vi "Lambda_Test_RT.vi"() -> ()   [LabVIEW 2014]
uses:
  <vilib>/rvi/interface/nirviOpenFPGA/nirviOpenFPGA.xnode
  <vilib>/rvi/interface/nirviReadWriteControl/nirviReadWriteControl.xnode
  <vilib>/Platform/TimedLoop/XDataNode/XDataNode.xnode
  <vilib>/Platform/TimedLoop/XDataNode/nitl_modes.ctl
  <vilib>/Platform/TimedLoop/XDataNode/XDNodeRunTimeDep.lvlib
  <vilib>/Platform/TimedLoop/XDataNode/wakeup.ctl
  <vilib>/Platform/TimedLoop/XDataNode/timing_clust.ctl
  <vilib>/addons/control/pid/NI_PID_pid.lvlib
  <vilib>/rvi/errors/niLvFpgaAdjustHostInterfaceError.vi
  <vilib>/rvi/interface/nirviCloseFPGA/nirviCloseFPGA.xnode
  <vilib>/addons/control/pid/pid.llb/PID (DBL).vi
  NiFpgaLv.dll
  <vilib>/Utility/error.llb/Error Cluster From Error Code.vi
  FPGA main v06-01.vi
  FPGA Bitfiles/MAXCAT_FPGATarget5_FPGAmainv06-01_qYdUsd75oPc.lvbitx
  FPGA 9146 v160610.vi
  <vilib>/FPGAPlugInAG/cRIO-9067/niLvFpga_Open_cRIO-9067.vi
  <vilib>/FPGAPlugInAG/cRIO-9067/niLvFpga_Close_cRIO-9067.vi
panel:
  in  "HC Fact HCLO":dbl
  in  "HC Base HCLO":dbl
  in  "O2 Base HCLO":dbl
  in  "O2 Fact HCLO":dbl
  in  "Heat Load Control":T1(radio)
  in  "Reset Heat Load 4":bool
  out "% Complete 4":dbl
  out "Complete 4":dbl(slide) scale=0.0..100.0
  out "Remaining Time 4":dbl format="%<%H:%M:%S>t"
  out "Ageing Time 4":dbl format="%<%H:%M:%S>t"
  in  "Reset Heat Load 3":bool
  out "% Complete 3":dbl
  out "Complete 3":dbl(slide) scale=0.0..100.0
  out "Remaining Time 3":dbl format="%<%H:%M:%S>t"
  out "Ageing Time 3":dbl format="%<%H:%M:%S>t"
  out "UEGO Array":dbl[](array[numeric])
  in  "UEGO 3":i64=200
  out "UEGO Sensor Results 2":T2
  in  "SensorControl 2":T3={"UEGO1Enable"=FALSE, "UEGO2Enable"=FALSE, "EGO1Enable"=FALSE, "EGO2Enable"=FALSE, "EGO3Enable"=FALSE, "EGO4Enable"=FALSE, "UEGO1Range"=FALSE, "UEGO2Range"=FALSE, "FilterCutoff (Hz)"=10.0}
  in  "UEGO Back Pressure (bar) 3":T4={"UEGO1BackPressure (bar)"=1.013, "UEGO2BackPressure (bar)"=1.013}
  in  "UEGOModuleEnable 3":bool
  out "UEGO Heater (V) 2":T5
  out "UEGO Diagnostics 3":T6={"ModulePresent"=FALSE, "UEGO1SensorFault"=63, "UEGO2SensorFault"=63, "UEGO1HeaterFault"=192, "UEGO2HeaterFault"=192, "UEGOFuseStatus"=0, "Battery (V)"=0.0, "LSUType"=0} {"LSUType" items=["LSU 4.9", "LSU 4.2"]; "UEGOFuseStatus" items=["FUSE OK", "FUSE BLOWN"]; "UEGO2SensorFault" items=["NO FAULT"=63, "SHORT TO GND OR BATT"=0]; "UEGO2HeaterFault" items=["SHORT TO GROUND"=0, "OPEN CIRCUIT"=64, "SHORT TO BATTERY"=128, "NO FAULT"=192]; "UEGO1SensorFault" items=["NO FAULT"=63, "SHORT TO GND OR BATT"=0]; "UEGO1HeaterFault" items=["SHORT TO GROUND"=0, "OPEN CIRCUIT"=64, "SHORT TO BATTERY"=128, "NO FAULT"=192]}
  out "UEGO Temperature (C) 2":T7
  in  "Start Test":bool
  out "Ready":bool
  out "UEGO Sensor Results":T2
  in  "SensorControl":T3={"UEGO1Enable"=FALSE, "UEGO2Enable"=FALSE, "EGO1Enable"=FALSE, "EGO2Enable"=FALSE, "EGO3Enable"=FALSE, "EGO4Enable"=FALSE, "UEGO1Range"=FALSE, "UEGO2Range"=FALSE, "FilterCutoff (Hz)"=10.0}
  in  "UEGO Back Pressure (bar)":T4={"UEGO1BackPressure (bar)"=1.013, "UEGO2BackPressure (bar)"=1.013}
  in  "UEGOModuleEnable":bool
  out "UEGO Heater (V)":T5
  out "UEGO Diagnostics":T6={"ModulePresent"=FALSE, "UEGO1SensorFault"=63, "UEGO2SensorFault"=63, "UEGO1HeaterFault"=192, "UEGO2HeaterFault"=192, "UEGOFuseStatus"=0, "Battery (V)"=0.0, "LSUType"=0} {"LSUType" items=["LSU 4.9", "LSU 4.2"]; "UEGOFuseStatus" items=["FUSE OK", "FUSE BLOWN"]; "UEGO2SensorFault" items=["NO FAULT"=63, "SHORT TO GND OR BATT"=0]; "UEGO2HeaterFault" items=["SHORT TO GROUND"=0, "OPEN CIRCUIT"=64, "SHORT TO BATTERY"=128, "NO FAULT"=192]; "UEGO1SensorFault" items=["NO FAULT"=63, "SHORT TO GND OR BATT"=0]; "UEGO1HeaterFault" items=["SHORT TO GROUND"=0, "OPEN CIRCUIT"=64, "SHORT TO BATTERY"=128, "NO FAULT"=192]}
  out "UEGO Temperature (C)":T7
  in  "Reset Heat Load 2":bool
  out "% Complete 2":dbl
  out "Complete 2":dbl(slide) scale=0.0..100.0
  out "Remaining Time 2":dbl format="%<%H:%M:%S>t"
  out "Ageing Time 2":dbl format="%<%H:%M:%S>t"
  in  "Pressure Transducer 2":enum32{"Druck ", "FUJI ", "Impress"}(radio)
  in  "Pressure Transducer 1":enum32{"Druck ", "FUJI ", "Impress"}(radio)
  out "UEGO Diagnostics 2":T8={"ModulePresent"=FALSE, "UEGO1SensorFault"=63, "UEGO2SensorFault"=63, "UEGO1HeaterFault"=192, "UEGO2HeaterFault"=192, "UEGOFuseStatus"=0, "Battery (V)"=0.0} {"UEGOFuseStatus" items=["FUSE OK", "FUSE BLOWN"]; "UEGO2SensorFault" items=["NO FAULT"=63, "SHORT TO GND OR BATT"=0]; "UEGO2HeaterFault" items=["SHORT TO GROUND"=0, "OPEN CIRCUIT"=64, "SHORT TO BATTERY"=128, "NO FAULT"=192]; "UEGO1SensorFault" items=["NO FAULT"=63, "SHORT TO GND OR BATT"=0]; "UEGO1HeaterFault" items=["SHORT TO GROUND"=0, "OPEN CIRCUIT"=64, "SHORT TO BATTERY"=128, "NO FAULT"=192]}
  in  "V Max Flow":sgl=10.0 format="%.3f"
  out "Press Time":i32
  out "Valve 2 Position":dbl
  out "Valve 1 Position":dbl
  in  "Valve 2 SP":dbl=1.0
  in  "Valve 1 SP":dbl=1.0
  out "Uego Avg":dbl
  in  "Press Up Limit":sgl=5.0
  in  "Press Low Limit":sgl
  out "Loop No.":i32
  in  "UEGO 1":i64=200
  in  "UEGO 2":i64=200
  in  "UEGOModuleEnable 2":bool=TRUE
  in  "UEGO Back Pressure (bar) 2":T4={"UEGO1BackPressure (bar)"=1.013, "UEGO2BackPressure (bar)"=1.013}
  in  "SensorEnable 2":T9={"UEGO1Enable"=TRUE, "UEGO2Enable"=TRUE, "EGO1Enable"=TRUE, "EGO2Enable"=TRUE, "EGO3Enable"=TRUE, "EGO4Enable"=TRUE}
  out "UEGO Meas 2":T2
  out "Pressure":dbl(graph)
  out "HC-2":bool
  out "AIR-2":bool
  out "HC-B":bool
  out "AIR-B":bool
  out "NO":bool
  out "AIR-1":bool
  out "HC-1":bool
  out "CO":bool
  in  "NO Factor":dbl
  in  "CO Factor":dbl
  in  "Set-point Fan":dbl
  in  "Fan PID":bool
  in  "Furnace 1":dbl=2.0
  in  "Furnace 2":dbl=2.0
  in  "Furnace Manual Mode":bool
  in  "Reset Heat Load":bool
  in  "Mop-up Lambda Control":bool
  in  "Lambda SP 3":dbl
  in  "Output Low 3":dbl
  in  "Output High 3":dbl
  in  "PID Mop-up Catalyst":T10={"proportional gain (Kc)"=0.8, "integral time (Ti, min)"=0.8, "derivative time (Td, min)"=0.0}
  in  "PID Catalyst 2":T10={"proportional gain (Kc)"=0.8, "integral time (Ti, min)"=0.8, "derivative time (Td, min)"=0.0}
  in  "PID Catalyst 1":T10={"proportional gain (Kc)"=0.8, "integral time (Ti, min)"=0.8, "derivative time (Td, min)"=0.0}
  in  "NO PID Light-Off":T10={"proportional gain (Kc)"=1.0, "integral time (Ti, min)"=0.0, "derivative time (Td, min)"=0.0}
  in  "NO PID Sweep Test":T10={"proportional gain (Kc)"=1.0, "integral time (Ti, min)"=0.0, "derivative time (Td, min)"=0.0}
  in  "H2O":dbl
  in  "SO2":dbl
  in  "N2":dbl
  in  "CO2":dbl
  in  "NO":dbl format="%#_13g"
  in  "CO":dbl format="%#_13g"
  out "% Complete":dbl
  out "Complete":dbl(slide) scale=0.0..100.0
  out "Remaining Time":dbl format="%<%H:%M:%S>t"
  out "Ageing Time":dbl format="%<%H:%M:%S>t"
  in  "Furnace Open Loop":bool
  in  "Furnace 2 Baseline":dbl=2.0
  in  "BED TARGET 2":dbl=2.0
  in  "PID Furnace 1":T10={"proportional gain (Kc)"=1.0, "integral time (Ti, min)"=0.0, "derivative time (Td, min)"=0.0}
  in  "Lambda SP 2":dbl
  in  "Furnace 1 Baseline":dbl=2.0
  in  "Counter Interval 2":i32
  in  "Counter Interval 1":i32
  in  "ECM Lambda Control":bool
  out "ECM 1":dbl
  out "ECM 2":dbl
  in  "Lambda SP":dbl
  in  "Output Low 2":dbl
  in  "Output High 2":dbl
  out "Tank Pressure":dbl
  out "Rapidox":dbl
  out "Inlet Temp":sgl
  out "MFC SV Array":bool[](array[boolean])
  out "Cycle Length":i32
  in  "HC Cyc 2":dbl format="%#_13g"
  in  "HC Bal":dbl format="%#_13g"
  in  "Air Cyc 1":dbl format="%#_13g"
  in  "Air Cyc 2":dbl format="%#_13g"
  in  "Air Bal":dbl format="%#_13g"
  in  "HC Cyc 1":dbl format="%#_13g"
  in  "Furnace 2":sgl=10.0
  in  "Furnace 1":sgl=10.0
  in  "Air Cyc 2 Factor":dbl
  in  "Air Cyc 1 Factor":dbl
  in  "HC Cyc 2 Factor":dbl
  in  "HC Bal Factor":dbl
  in  "Air Bal Factor":dbl
  in  "HC Cyc1 Factor":dbl
  in  "NOxLambda Control":bool
  in  "Furnace Control VI":bool
  out "UEGO 1 Cat":dbl(graph)
  out "UEGO 1 Fur":sgl(graph)
  in  "O2 Low Limit":sgl
  in  "O2 Up Limit":sgl=5.0
  out "Flow 2":dbl
  out "Flow 1":dbl
  out "Test Start":i32
  out "Control Variables":dbl[](array[numeric])
  out "Iteration \nDuration 3":i64
  in  "Output High 1":dbl
  in  "Output Low 1":dbl
  in  "NO Base NOLO":dbl
  in  "NO Factor NOLO":dbl
  in  "CO Base NOLO":dbl
  in  "CO Factor NOLO":dbl
  in  "CO Base COLO":dbl
  in  "O2 Base COLO":dbl
  in  "CO Fact COLO":dbl
  in  "O2 Fact COLO":dbl
  in  "NO Furnace Inlet":dbl=5.0
  in  "CO Furnace Inlet":dbl=5.0
  in  "SW Furnace Inlet":dbl=5.0
  in  "HC Furnace Inlet":dbl=0.2
  in  "Sw time":dbl
  in  "N2 Age":dbl
  in  "HC INJ CONTROL":i32
  in  "Age Furnace Inlet":dbl=5.0
  in  "BED TARGET":dbl=2.0
  in  "Age Rap Lim":dbl=5.0
  in  "SW rap lim":dbl=5.0
  in  "CO Rap Lim":dbl=5.0
  in  "NO Rap Lim":dbl=5.0
  in  "Fan Speed V":dbl
  in  "HC rap lim":dbl=0.2
  in  "STOP":bool
  in  "TankLo":dbl=1.5
  in  "TankHi":dbl=2.0
  out "DI no1":u32
  in  "PID Furnace 2":T10={"proportional gain (Kc)"=1.0, "integral time (Ti, min)"=0.0, "derivative time (Td, min)"=0.0}
  in  "PID Inverter":T10={"proportional gain (Kc)"=0.8, "integral time (Ti, min)"=0.8, "derivative time (Td, min)"=0.0}
  out "Iteration Duration 2":i64
  out "error out":errorcluster
  # "Heat Load 1"
  # "Heat Load 1"
  # "Loop Readings"
  # "Pressure Release Limits"
  # "Pressure Alarm"
  # "MFC Alarms"
  # "kPa"
  # "kPa"
  # "Leak Limits"
  # "Warm-up"
  # "Rapidox Limit"
  # "Furnace Limit"
  # "Fan Control"
  # "Heat Load 2"
  # "Heat Load 2"
  # "Readings"
  # "Test Mode"
  # "Lambda PID Control"
  # "Furnace Control"
  # "NO Light - off"
  # "HC Light - off"
  # "Ageing"
  # "CO Light - off"
  # "Catalyst 1"
  # "Catalyst 2"
  # "Mop-up Catalyst"
  # "UEGO Module 1"
  # "UEGO Module 2"
  # "UEGO Module 3"
  # "Furnace PID Control"
  # "Other PID Control"
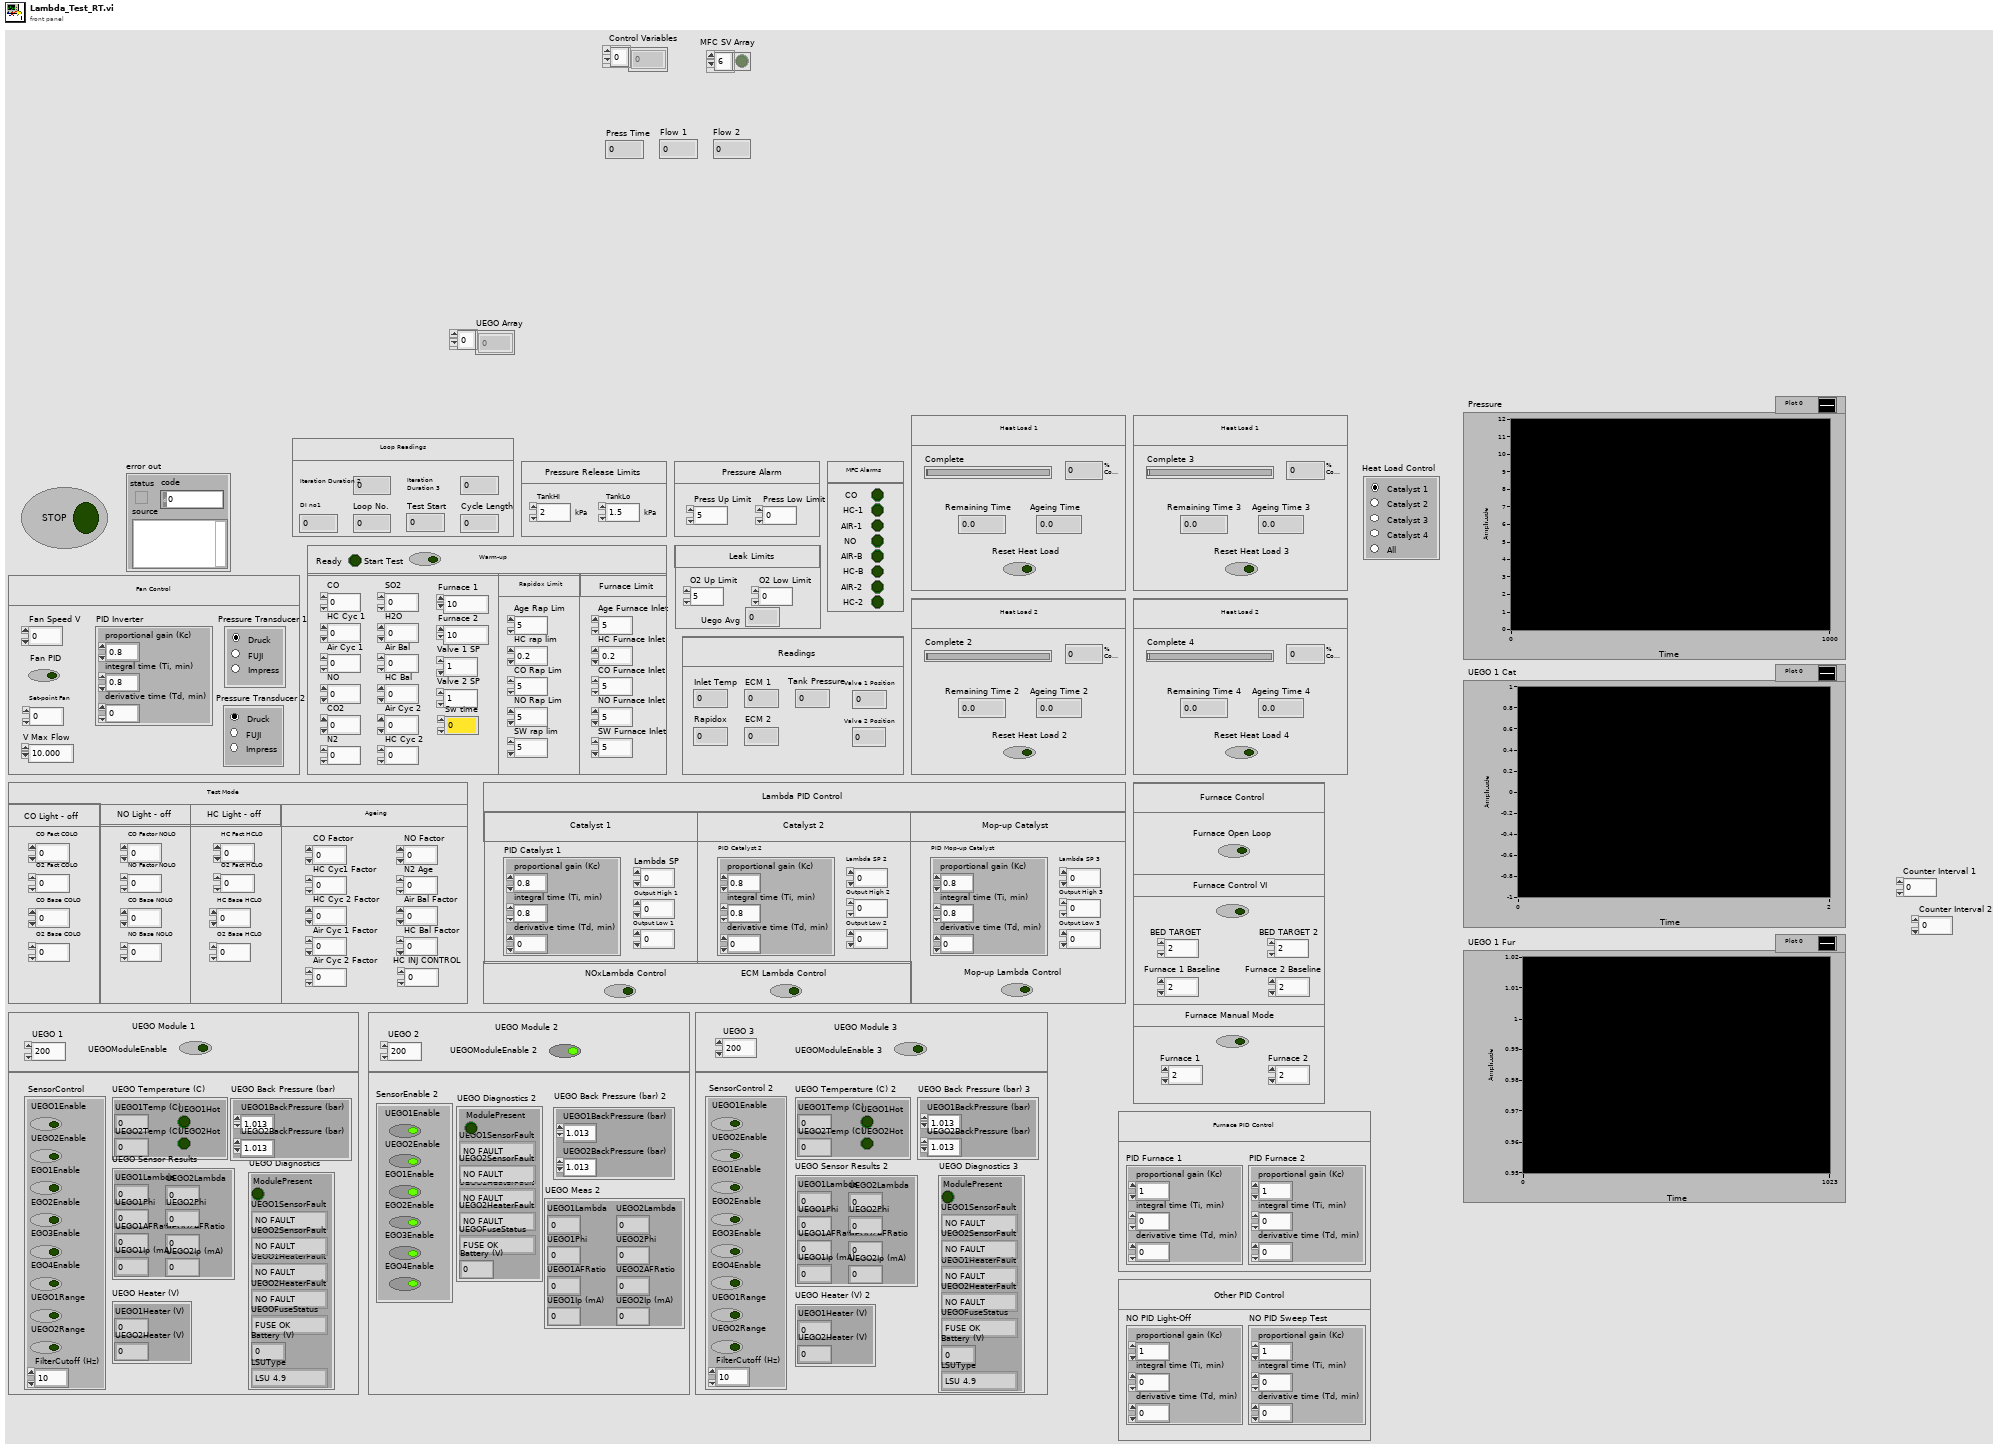
[diagram p1: front panel]
types:
  T1 = enum32{"Catalyst 1 ", "Catalyst 2 ", "Catalyst 3", "Catalyst 4", "All"}
  T2 = cluster{"UEGO1Lambda":sgl, "UEGO1Phi":sgl, "UEGO1AFRatio":sgl, "UEGO1Ip (mA)":sgl, "UEGO2Lambda":sgl, "UEGO2Phi":sgl, "UEGO2AFRatio":sgl, "UEGO2Ip (mA)":sgl}
  T3 = cluster{"UEGO1Enable":bool, "UEGO2Enable":bool, "EGO1Enable":bool, "EGO2Enable":bool, "EGO3Enable":bool, "EGO4Enable":bool, "UEGO1Range":bool, "UEGO2Range":bool, "FilterCutoff (Hz)":dbl}
  T4 = cluster{"UEGO1BackPressure (bar)":sgl, "UEGO2BackPressure (bar)":sgl}
  T5 = cluster{"UEGO1Heater (V)":sgl, "UEGO2Heater (V)":sgl}
  T6 = cluster{"ModulePresent":bool, "UEGO1SensorFault":u8, "UEGO2SensorFault":u8, "UEGO1HeaterFault":u8, "UEGO2HeaterFault":u8, "UEGOFuseStatus":u8, "Battery (V)":sgl, "LSUType":u8}
  T7 = cluster{"UEGO1Temp (C)":sgl, "UEGO2Temp (C)":sgl, "UEGO1Hot":bool, "UEGO2Hot":bool}
  T8 = cluster{"ModulePresent":bool, "UEGO1SensorFault":u8, "UEGO2SensorFault":u8, "UEGO1HeaterFault":u8, "UEGO2HeaterFault":u8, "UEGOFuseStatus":u8, "Battery (V)":sgl}
  T9 = cluster{"UEGO1Enable":bool, "UEGO2Enable":bool, "EGO1Enable":bool, "EGO2Enable":bool, "EGO3Enable":bool, "EGO4Enable":bool}
  T10 = cluster{"proportional gain (Kc)":dbl, "integral time (Ti, min)":dbl, "derivative time (Td, min)":dbl}
  T11 = typedef "XDNodeRunTimeDep.lvlib/timing_clust.ctl" = cluster{"Expected End [f-1]":u64, "Actual End [f-1]":u64, "Finished Late? [f-1]":bool, "Expected End [i-1]":u64, "Actual End [i-1]":u64, "Finished Late? [i-1]":bool, "Expected Start [i]":u64, "Actual Start [i]":u64, "Expected Start [f]":u64, "Actual Start [f]":u64, "Source Name":string, "Structure Name":string, "Period":i64, "Deadline":i64, "Offset":i64, "Start":i64, "Priority":i32, "Timeout":i32, "Mode":T12, "Wakeup Reason":T13, "Error":errorcluster, "Source Type":string, "Secondary Source Type":string, "Global End Time":u64, "Global Start Time":u64, "Frame Duration":u64, "Iteration Duration":u64, "Assigned CPU":i32, "I/O Scan Engine Mode":u32}
  T12 = typedef "XDNodeRunTimeDep.lvlib/nitl_modes.ctl" = enum32{"No Change", "Process missed periods, maintain original phase", "Discard missed periods, maintain original phase", "Process missed periods, ignore original phase", "Discard missed periods, ignore original phase"}
  T13 = typedef "XDNodeRunTimeDep.lvlib/wakeup.ctl" = enum32{"Normal", "Aborted", "Asynchronous wakeup", "Timing source error", "Timed loop error", "Timeout"}
  T14 = cluster{"Stoich A/F Ratio":sgl, "IpArray (mA)":sgl[], "LambdaArray":sgl[]}
  T15 = cluster{"UEGO1Diag":u8, "UEGO2Diag":u8, "UEGO1Sensor":u16, "UEGO2Sensor":u16, "UEGO1Heater":u16, "UEGO2Heater":u16, "UEGO1AmpOffset":u16, "UEGO2AmpOffset":u16, "UEGO1RIOffset":u16, "UEGO2RIOffset":u16, "UEGO1HeaterGain":u16, "UEGO2HeaterGain":u16, "Fuse":u16, "EGO1Sensor":u16, "EGO2Sensor":u16, "EGO3Sensor":u16, "EGO4Sensor":u16, "Battery":u16, "ModulePresent":bool, "UEGO1ID":u8, "UEGO2ID":u8, "LSUType":u8}
  T16 = cluster{"ModuleEnable":bool, "WatchdogIn":bool, "UEGO1Hot":bool, "UEGO2Hot":bool, "Cal1Request":bool, "Cal2Request":bool, "UEGOHeaterPeriod":u16, "UEGO1HeaterPulseWidth":u16, "UEGO2HeaterPulseWidth":u16, "UEGO1Range":bool, "UEGO2Range":bool, "LSUType (F=4.9,T=4.2)":bool}
  T17 = cluster{"UEGO1Diag":u8, "UEGO2Diag":u8, "UEGO1Sensor":i16, "UEGO2Sensor":i16, "UEGO1Heater":i16, "UEGO2Heater":i16, "UEGO1AmpOffset":i16, "UEGO2AmpOffset":i16, "UEGO1RIOffset":i16, "UEGO2RIOffset":i16, "UEGO1HeaterGain":i16, "UEGO2HeaterGain":i16, "Fuse":i16, "EGO1Sensor":i16, "EGO2Sensor":i16, "EGO3Sensor":i16, "EGO4Sensor":i16, "Battery":i16, "ModulePresent":bool, "UEGO1ID":u8, "UEGO2ID":u8}
  T18 = cluster{"ModuleEnable":bool, "WatchdogIn":bool, "UEGO1Hot":bool, "UEGO2Hot":bool, "Cal1Request":bool, "Cal2Request":bool, "UEGOHeaterPeriod":u16, "UEGO1HeaterPulseWidth":u16, "UEGO2HeaterPulseWidth":u16}
  T19 = cluster{"NOx (bits)":u16, "O2 (bits)":u16, "Sensor Supply Status":u8, "Sensor Temperature Status":u8, "NOx Signal Status":u8, "O2 Signal Status":u8, "Heater Mode Status":u8, "Heater Circuit Status":u8, "NOx Circuit Status":u8, "O2 Circuit Status":u8, "NOx Sensor Module Present":bool}
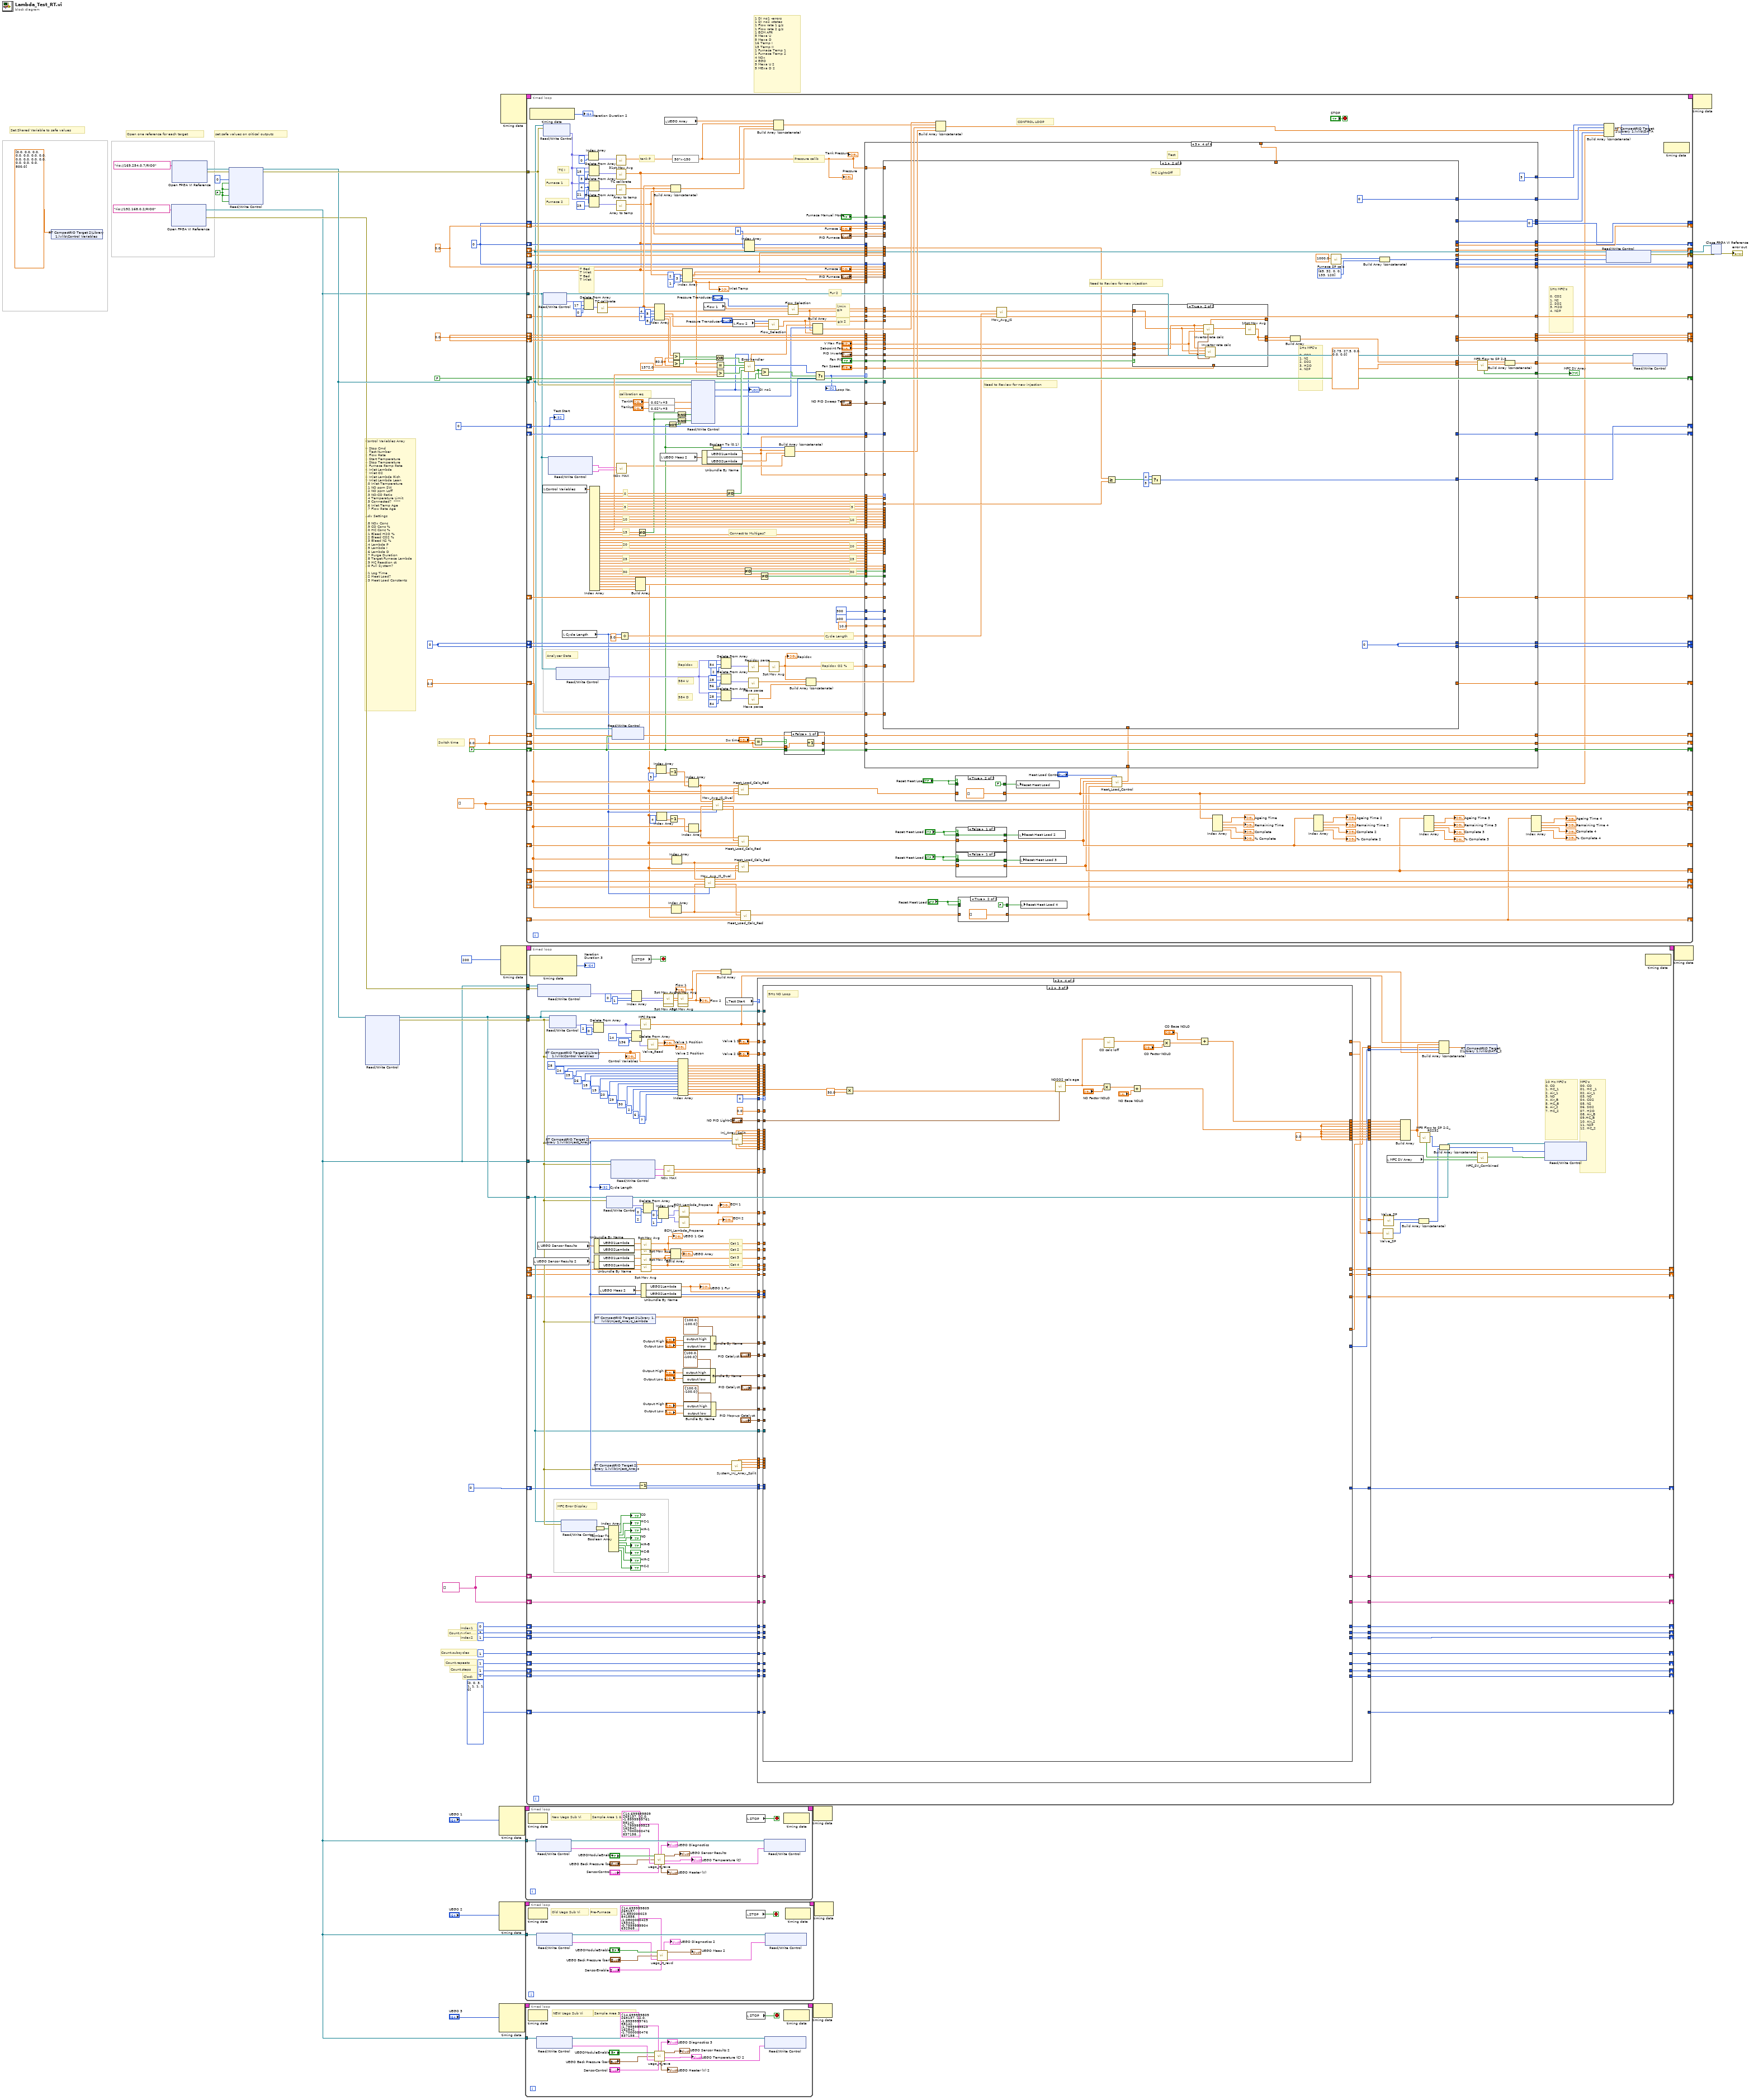
[diagram p0: block diagram]
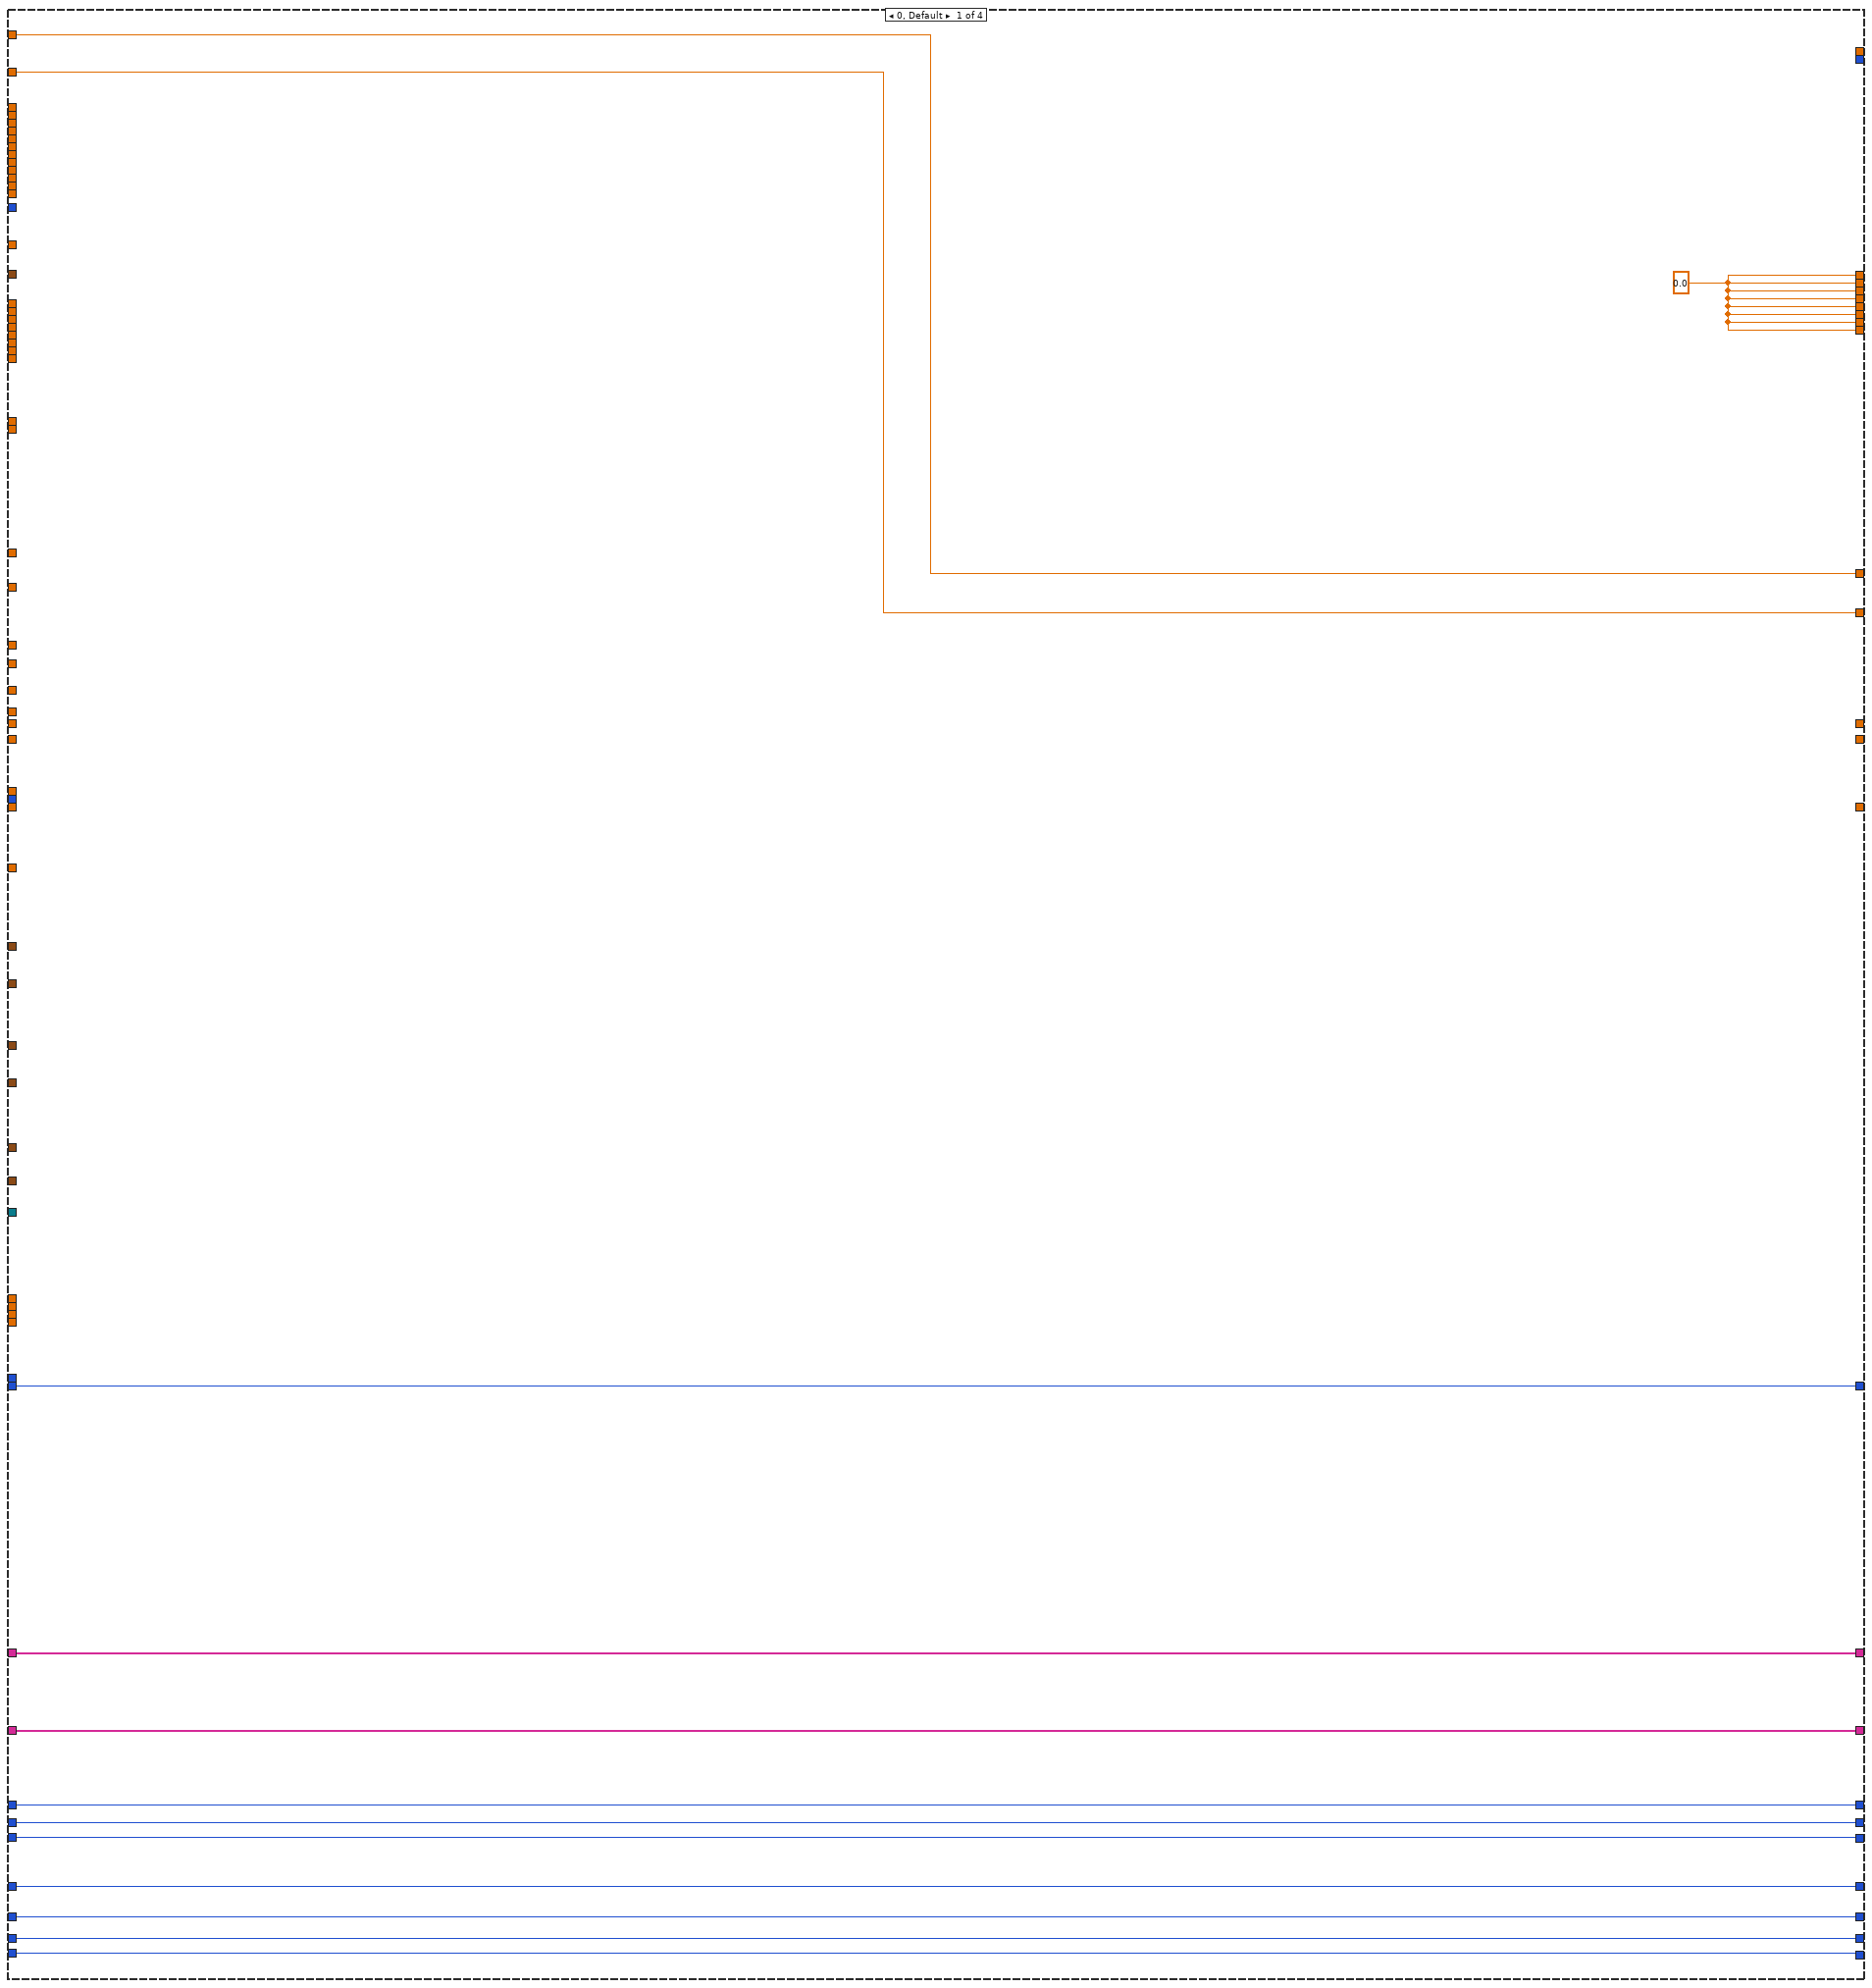
[diagram p2: hidden frame]
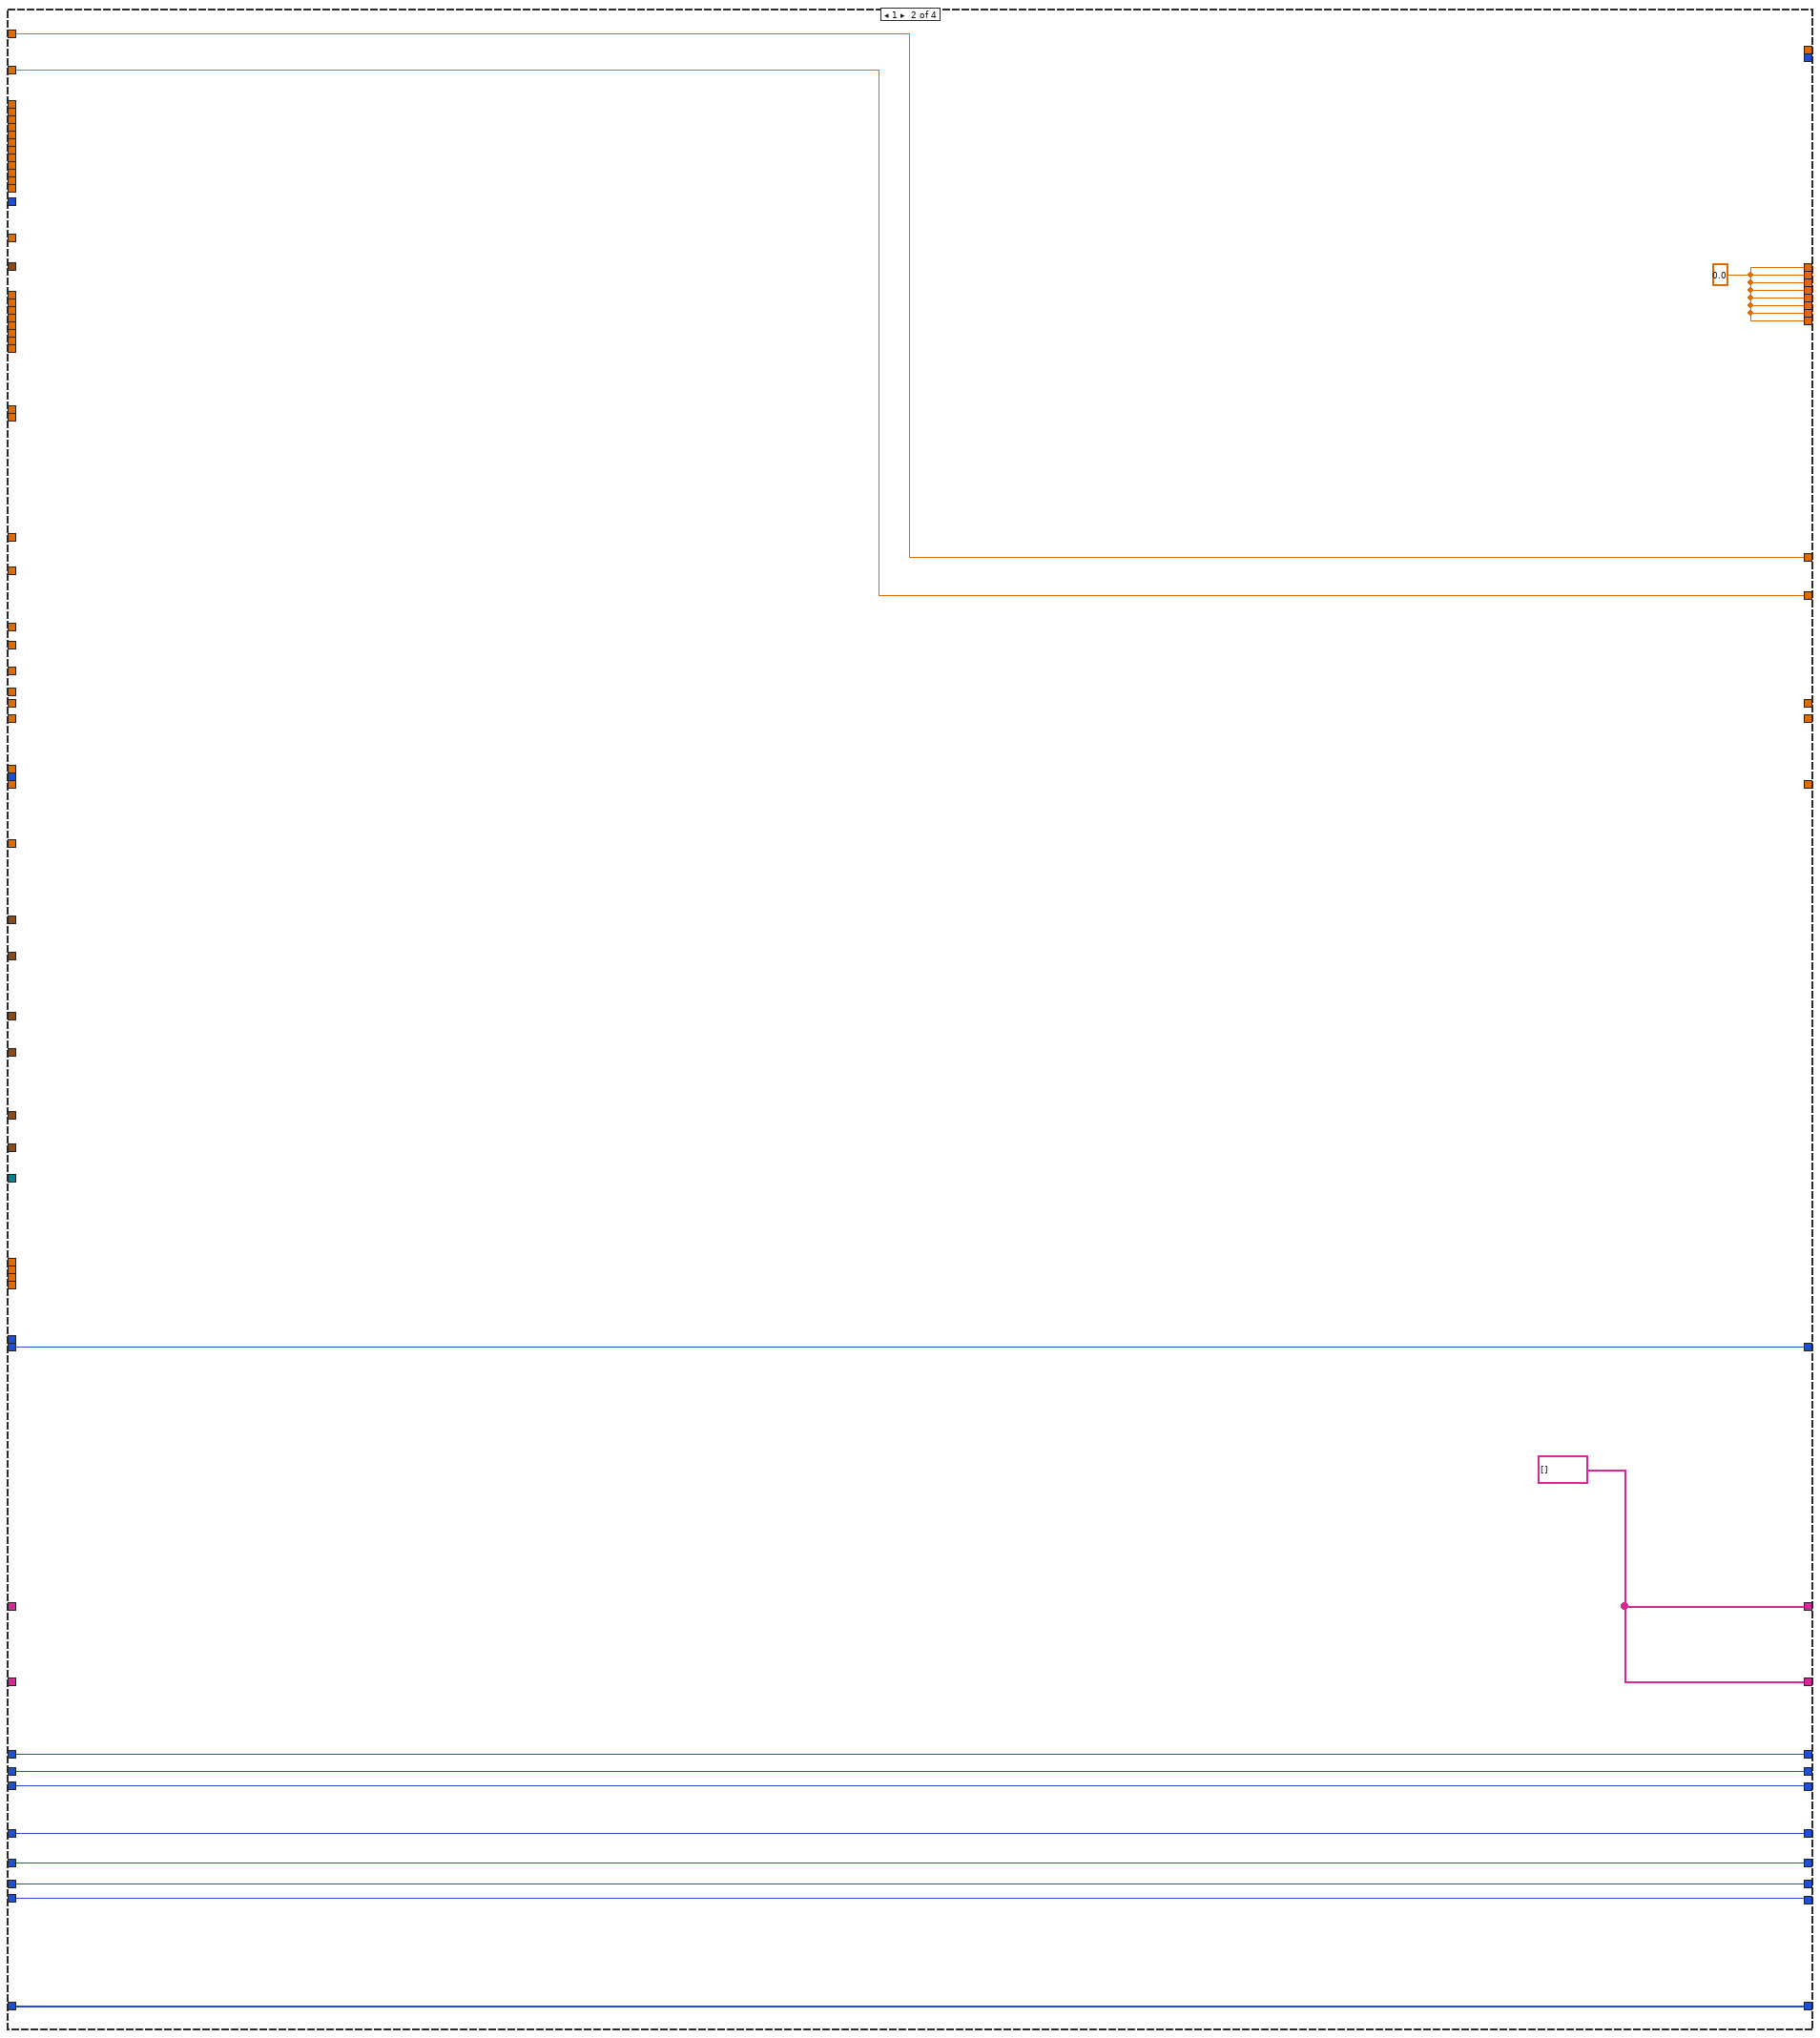
[diagram p3: hidden frame]
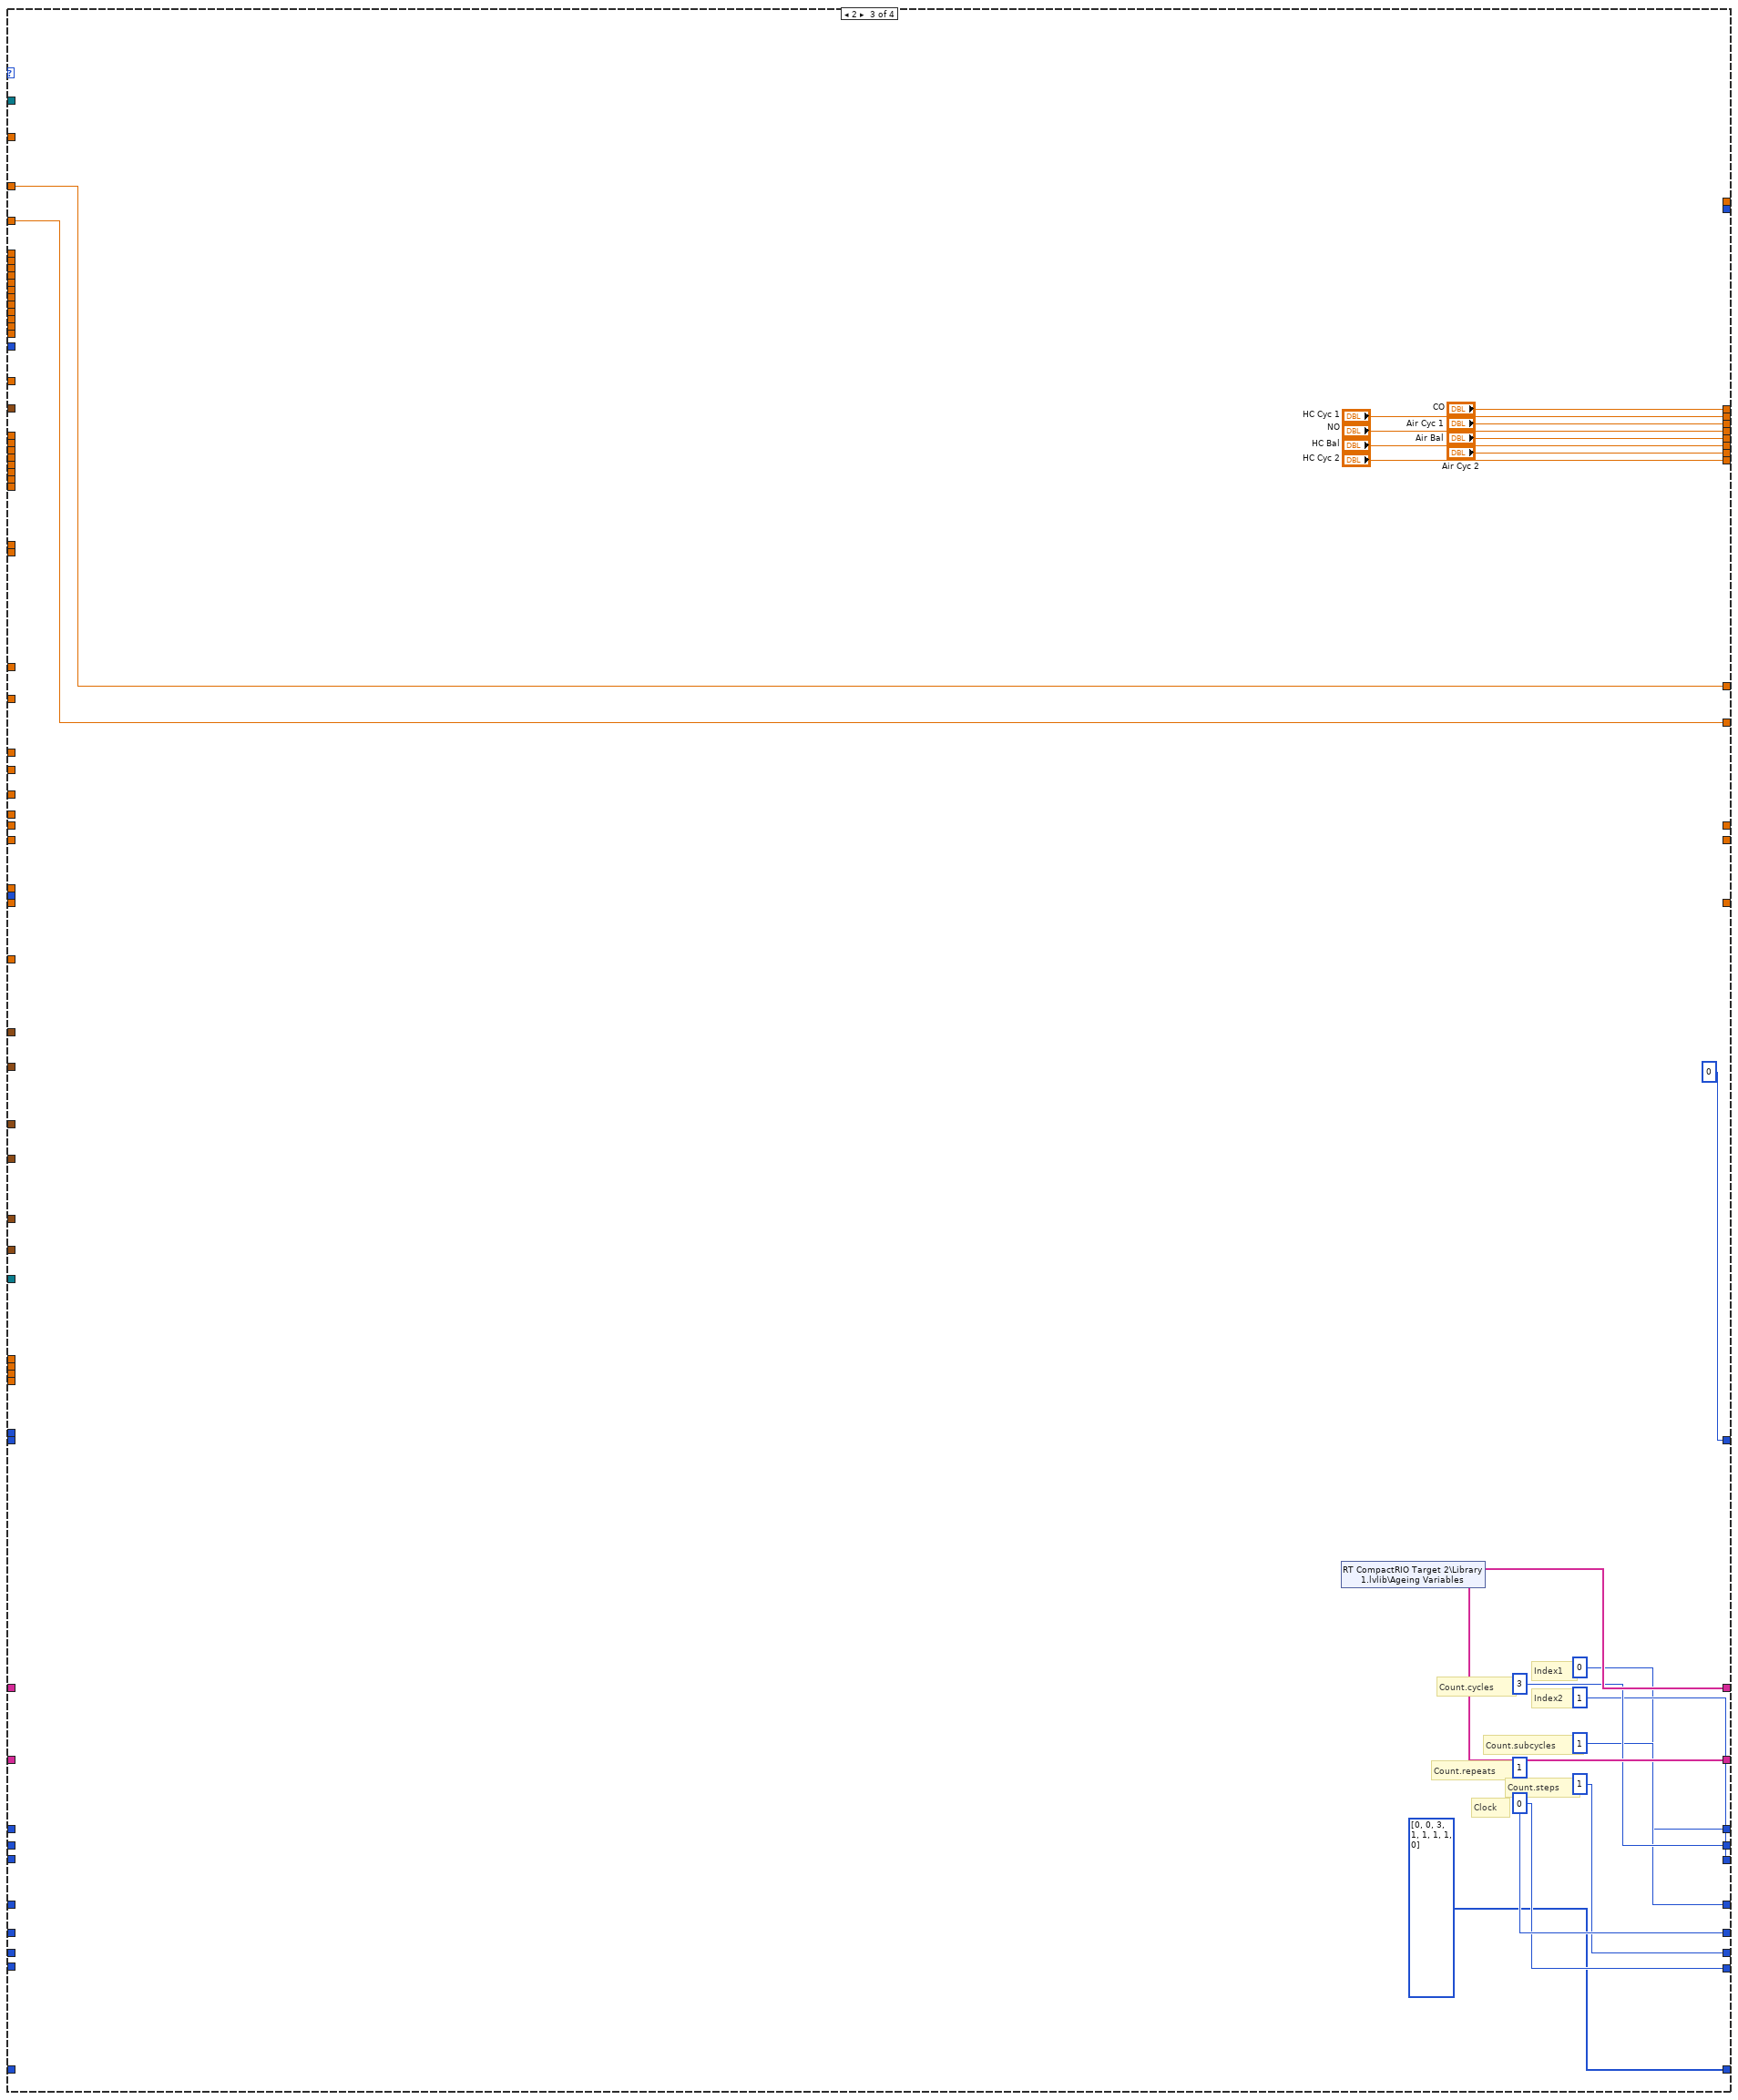
[diagram p4: hidden frame]
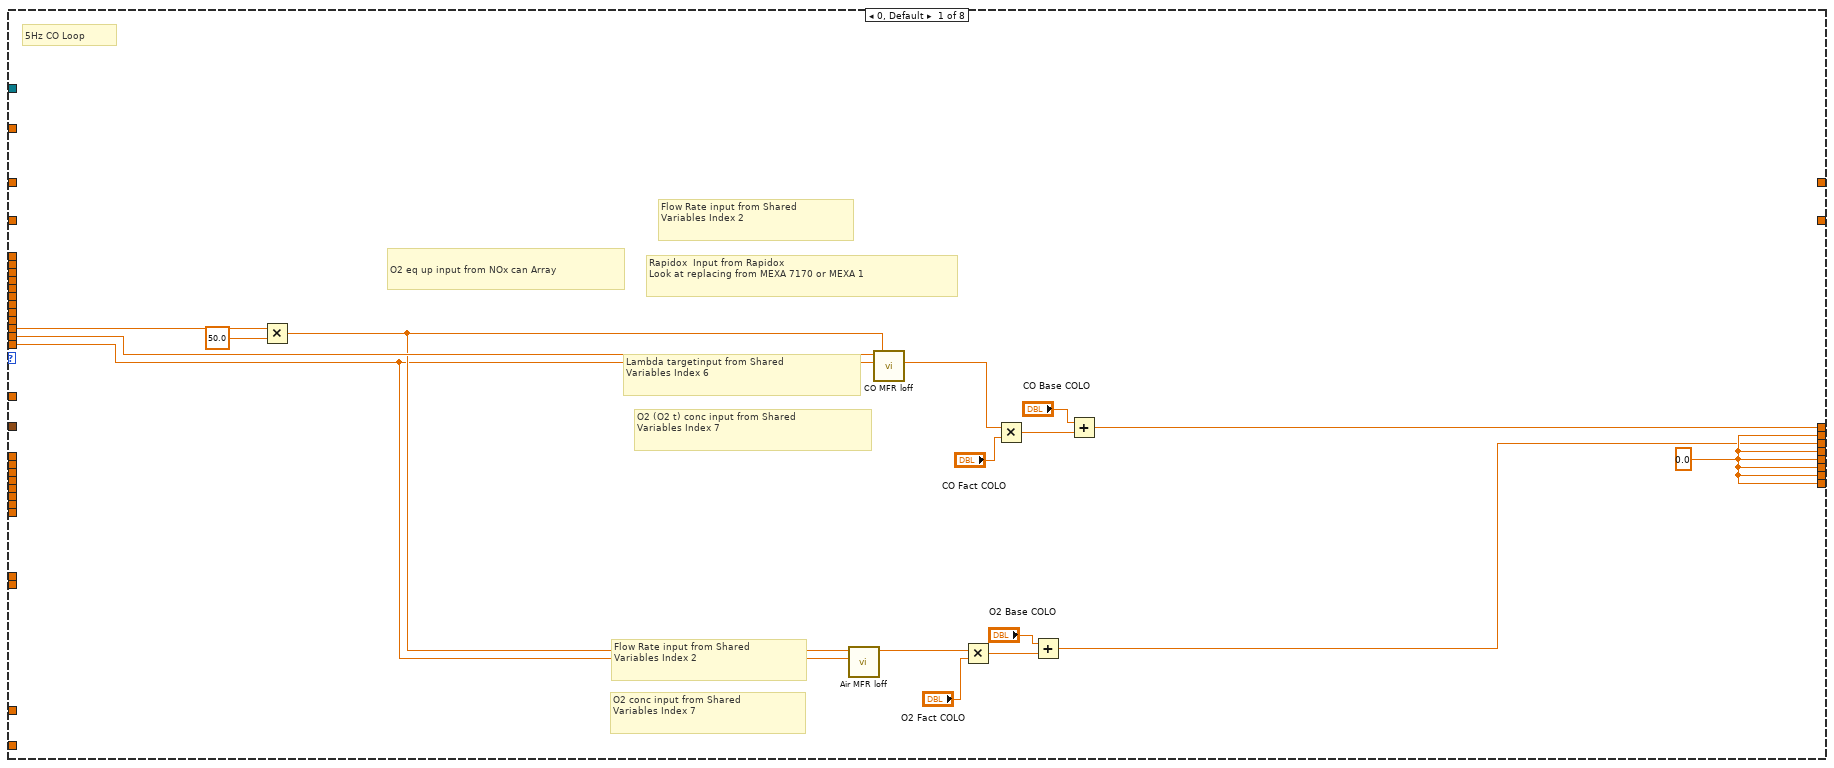
[diagram p5: hidden frame]
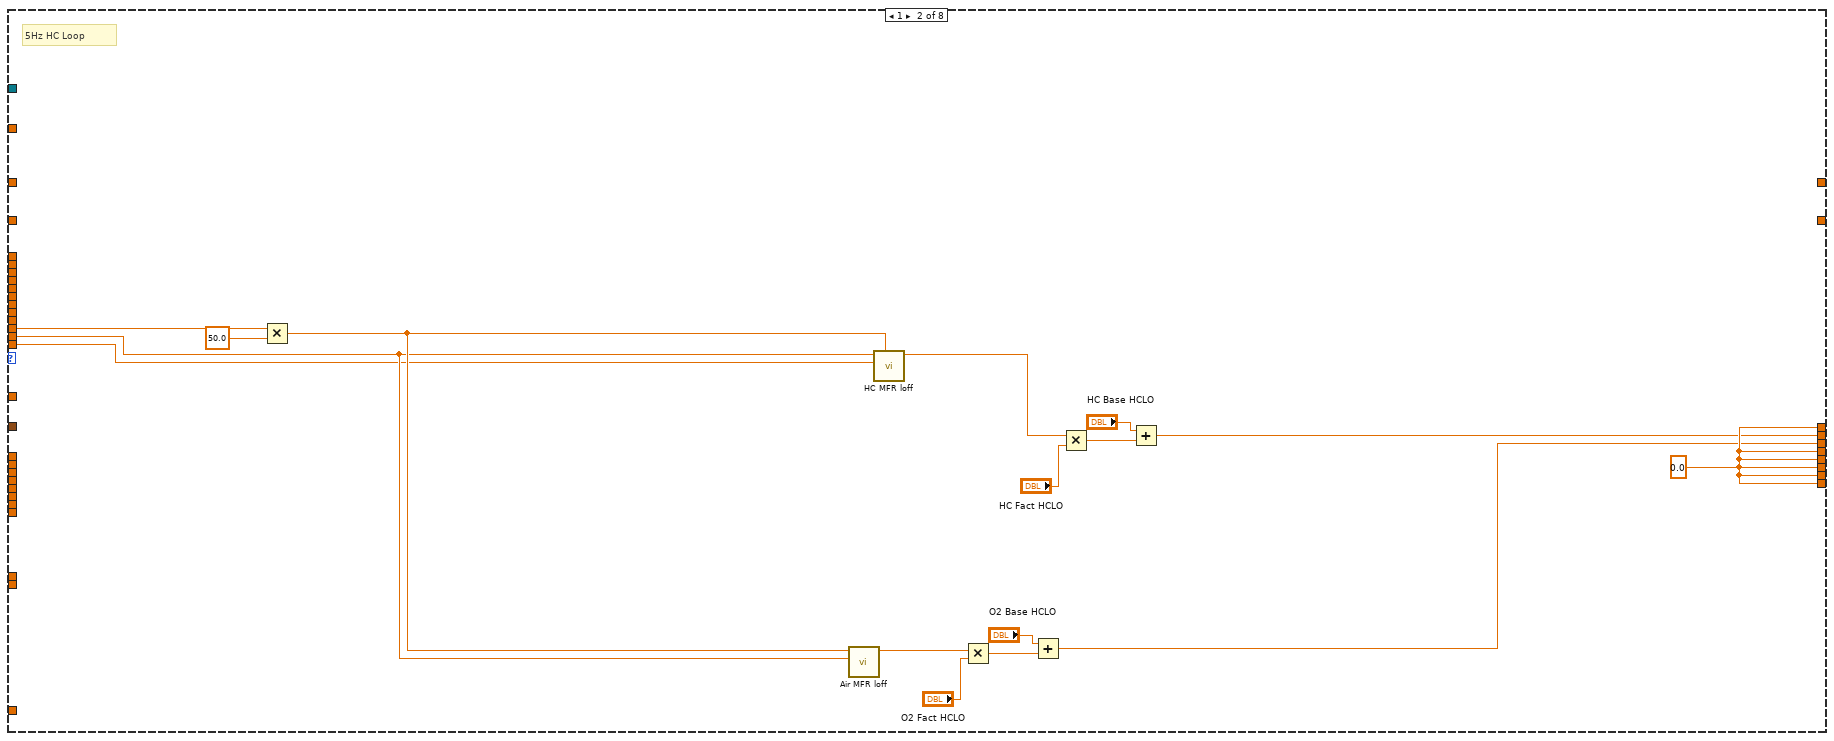
[diagram p6: hidden frame]
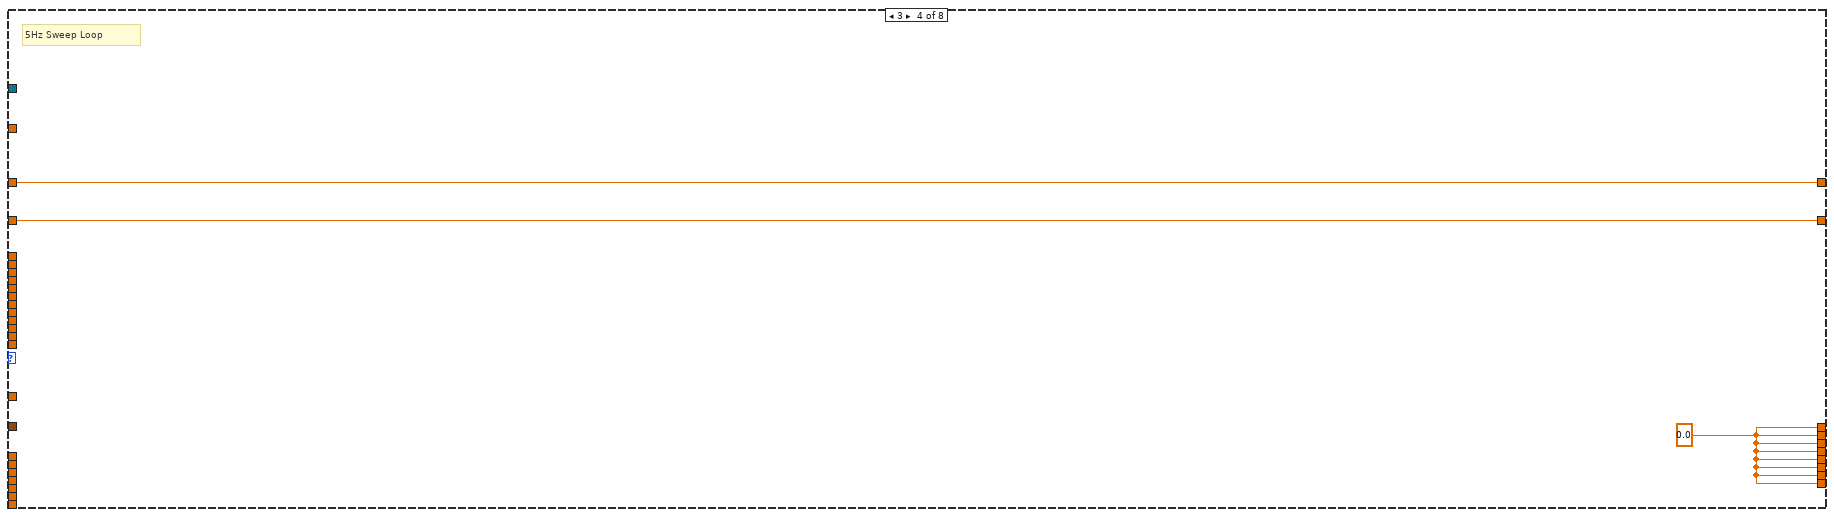
[diagram p7: hidden frame]
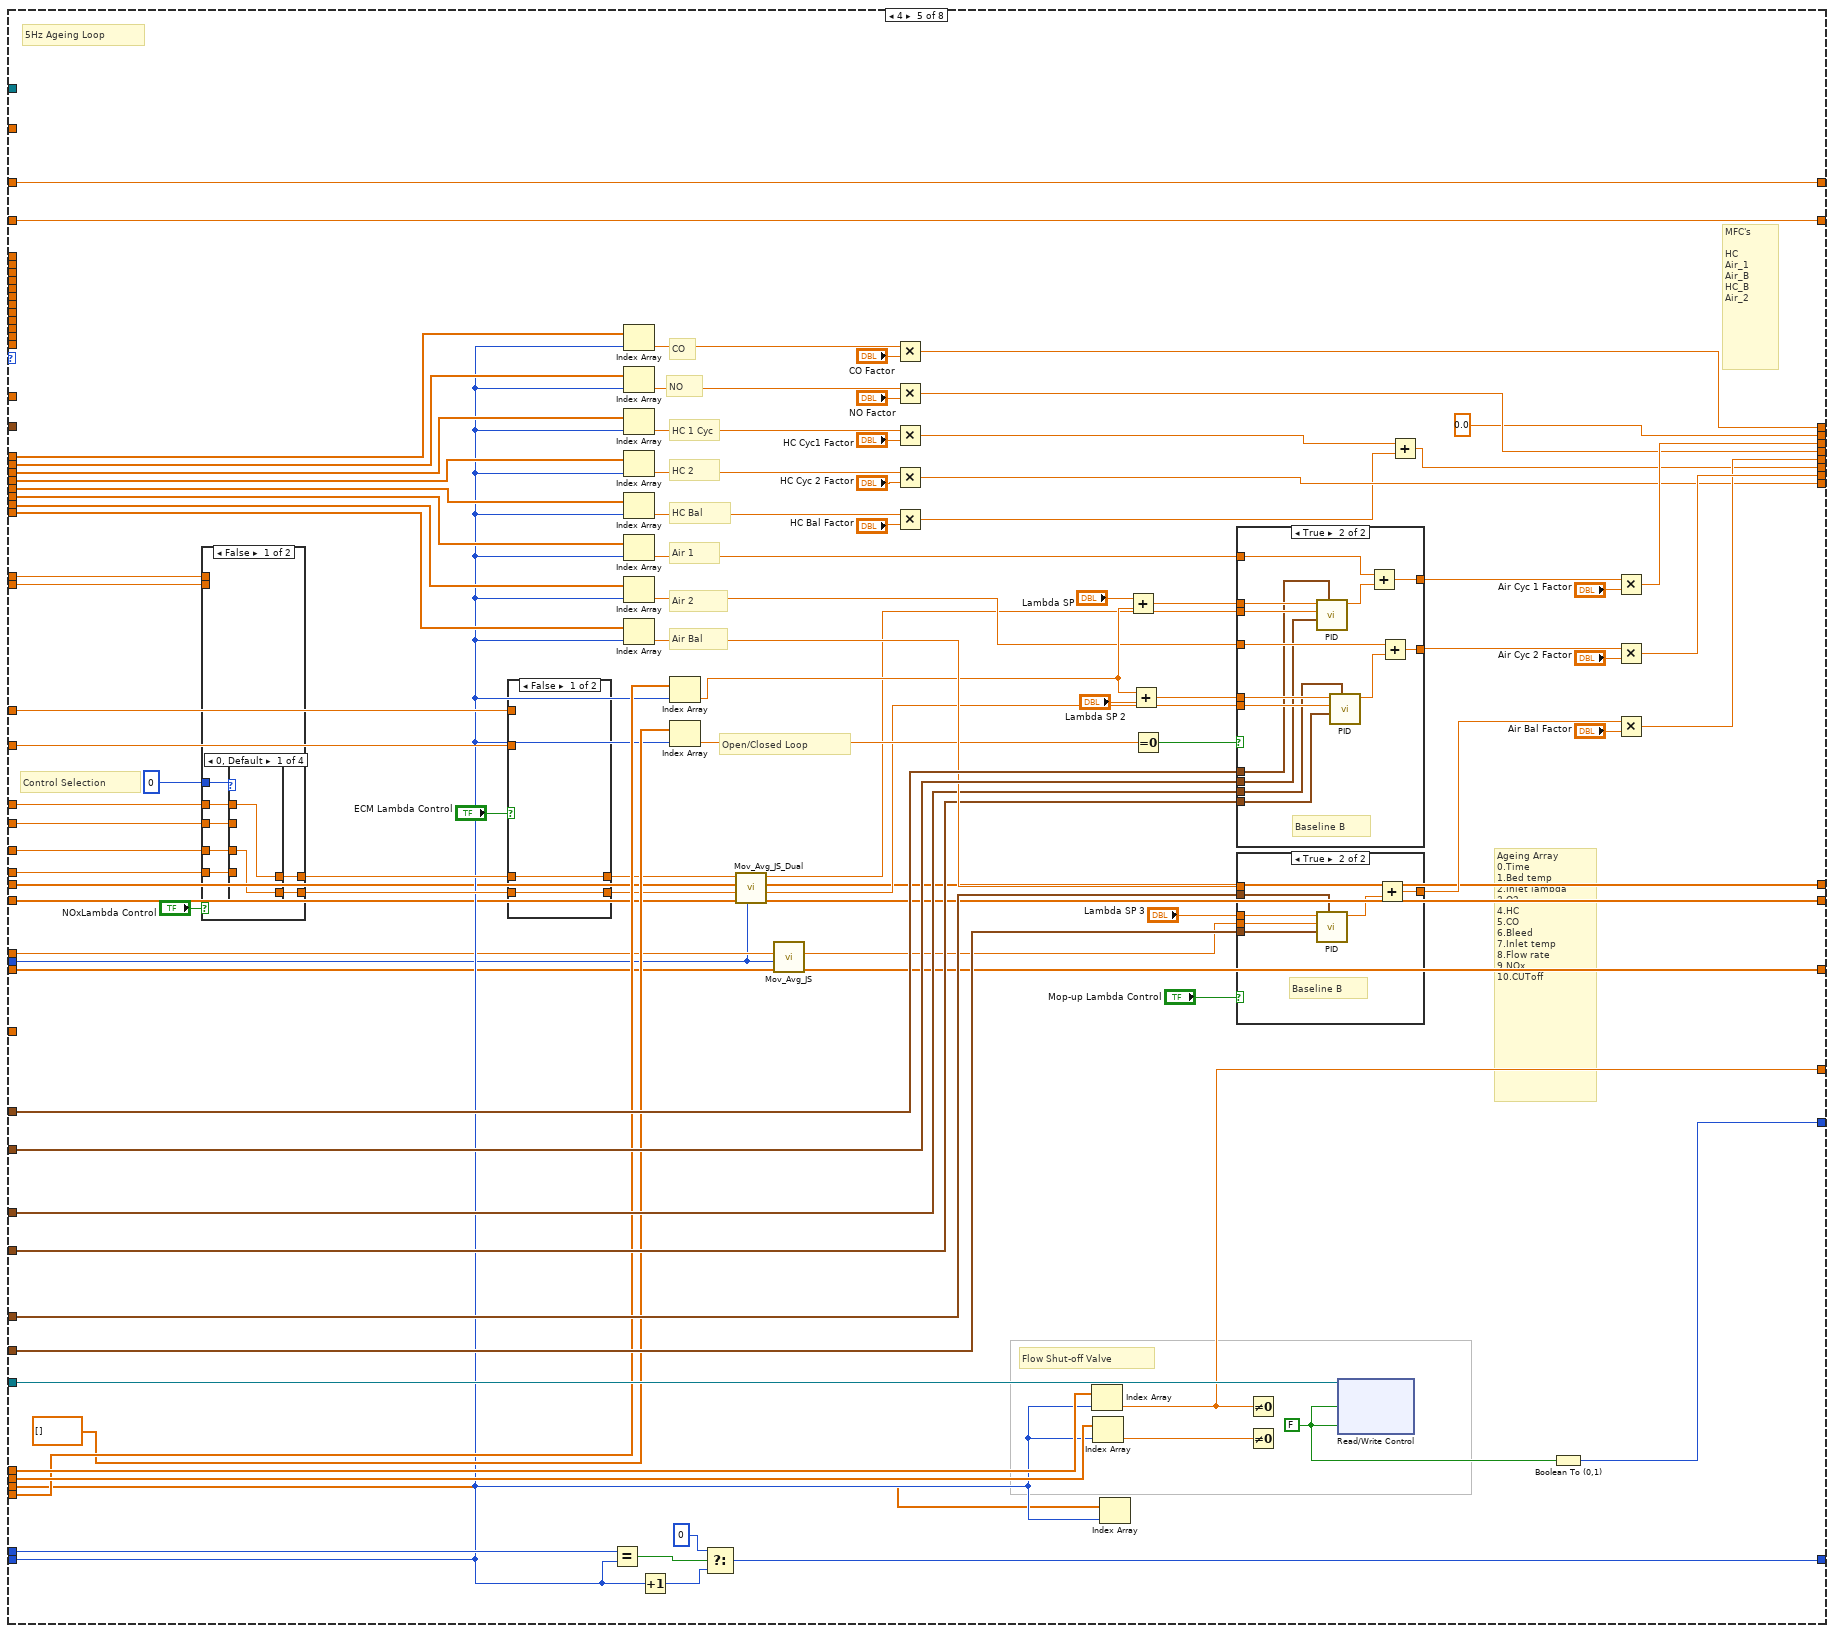
[diagram p8: hidden frame]
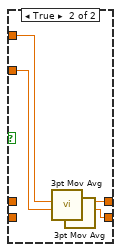
[diagram p10: hidden frame]
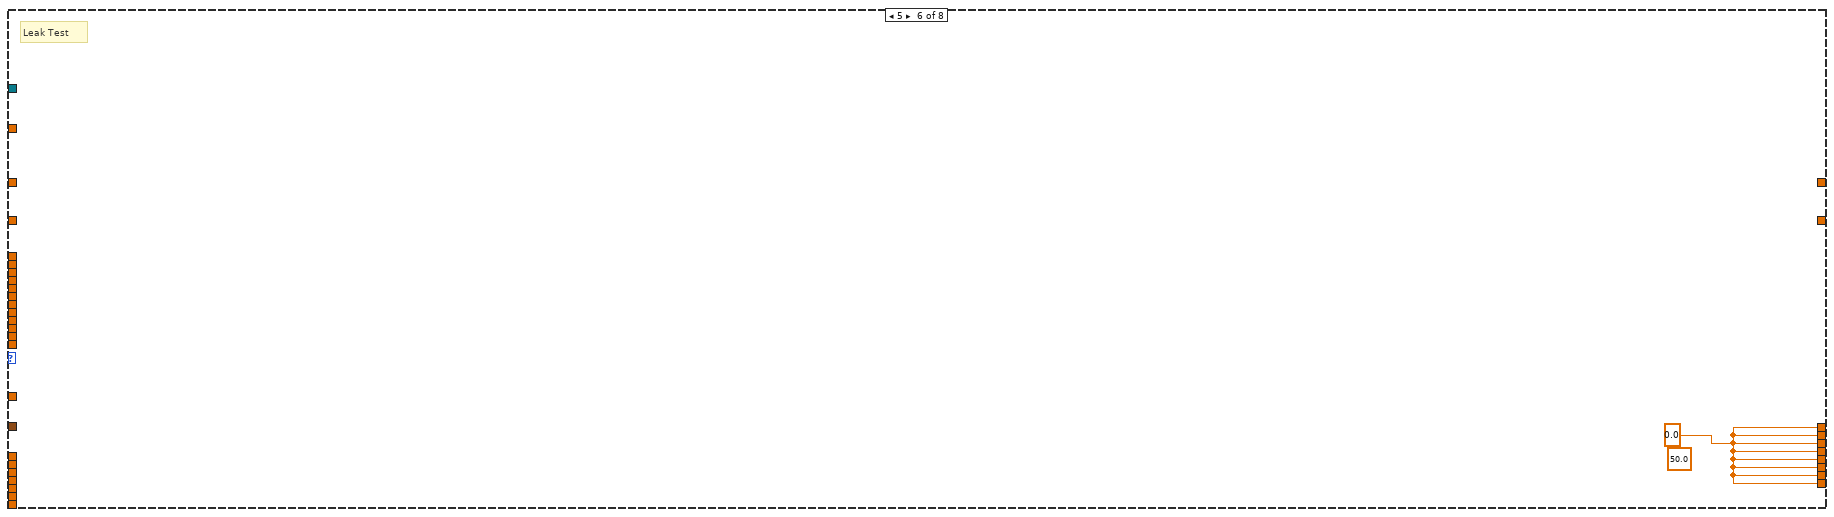
[diagram p16: hidden frame]
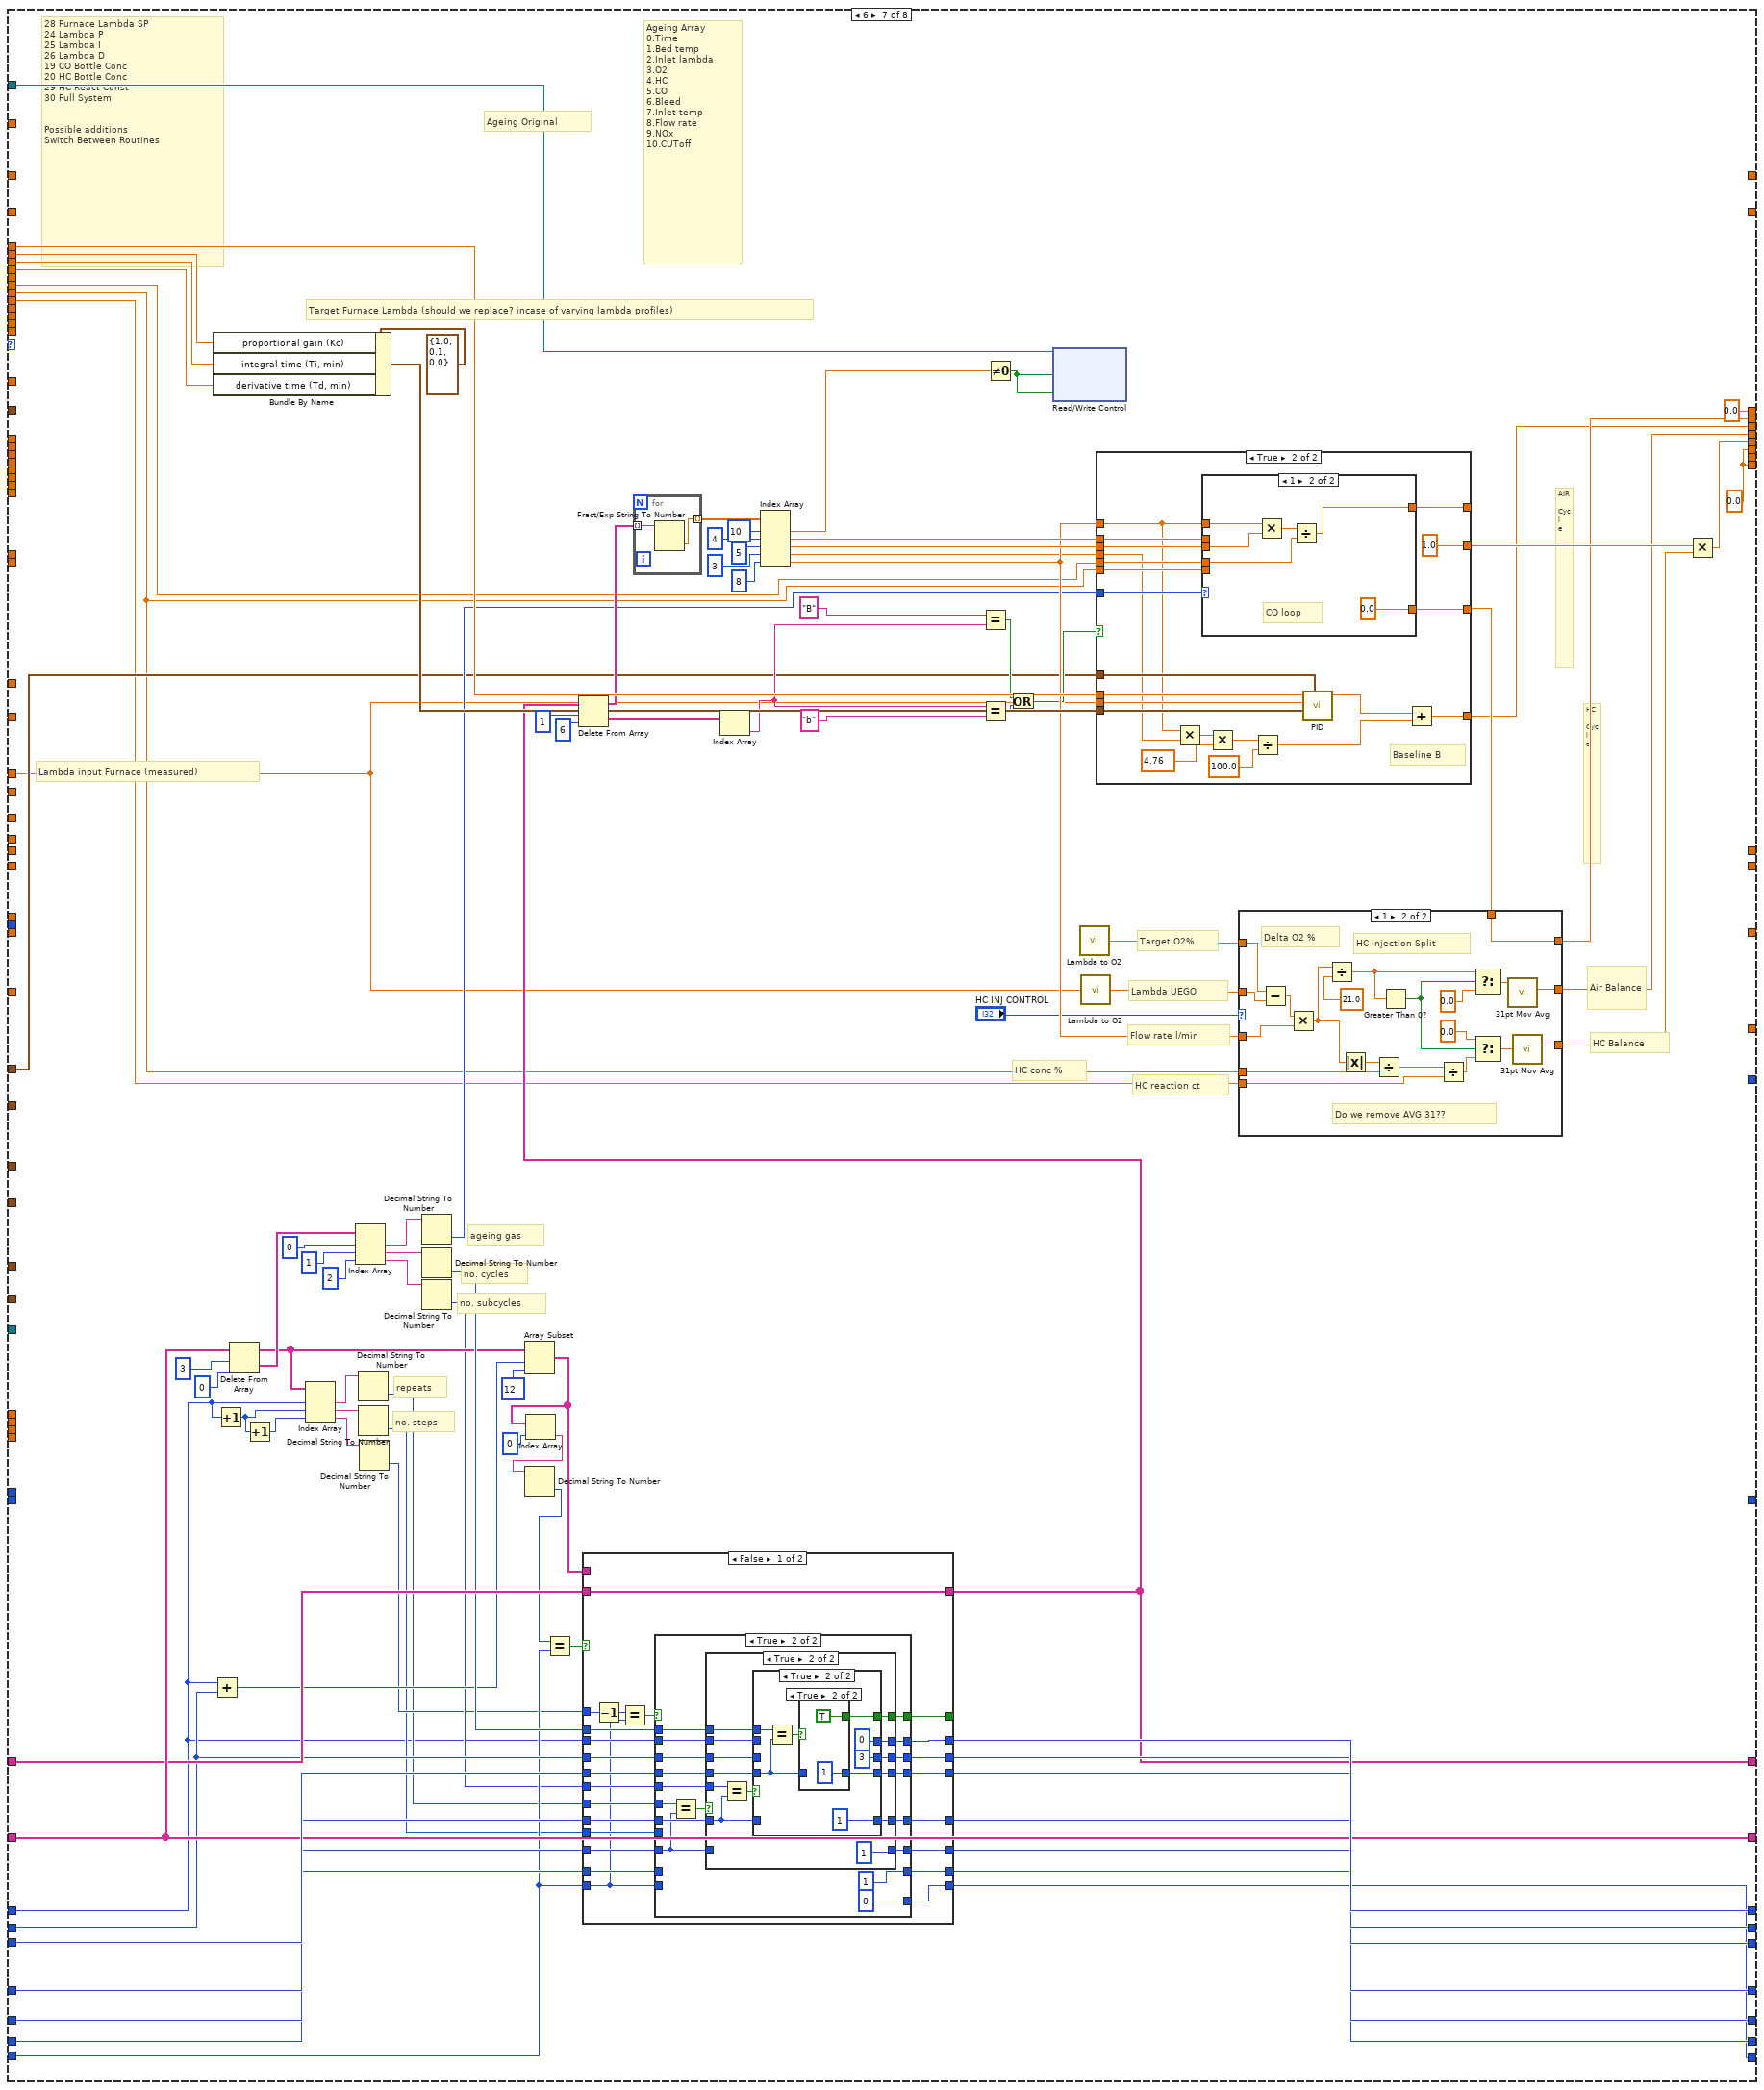
[diagram p17: hidden frame]
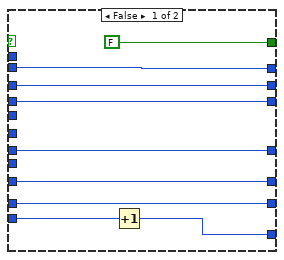
[diagram p18: hidden frame]
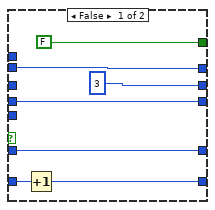
[diagram p19: hidden frame]
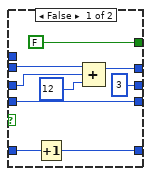
[diagram p20: hidden frame]
diagram:
  w5 = dbl[] [] ("Array Out Main")
  w24 = 0.0 ("Furnace Set-point")
  w7 = 0 ("It Out")
  w26 = string[] [] ("Ageing Variables")
  w8 = 0.0 ("Time to shut down 3")
  w9 = 0.0 ("output V")
  w20 = FALSE ("DIO On?")
  w50 = u16 0 ("length")
  # "1 DI no1 -errors\n1 DI no2 -states\n1 Flow rate 1 g/s\n1 Flow rate 2 g/s\n1 ECM AFR\n5 Mexa U\n5 Mexa D\n16 Temp I\n15 Temp II\n1 Furnace Temp 1\n1 Furnace Temp 2\n4 NOx\n4 EGO\n5 Mexa U 2\n5 MExa D 2"
  # "Control Variables Array\n\n0 Stop Cmd\n1 Test Number\n2 Flow Rate\n3 Start Temperature\n4 Stop Temperature\n5 Furnace Ramp Rate\n6 Inlet Lambda\n7 Inlet O2\n8 Inlet Lambda Rich\n9 Inlet Lambda Lean\n10 Inlet Temperature\n11 NO ppm SW\n12 NO ppm Loff\n13 NO:CO Ratio\n14 Temperature Limit\n15 Connected?  ****\n16 Inlet Temp Age\n17 Flow Rate Age\n\nAdv Settings\n\n18 NOx Conc\n19 CO Conc %\n20 HC Conc %\n21 Bleed H2O %\n22 Bleed CO2 %\n23 Bleed N2 %\n24 Lambda P\n25 Lambda I\n26 Lambda D\n27 Purge Duration\n28 Target Furnace Lambda\n29 HC Reaction ct\n30 Full System?\n\n31 Log Time\n32 Heat Load?\n33 Heat Load Constants"
  # "set safe values on critical outputs"
  # "Open one reference for each target"
  # "Set Shared Variable to safe values"
  # "Index2"
  # "Index1"
  # "Clock"
  # "Count.steps"
  # "Count.repeats"
  # "Count.subcycles"
  # "Count.cycles"
  # "Switch time"
  n1 = shared-variable "RT CompactRIO Target 2\\Library 1.lvlib\\Control Variables"(dbl[] [0.0, 0.0, 0.0, 0.0, 0.0, 0.0, 0.0, 0.0, 0.0, 0.0, 0.0, 0.0, 0.0, 0.0, 800.0] ("Control Variables")) -> ()  [unwired: 1 in, 1 out]
  n2 = xnode "Open FPGA VI Reference"("resource name"=tag "rio://192.168.0.2/RIO0") -> ("FPGA VI Reference Out"=w2:refnum<k20>, "error out"=w19:errorcluster)  [unwired: 1 in]
  n3 = xnode "Open FPGA VI Reference"("resource name"=tag "rio://169.254.0.7/RIO0") -> ("FPGA VI Reference Out"=w13:refnum<k20>, "error out"=w43:errorcluster)  [unwired: 1 in]
  n4 = xnode "Read/Write Control"("FPGA VI Reference In"=w13, "error in"=w43, "Command"=0, "Leak test on?"=w20, "DO On?"=w20, "CUToff 1"=w20, "CUToff 2"=w20) -> ("FPGA VI Reference Out"=w29:refnum<k20>, "error out"=w42:errorcluster)
  n5 = xnode "Read/Write Control"("FPGA VI Reference In"=w29) -> ("FPGA VI Reference Out"=w23:refnum<k20>, "error out"=w30:errorcluster)  [unwired: 8 in]
  n6 = node-c288("UEGO 1") -> (w12:T11)  [unwired: 3 in]
  n7 = node-c288("UEGO 2") -> (w18:T11)  [unwired: 3 in]
  n8 = node-c288("UEGO 3") -> (w4:T11)  [unwired: 3 in]
  n9 = node-c288() -> (w47:T11)  [unwired: 4 in]
  n10 = node-c288(i64 200 ("Period")) -> (w39:T11)  [unwired: 3 in]
  n11 = timed-loop {
    timing: w12 -> [_]
    timing-out: [_] -> w11
    tunnel: w2 -> [w63]
    stop <- w62 stop-if-true
    # "Sample Area 1 & 2"
    # "New Uego Sub Vi"
    n12 = node-c288() -> ()  [unwired: 1 in, 1 out]
    n13 = xnode "Read/Write Control"("FPGA VI Reference In"=w63) -> ("FPGA VI Reference Out"=w53:refnum<k20>, "UEGO-1_Data"=w54:T15)  [unwired: 1 in, 1 out]
    n14 = call <vilib>:"uego_rt_reve.vi"("UEGOModuleEnable"="UEGOModuleEnable", "UEGOCalibration"=T14 {"Stoich A/F Ratio"=14.7, "IpArray (mA)"=[-2.0, -1.9, -1.8, -1.7, -1.602, -1.5, -1.4, -1.3, -1.243, -1.1, -1.0, -0.927, -0.8, -0.7, -0.652, -0.5, -0.405, -0.183, -0.0746, -0.0398, -0.007, 0.0, 0.0146, 0.057, 0.097, 0.15, 0.193, 0.25, 0.329, 0.35, 0.4, 0.45, 0.509, 0.55, 0.6, 0.67, 0.7, 0.75, 0.8, 0.85, 0.9, 0.938, 1.0, 1.05, 1.1, 1.15, 1.2, 1.25, 1.3, 1.35, 1.4, 1.45, 1.5, 1.55, 1.6, 1.65, 1.7, 1.75, 1.8, 1.85, 1.9, 1.95, 2.0, 2.05, 2.1, 2.15, 2.2, 2.25, 2.3, 2.3565], "LambdaArray"=[0.65, 0.6607, 0.6732, 0.6866, 0.7, 0.714, 0.7278, 0.7418, 0.75, 0.7716, 0.7876, 0.7999, 0.8224, 0.841, 0.8502, 0.8802, 0.8999, 0.9501, 0.9791, 0.9895, 1.0, 1.0032, 1.01, 1.0301, 1.0498, 1.077, 1.1, 1.1319, 1.179, 1.1921, 1.2243, 1.2581, 1.3002, 1.331, 1.3703, 1.4289, 1.4554, 1.5016, 1.5504, 1.6021, 1.657, 1.701, 1.7774, 1.8437, 1.9145, 1.9904, 2.0719, 2.1597, 2.2545, 2.3571, 2.4687, 2.5904, 2.7236, 2.8701, 3.0321, 3.212, 3.4131, 3.6393, 3.8958, 4.189, 4.5275, 4.9229, 5.3907, 5.9531, 6.6421, 7.5061, 8.6219, 10.1187, 12.2328, 15.99]}, "UEGO Back Pressure (bar)"="UEGO Back Pressure (bar)", "UEGOData (From FPGA)"=w54, "SensorControl"="SensorControl") -> ("UEGO Diagnostics"=→"UEGO Diagnostics":T6, "UEGO Sensor Results"=→"UEGO Sensor Results":T2, "UEGO Heater (V)"=→"UEGO Heater (V)":T5, "UEGO Temperature (C)"=→"UEGO Temperature (C)":T7, "UEGOControl (To FPGA)"=w55:T16)  [unwired: 1 out]
    n15 = local read "STOP"() -> (w62:bool)
    n16 = xnode "Read/Write Control"("FPGA VI Reference In"=w53, "UEGO-1_Control"=w55) -> ()  [unwired: 1 in, 2 out]
    n17 = node-c288() -> ()  [unwired: 1 in, 1 out]
  }
  n18 = timed-loop {
    timing: w18 -> [_]
    timing-out: [_] -> w17
    tunnel: w2 -> [w76]
    stop <- w75 stop-if-true
    # "Pre-Furnace"
    # "Old Uego Sub Vi"
    n19 = node-c288() -> ()  [unwired: 1 in, 1 out]
    n20 = xnode "Read/Write Control"("FPGA VI Reference In"=w76) -> ("FPGA VI Reference Out"=w74:refnum<k20>, "UEGO-2_Data"=w69:T17)  [unwired: 1 in, 1 out]
    n21 = call <vilib>:"uego_rt_revd.vi"("UEGOModuleEnable"="UEGOModuleEnable 2", "UEGOCalibration"=T14 {"Stoich A/F Ratio"=14.7, "IpArray (mA)"=[-1.85, -1.08, -0.76, -0.47, 0.0, 0.34, 0.68, 0.95, 1.4, 2.55], "LambdaArray"=[0.7, 0.8, 0.85, 0.9, 1.009, 1.18, 1.43, 1.7, 2.42, 5.0]}, "UEGO Back Pressure (bar)"="UEGO Back Pressure (bar) 2", "UEGOData (From FPGA)"=w69, "SensorEnable"="SensorEnable 2") -> ("UEGO Diagnostics"=→"UEGO Diagnostics 2":T8, "UEGO Sensor Results"=→"UEGO Meas 2":T2, "UEGOControl (To FPGA)"=w68:T18)  [unwired: 3 out]
    n22 = local read "STOP"() -> (w75:bool)
    n23 = xnode "Read/Write Control"("FPGA VI Reference In"=w74, "UEGO-2_Control"=w68) -> ()  [unwired: 1 in, 2 out]
    n24 = node-c288() -> ()  [unwired: 1 in, 1 out]
  }
  n25 = timed-loop {
    timing: w4 -> [_]
    timing-out: [_] -> w3
    tunnel: w2 -> [w91]
    stop <- w90 stop-if-true
    # "Sample Area 3 & 4"
    # "NEW Uego Sub Vi"
    n26 = node-c288() -> ()  [unwired: 1 in, 1 out]
    n27 = xnode "Read/Write Control"("FPGA VI Reference In"=w91) -> ("FPGA VI Reference Out"=w81:refnum<k20>, "UEGO-3_Data"=w82:T15)  [unwired: 1 in, 1 out]
    n28 = call <vilib>:"uego_rt_reve.vi"("UEGOModuleEnable"="UEGOModuleEnable 3", "UEGOCalibration"=T14 {"Stoich A/F Ratio"=14.7, "IpArray (mA)"=[-2.0, -1.9, -1.8, -1.7, -1.602, -1.5, -1.4, -1.3, -1.243, -1.1, -1.0, -0.927, -0.8, -0.7, -0.652, -0.5, -0.405, -0.183, -0.0746, -0.0398, -0.007, 0.0, 0.0146, 0.057, 0.097, 0.15, 0.193, 0.25, 0.329, 0.35, 0.4, 0.45, 0.509, 0.55, 0.6, 0.67, 0.7, 0.75, 0.8, 0.85, 0.9, 0.938, 1.0, 1.05, 1.1, 1.15, 1.2, 1.25, 1.3, 1.35, 1.4, 1.45, 1.5, 1.55, 1.6, 1.65, 1.7, 1.75, 1.8, 1.85, 1.9, 1.95, 2.0, 2.05, 2.1, 2.15, 2.2, 2.25, 2.3, 2.3565], "LambdaArray"=[0.65, 0.6607, 0.6732, 0.6866, 0.7, 0.714, 0.7278, 0.7418, 0.75, 0.7716, 0.7876, 0.7999, 0.8224, 0.841, 0.8502, 0.8802, 0.8999, 0.9501, 0.9791, 0.9895, 1.0, 1.0032, 1.01, 1.0301, 1.0498, 1.077, 1.1, 1.1319, 1.179, 1.1921, 1.2243, 1.2581, 1.3002, 1.331, 1.3703, 1.4289, 1.4554, 1.5016, 1.5504, 1.6021, 1.657, 1.701, 1.7774, 1.8437, 1.9145, 1.9904, 2.0719, 2.1597, 2.2545, 2.3571, 2.4687, 2.5904, 2.7236, 2.8701, 3.0321, 3.212, 3.4131, 3.6393, 3.8958, 4.189, 4.5275, 4.9229, 5.3907, 5.9531, 6.6421, 7.5061, 8.6219, 10.1187, 12.2328, 15.99]}, "UEGO Back Pressure (bar)"="UEGO Back Pressure (bar) 3", "UEGOData (From FPGA)"=w82, "SensorControl"="SensorControl 2") -> ("UEGO Diagnostics"=→"UEGO Diagnostics 3":T6, "UEGO Sensor Results"=→"UEGO Sensor Results 2":T2, "UEGO Heater (V)"=→"UEGO Heater (V) 2":T5, "UEGO Temperature (C)"=→"UEGO Temperature (C) 2":T7, "UEGOControl (To FPGA)"=w83:T16)  [unwired: 1 out]
    n29 = local read "STOP"() -> (w90:bool)
    n30 = xnode "Read/Write Control"("FPGA VI Reference In"=w81, "UEGO-3_Control"=w83) -> ()  [unwired: 1 in, 2 out]
    n31 = node-c288() -> ()  [unwired: 1 in, 1 out]
  }
  n32 = timed-loop {
    shift-right: [w340] -> _
    shift-left: u16 0 ("UInt16") -> [w364]
    tunnel: w29 -> [w182]
    shift-right: [w339] -> _
    shift-left: w50 -> [w337]
    shift-right: [w338] -> _
    shift-left: w50 -> [w336]
    timing: w47 -> [_]
    timing-out: [_] -> w46
    shift-right: [w326] -> _
    shift-left: FALSE ("Alarm?") -> [w325]
    tunnel: w2 -> [w231]
    tunnel: w42 -> [w277]
    shift-right: [w299] -> _
    shift-left: w9 -> [w298]
    shift-right: [w297] -> _
    shift-left: w9 -> [w296]
    shift-right: [w175] -> _
    shift-left: w8 -> [w179]
    shift-right: [w174] -> _
    shift-left: FALSE -> [w178]
    shift-right: [w273] -> _
    shift-left: _ -> [w272]
    shift-right: [w264] -> _
    shift-left: w7 -> [w260]
    shift-right: [w263] -> _
    shift-left: w7 -> [w259]
    shift-right: [w261] -> _
    shift-left: w24 -> [w257]
    shift-right: [w262] -> _
    shift-left: w24 -> [w258]
    shift-right: [w251] -> _
    shift-left: _ -> [w250]
    shift-right: [w110] -> _
    shift-left: _ -> [w249]
    tunnel: [w242] -> w22
    tunnel: [w241] -> w21
    shift-right: [w204] -> _
    shift-left: 0.0 ("y") -> [w203]
    shift-right: [w194] -> _
    shift-left: w7 -> [w195]
    shift-right: [w105] -> _
    shift-left: _ -> [w139]
    shift-right: [w185] -> _
    shift-left: w9 -> [w186]
    shift-right: [w172] -> _
    shift-left: w8 -> [w173]
    shift-right: [w165] -> _
    shift-left: _ -> [w167]
    shift-right: [w164] -> _
    shift-left: _ -> [w166]
    shift-right: [w162] -> _
    shift-left: _ -> [w163]
    shift-right: [w146] -> _
    shift-left: w5 -> [w148]
    shift-right: [w145] -> _
    shift-left: w5 -> [w147]
    shift-right: [w125] -> _
    shift-left: _ -> [w133]
    shift-right: [w124] -> _
    shift-left: _ -> [w132]
    shift-right: [w104] -> _
    shift-left: _ -> [w129]
    shift-right: [w99] -> _
    shift-left: _ -> [w128]
    stop <- "STOP" stop-if-true
    w315 = sgl 80.0 ("y")
    w320 = 4 ("length")
    # "Cycle Length"
    # "Analyser Data"
    # "Rapidox"
    # "584 U"
    # "584 D"
    # "1Hz MFC's\n\n0. CO2\n1. N2\n2. SO2\n3. H2O\n4. N2P"
    # "Fur 2"
    # "l/min\ng/s"
    # "T Bed\nT Inlet\nT Bed\nT Inlet"
    # "30"
    # "25"
    # "20"
    # "10"
    # "5"
    # "30"
    # "25"
    # "20"
    # "15"
    # "10"
    # "5"
    # "0"
    # "Pressure calib"
    # "g/s 2"
    # "calibration eq"
    # "Furnace 2"
    # "Furnace 1"
    # "Connect to Multigas?"
    # "tank P"
    # "Rapidox O2 %"
    # "CONTROL LOOP"
    # "TC I"
    n33 = node-c288() -> (→"Iteration Duration 2":i64)  [unwired: 1 in]
    n34 = local read "Control Variables"() -> (w278:dbl[])
    n35 = xnode "Read/Write Control"("FPGA VI Reference In"=w182, "error in"=w277) -> ("Array 1 In"=w284:fxp<+/-,35,9>[])  [unwired: 2 out]
    n36 = xnode "Read/Write Control"("FPGA VI Reference In"=w231) -> ("TC array"=w303:fxp<+/-,24,-2>[])  [unwired: 1 in, 2 out]
    n37 = xnode "Read/Write Control"("FPGA VI Reference In"=w231) -> ("NOxSensorData 1"=w237:T19, "NOxSensorData 2"=w238:T19)  [unwired: 1 in, 2 out]
    n38 = xnode "Read/Write Control"("FPGA VI Reference In"=w231) -> ("Expansion Input Array"=w213:fxp<+/-,34,9>[])  [unwired: 1 in, 2 out]
    n39 = local read "Cycle Length"() -> (w134:i32)
    n40 = Delete From Array(array=w303, length=17, index=0 ("length")) -> (deleted portion=w300:fxp<+/-,24,-2>[])  [unwired: 1 out]
    n41 = Index Array(array=w284, index=0 ("length")) -> (element=w142:fxp<+/-,35,9>)
    n42 = Delete From Array(array=w284, length=18 ("index"), index=3 ("length")) -> (deleted portion=w365:fxp<+/-,35,9>[])  [unwired: 1 out]
    n43 = Delete From Array(array=w284, length=w320, index=21) -> (deleted portion=w362:fxp<+/-,35,9>[])  [unwired: 1 out]
    n44 = Delete From Array(array=w284, length=w320, index=25) -> (deleted portion=w322:fxp<+/-,35,9>[])  [unwired: 1 out]
    n45 = Index Array(array=w278) -> (element #1=w358:dbl, element #2=w354:dbl, element #3=w353:dbl, element #4=w352:dbl, element #5=w310:dbl, element #6=w351:dbl, element #7=w349:dbl, element #8=w348:dbl, element #9=w347:dbl, element #10=w346:dbl, element #11=w345:dbl, element #12=w344:dbl, element #13=w343:dbl, element #14=w342:dbl, element #15=w341:dbl, element #16=w294:dbl, element #17=w293:dbl, element #18=w292:dbl, element #19=w291:dbl, element #20=w290:dbl, element #21=w289:dbl, element #22=w288:dbl, element #23=w287:dbl, element #24=w286:dbl, element #25=w281:dbl, element #26=w280:dbl, element #27=w279:dbl, element #28=w285:dbl, element #29=w306:dbl, element #30=w305:dbl, element #31=w307:dbl, element #32=w254:dbl, element #33=w253:dbl, element #34=w247:dbl, element #35=w246:dbl, element #36=w245:dbl, element #37=w201:dbl, element #38=w188:dbl)  [unwired: 38 in]
    n46 = call "TC calibrate.vi"("TC in"=w300) -> ("TC out"=w271:sgl[])  [unwired: 10 in]
    n47 = xnode "Read/Write Control"("FPGA VI Reference In"=w182, "Emission SV"=w178) -> ()  [unwired: 1 in, 2 out]
    n48 = call "31pt Mov Avg.vi"("Value in"=w142) -> ("Value out"=w255:dbl)  [unwired: 10 in]
    n49 = call "TC calibrate.vi"("TC in"=w365) -> ("TC out"=w136:sgl[])  [unwired: 10 in]
    n50 = call "Array to temp.vi"("Array"=w362) -> ("Temperature"=w266:sgl)  [unwired: 10 in]
    n51 = call "Array to temp.vi"("Array"=w322) -> ("Temperature"=w265:sgl)  [unwired: 10 in]
    n52 = call "NOx MAX.vi"("NOx Input 2"=w238, "NOx Input 1"=w237) -> ("Output Array"=w235:dbl[])  [unwired: 3 in, 6 out]
    n53 = Divide(x=w134, y=5.0) -> (x/y=w170:dbl)
    n54 = Build Array(w247, w246, w245, w201, w188) -> (w130:dbl[])
    n55 = Not Equal To 0?(x=w294) -> (x != 0?=w268:bool)
    n56 = expression code="0.02*x+3"("TankHi") -> (w329:dbl)
    n57 = expression code="0.02*x+3"("TankLo") -> (w330:dbl)
    n58 = Index Array(array=w271, index #1=4 ("index"), index #2=5 ("index"), index #3=7 ("index"), index #4=8 ("index")) -> (element #1=w159:sgl, element #2=w154:sgl, element #3=w319:sgl, element #4=w314:sgl)
    n59 = Index Array(array=w130, index=3) -> (element=w197:dbl)
    n60 = Index Array(array=w130, index=4) -> (element=w192:dbl)
    n61 = local read "UEGO Meas 2"() -> (w210:T2)
    n62 = local read "UEGO Array"() -> (w141:dbl[])
    n63 = Not(x=w178) -> (.not. x?=w267:bool)
    n64 = Decrement(x=w197) -> (x-1=w196:dbl)
    n65 = Decrement(x=w192) -> (x-1=w193:dbl)
    n66 = Build Array (concatenate)(w271, w266, w265) -> (w217:sgl[])
    n67 = Greater?(x=w319, y=w315) -> (0:w312:bool)
    n68 = Greater?(x=w314, y=w315) -> (0:w311:bool)
    n69 = Index Array(array=w136) -> (element=w131:sgl)  [unwired: 1 in]
    n70 = Index Array(array=w136) -> (element=w135:sgl)  [unwired: 1 in]
    n71 = expression code="50*x-150"(w255) -> (w143:dbl)
    "Tank Pressure" <- w143
    "Pressure" <- w143
    n72 = And(x=w268, y=w178) -> (x .and. y?=w270:bool)
    n73 = And(x=w268, y=w267) -> (x .and. y?=w269:bool)
    n74 = Index Array(array=w136, index #1=2 ("index"), index #2=3 ("index"), index #3=1 ("index")) -> (element #1=w168:sgl, element #2=w183:sgl, element #3=w184:sgl)
    "Inlet Temp" <- w184
    n75 = Index Array(array=w136, index=w196) -> (element=w152:sgl)
    n76 = Index Array(array=w136, index=w193) -> (element=w151:sgl)
    n77 = xnode "Read/Write Control"("FPGA VI Reference In"=w182, "error in"=w277, "TankHi"=w329, "TankLo"=w330, "ISO4_SV"=w270, "ISO5_SV"=w269) -> ("FPGA VI Reference Out"=w355:refnum<k20>, "DI no 1"=w144:u16, "DI no 2"=w275:u8)  [unwired: 1 out]
    "DI no1" <- w144
    n78 = Unbundle By Name(w210) -> ("UEGO1Lambda"=w94:sgl, "UEGO2Lambda"=w140:sgl)
    n79 = local read "Flow 1"() -> (w160:dbl)
    n80 = call "Mov_Avg_JS_Dual.vi"("Cycle Length"=w134, "Array In 2"=w132, "Input 2"=w131, "Array In"=w133, "Input"=w135) -> ("Array Out Main 2"=w124:dbl[], "Mean 2"=w126:dbl, "Array Out Main"=w125:dbl[], "Mean"=w127:dbl)  [unwired: 3 in]
    n81 = Boolean To (0,1)(Boolean=w178) -> (0, 1=w209:i16)
    n82 = call "Mov_Avg_JS_Dual.vi"("Cycle Length"=w134, "Array In 2"=w147, "Input 2"=w151, "Array In"=w148, "Input"=w152) -> ("Array Out Main 2"=w145:dbl[], "Mean 2"=w149:dbl, "Array Out Main"=w146:dbl[], "Mean"=w150:dbl)  [unwired: 3 in]
    n83 = Or(x=w312, y=w311) -> (x .or. y?=w313:bool)
    n84 = Equal?(x=w184, y=sgl 1372.0) -> (x = y?=w282:bool)
    n85 = Greater?(x=w184, y=w341) -> (0:w283:bool)
    n86 = Delete From Array(array=w213, length=54 ("index"), index=2 ("length")) -> (deleted portion=w224:fxp<+/-,34,9>[])  [unwired: 1 out]
    n87 = Delete From Array(array=w213, length=28 ("index"), index=56 ("length")) -> (deleted portion=w225:fxp<+/-,34,9>[])  [unwired: 1 out]
    n88 = Delete From Array(array=w213, length=28 ("index"), index=84 ("length")) -> (deleted portion=w223:fxp<+/-,34,9>[])  [unwired: 1 out]
    n89 = Not Equal To 0?(x=w358) -> (x != 0?=w334:bool)
    n90 = local read "Flow 2"() -> (w155:dbl)
    n91 = call "Heat_Load_Calc_Red.vi"("Input Array 2"=w249, "Input Array"=w130, "Avg Temp In"=w150, "Temp In"=w152) -> ("Output Array"=w137:dbl[])  [unwired: 4 in, 3 out]
    n92 = call "Heat_Load_Calc_Red.vi"("Input Array 2"=w139, "Input Array"=w130, "Avg Temp In"=w149, "Temp In"=w151) -> ("Output Array"=w138:dbl[])  [unwired: 4 in, 3 out]
    n93 = call "Heat_Load_Calc_Red.vi"("Input Array 2"=w129, "Input Array"=w130, "Avg Temp In"=w127, "Temp In"=w135) -> ("Output Array"=w123:dbl[])  [unwired: 4 in, 3 out]
    n94 = call "Heat_Load_Calc_Red.vi"("Input Array 2"=w128, "Input Array"=w130, "Avg Temp In"=w126, "Temp In"=w131) -> ("Output Array"=w121:dbl[])  [unwired: 4 in, 3 out]
    n95 = Not Equal To 0?(x=w307) -> (x != 0?=w309:bool)
    n96 = Index Array(array=w136, index #1=0 ("index")) -> (element #1=w169:sgl)  [unwired: 1 in, 1 out]
    n97 = call "Error handler.vi"("Test Alarms"=w272, "DI no 1 in"=w144, "Error 4"=w334, "Error 3"=w283, "Error 2"=w282, "Error 1"=w313) -> ("Alarm?"=w326:bool, "Loop out"=w333:u16, "Error no out"=w276:dbl)  [unwired: 3 in]
    n98 = call "Rapidox parse.vi"("RapidoxOutput"=w224) -> ("O2 %"=w230:dbl)  [unwired: 10 in]
    n99 = call "Mexa parse.vi"("Byte array"=w225) -> ("Output"=w221:dbl[])  [unwired: 10 in]
    n100 = call "Mexa parse.vi"("Byte array"=w223) -> ("Output"=w220:dbl[])  [unwired: 10 in]
    n101 = Equal?(x="Sw time", y=w179) -> (x = y?=w180:bool)
    n102 = Not Equal To 0?(x=w253) -> (x != 0?=w252:bool)
    n103 = Greater?(x=w326, y=w325) -> (0:w324:bool)
    n104 = call "Flow_Selection.vi"("Linearized Temperature"=w154, "Flow"=w155, "Pressure Transducer 2"="Pressure Transducer 2") -> ("Flow rate g/s"=w156:dbl)  [unwired: 7 in, 1 out]
    n105 = call "3pt Mov Avg.vi"("Value in"=w230) -> ("Value out"=w219:dbl)  [unwired: 10 in]
    "Rapidox" <- w219
    n106 = Build Array (concatenate)(w141, w143, w136, w217) -> (w216:dbl[])
    n107 = case shown="False" w180 {
      tunnel: [w379 w381] -> w176
      tunnel: w178 -> [w379 w382]
      tunnel: [w378 0.0] -> w177
      tunnel: w179 -> [w377 _]
      frame False {
        n108 = Increment(x=w377) -> (x+1=w378:dbl)
      }
      frame True {
        n109 = Not(x=w382) -> (.not. x?=w381:bool)
      }
    }
    n110 = Build Array (concatenate)(w209, w94, w140, w235) -> (w211:dbl[])
    n111 = call "Flow_Selection.vi"("Linearized Temperature"=w159, "Flow"=w160, "Pressure Transducer 2"="Pressure Transducer 1") -> ("Flow rate g/s"=w157:dbl, "Flow rate l/min"=w158:dbl)  [unwired: 7 in]
    n112 = Build Array (concatenate)(w219, w221, w220) -> (w215:dbl[])
    n113 = Build Array(w276, w275, w157, w156) -> (w274:dbl[])
    n114 = Select(t=w333, s=w324, f=w364) -> (s? t:f=w206:i32)
    "Loop No." <- w206
    n115 = Build Array (concatenate)(w274, w216, w215, w211) -> (w218:dbl[])
    n116 = case shown="True" "Reset Heat Load" {
      tunnel: [w388 dbl[] [] ("Output Array")] -> w110
      tunnel: w137 -> [w388 _]
      tunnel: "Reset Heat Load" -> [w387 _]
      tunnel: [w387 FALSE ("Reset Heat Load")] -> w198
      frame False {
      }
      frame True {
      }
    }
    n117 = case shown="False" "Reset Heat Load 2" {
      tunnel: [w384 dbl[] [] ("Output Array")] -> w105
      tunnel: w138 -> [w384 _]
      tunnel: "Reset Heat Load 2" -> [w383 _]
      tunnel: [w383 FALSE ("Reset Heat Load")] -> w190
      frame False {
      }
      frame True {
      }
    }
    n118 = case shown="False" "Reset Heat Load 3" {
      tunnel: [w370 dbl[] [] ("Output Array")] -> w104
      tunnel: w123 -> [w370 _]
      tunnel: "Reset Heat Load 3" -> [w369 _]
      tunnel: [w369 FALSE ("Reset Heat Load")] -> w119
      frame False {
      }
      frame True {
      }
    }
    n119 = case shown="True" "Reset Heat Load 4" {
      tunnel: [w374 dbl[] [] ("Output Array")] -> w99
      tunnel: w121 -> [w374 _]
      tunnel: "Reset Heat Load 4" -> [w373 _]
      tunnel: [w373 FALSE ("Reset Heat Load")] -> w118
      frame False {
      }
      frame True {
      }
    }
    n120 = local write "Reset Heat Load"(w198) -> ()
    n121 = local write "Reset Heat Load 2"(w190) -> ()
    n122 = local write "Reset Heat Load 3"(w119) -> ()
    n123 = local write "Reset Heat Load 4"(w118) -> ()
    n124 = call "Heat_Load_Control.vi"("Heat Load Control"="Heat Load Control", "Catalyst 4"=w99, "Catalyst 3"=w104, "Catalyst 2"=w105, "Catalyst 1"=w110) -> ("Ki() Array"=w115:dbl[], "Control Cat"=w116:dbl)  [unwired: 5 in]
    n125 = case shown="3" w206 {
      tunnel: w355 -> [w405 w424 w502 w647 _ w1434]
      tunnel: [w407 2 w506 w665 w1417 u16 0 ("length")] -> w340
      tunnel: [w396 w411 w484 w613 w1416 w1420] -> w240
      tunnel: w157 -> [_ _ w441 w667 w1411 _]
      tunnel: w352 -> [_ _ w496 _ _ _]
      tunnel: w353 -> [_ _ _ w669 _ _]
      tunnel: w348 -> [_ _ _ w668 _ _]
      tunnel: w349 -> [_ _ _ w666 _ _]
      tunnel: w351 -> [_ w423 _ _ _ _]
      tunnel: w310 -> [_ _ _ w664 _ _]
      tunnel: w354 -> [_ _ w492 w663 _ _]
      tunnel: w143 -> [_ _ _ w662 _ _]
      tunnel: w347 -> [_ _ _ w655 _ _]
      tunnel: w346 -> [_ _ _ w656 _ _]
      tunnel: w345 -> [_ _ w497 w659 _ _]
      tunnel: w337 -> [_ _ _ w661 _ _]
      tunnel: [w408 w427 w505 w660 w1415 w1433] -> w339
      tunnel: w336 -> [_ _ _ w658 _ _]
      tunnel: [w408 w427 w505 w657 w1415 w1433] -> w338
      tunnel: "PID Inverter" -> [_ _ w468 w654 w1414 _]
      tunnel: "PID Furnace 2" -> [_ _ w459 w653 _ _]
      tunnel: w344 -> [_ _ _ w652 _ _]
      tunnel: w343 -> [_ _ _ w651 _ _]
      tunnel: w342 -> [_ _ _ w650 _ _]
      tunnel: w291 -> [_ _ _ w649 _ _]
      tunnel: [w404 1 2 3 4 5] -> w350
      tunnel: w158 -> [_ _ _ w646 _ _]
      tunnel: w290 -> [_ _ _ w645 _ _]
      tunnel: w289 -> [_ _ _ w630 _ _]
      tunnel: w286 -> [_ _ _ w644 _ _]
      tunnel: w287 -> [_ _ _ w643 _ _]
      tunnel: [w404 0 0 w642 0 0] -> w328
      tunnel: w292 -> [_ _ _ _ _ _]
      tunnel: w293 -> [_ _ w498 _ _ _]
      tunnel: "NO PID Sweep Test" -> [_ _ _ w641 _ _]
      tunnel: w285 -> [_ _ w431 _ _ _]
      tunnel: w288 -> [_ _ _ w638 _ _]
      tunnel: w309 -> [_ _ w474 w640 _ _]
      tunnel: w168 -> [_ _ _ w603 _ _]
      tunnel: w156 -> [_ _ w467 w639 _ _]
      tunnel: w306 -> [_ _ _ w637 _ _]
      tunnel: w305 -> [_ _ _ w636 _ _]
      tunnel: [_ _ _ w635 _ _] -> w299
      tunnel: w298 -> [_ _ _ w634 _ _]
      tunnel: [_ _ _ w633 _ _] -> w297
      tunnel: w296 -> [_ _ _ w632 _ _]
      tunnel: "Fan Speed V" -> [_ _ w462 w631 w1405 _]
      tunnel: w281 -> [_ _ _ _ _ _]
      tunnel: w280 -> [_ _ _ _ _ _]
      tunnel: w279 -> [_ _ _ _ _ _]
      tunnel: [w403 w418 w491 w629 w1404 _] -> w273
      tunnel: w272 -> [w403 w418 w491 w628 w1404 _]
      tunnel: w266 -> [_ _ w470 w627 _ _]
      tunnel: w265 -> [_ _ w469 w626 _ _]
      tunnel: [_ _ _ w625 _ _] -> w264
      tunnel: [_ _ _ w624 _ _] -> w263
      tunnel: [_ _ _ w623 _ _] -> w262
      tunnel: [_ _ _ w622 _ _] -> w261
      tunnel: w260 -> [_ _ _ w621 _ _]
      tunnel: w259 -> [_ _ _ w620 _ _]
      tunnel: w258 -> [_ _ _ w619 _ _]
      tunnel: w257 -> [_ _ _ w618 _ _]
      tunnel: "PID Furnace 1" -> [_ _ _ w617 _ _]
      tunnel: w254 -> [_ _ w490 _ _ _]
      tunnel: w252 -> [_ _ _ w616 _ _]
      tunnel: [0.0 ("Numeric") 0.0 ("Numeric") w490 w614 0.0 ("Numeric") 0.0 ("Numeric")] -> w251
      tunnel: w250 -> [_ _ _ w615 _ _]
      tunnel: w245 -> [_ _ _ w611 _ _]
      tunnel: "Furnace Manual Mode" -> [_ _ _ w610 _ _]
      tunnel: [u8[] [64, 160, 0, 0, 133, 108, 64, 160, 0, 0, 133, 108] ("SP&CRC") u8[] [64, 160, 0, 0, 133, 108, 64, 160, 0, 0, 133, 108] ("SP&CRC") w481 w609 w1399 u8[] [64, 160, 0, 0, 133, 108, 64, 160, 0, 0, 133, 108] ("SP&CRC")] -> w243
      tunnel: [bool[] [FALSE, FALSE, FALSE, FALSE, FALSE] ("SV Array") bool[] [FALSE, FALSE, FALSE, FALSE, FALSE] ("SV Array") w480 w606 w1397 bool[] [FALSE, FALSE, FALSE, FALSE, FALSE] ("SV Array")] -> w239
      tunnel: "Furnace 1" -> [_ _ _ w605 _ _]
      tunnel: "Fan PID" -> [_ _ w461 w604 _ _]
      tunnel: "Furnace 2" -> [_ _ _ w602 _ _]
      tunnel: w219 -> [_ _ w476 w601 _ _]
      tunnel: "Set-point Fan" -> [_ _ w454 w600 _ _]
      tunnel: 400 ("y") -> [_ _ _ w599 _ _]
      tunnel: 10.0 ("y") -> [_ _ _ w598 _ _]
      tunnel: w94 -> [_ _ _ w597 _ _]
      tunnel: 300 ("y") -> [_ _ _ w596 _ _]
      tunnel: [_ _ _ w595 _ _] -> w204
      tunnel: w203 -> [_ _ _ w594 _ _]
      tunnel: [_ _ _ w593 _ _] -> w202
      tunnel: w195 -> [_ _ w448 _ _ _]
      tunnel: w184 -> [_ _ w446 _ _ _]
      tunnel: [_ _ w447 0 ("index") _ _] -> w194
      tunnel: [_ _ w437 w591 _ _] -> _
      tunnel: "V Max Flow" -> [_ _ w436 w590 _ _]
      tunnel: w186 -> [_ _ _ w589 _ _]
      tunnel: [_ _ w435 _ _ _] -> w185
      tunnel: w183 -> [_ _ w434 _ _ _]
      tunnel: w177 -> [_ _ w433 w588 _ _]
      tunnel: w176 -> [_ _ w432 w587 _ _]
      tunnel: [w394 w409 w433 w588 0.0 ("Sw time") w1418] -> w175
      tunnel: [FALSE FALSE w432 w587 FALSE FALSE] -> w174
      tunnel: w173 -> [_ _ _ w586 w1392 _]
      tunnel: [w394 w409 w431 w586 w1391 w1418] -> w172
      tunnel: w170 -> [_ _ _ w585 _ _]
      tunnel: w167 -> [_ _ _ w584 _ _]
      tunnel: w166 -> [_ _ _ w583 _ _]
      tunnel: w169 -> [_ _ _ w582 _ _]
      tunnel: w168 -> [_ _ _ w581 _ _]
      tunnel: [_ _ _ w580 _ _] -> w165
      tunnel: [_ _ _ w579 _ _] -> w164
      tunnel: w163 -> [_ _ _ w578 _ _]
      tunnel: [_ _ _ w577 _ _] -> w162
      tunnel: w116 -> [_ _ _ w576 _ _]
      tunnel: w94 -> [_ _ w428 _ _ _]
      frame 0, Default {
        (unwired) dbl[] [0.0, 0.0, 65.0, 48.0, 48.0, 48.0, 48.0, 48.0, 13.0, 68.0, 48.0, 48.0, 48.0, 48.0, 48.0, 13.0, 69.0, 48.0, 48.0, 48.0, 48.0, 48.0, 13.0, 70.0, 48.0, 48.0, 48.0, 48.0, 48.0, 13.0, 71.0, 48.0, 48.0, 48.0, 48.0, 48.0, 13.0] ("appended array")
        w394 = 0.0 ("Sw time")
        (unwired) 0.0 ("dt (s)")
        (unwired) 0.0 ("f")
        w404 = 0
        w408 = u16 0 ("length")
        # "Standby"
        # "an array of 37 values"
        # "safety values are sent to the system"
        n126 = xnode "Read/Write Control"("FPGA VI Reference In"=w405, "Command"=0) -> ()  [unwired: 1 in, 2 out]
        n127 = shared-variable "RT CompactRIO Target 2\\Library 1.lvlib\\Enum 1"() -> (w407:u16)  [unwired: 1 in, 1 out]
        n128 = call "MFR Flow to SP 2-3.vi"("MFC SPs"=dbl[] [0.0, 0.0, 0.0, 0.0, 0.0]) -> ("MFC array"=w399:dbl[])  [unwired: 9 in, 1 out]
        n129 = Build Array (concatenate)(dbl[] [0.0, 0.0] ("element"), w399) -> (w396:dbl[])
      }
      frame 1 {
        (unwired) dbl[] [0.0, 0.0, 65.0, 48.0, 48.0, 48.0, 48.0, 48.0, 13.0, 68.0, 48.0, 48.0, 48.0, 48.0, 48.0, 13.0, 69.0, 48.0, 48.0, 48.0, 48.0, 48.0, 13.0, 70.0, 48.0, 48.0, 48.0, 48.0, 48.0, 13.0, 71.0, 48.0, 48.0, 48.0, 48.0, 48.0, 13.0] ("appended array")
        w409 = 0.0 ("Sw time")
        (unwired) 0.0 ("dt (s)")
        (unwired) 0.0 ("f")
        w427 = u16 0
        # "Initialise"
        n130 = call "Furnace rate SP calc.vi"("SP"=w423) -> ("SP&CRC"=w419:u8[])  [unwired: 10 in]
        n131 = xnode "Read/Write Control"("FPGA VI Reference In"=w424, "Ramp rate 1 SP&CRC"=w419, "Ramp rate 2 SP&CRC"=w419, "Command"=i16 1, "DO On?"=TRUE) -> ()  [unwired: 1 in, 2 out]
        n132 = call "MFR Flow to SP 2-3.vi"("MFC SPs"=dbl[] [0.0, 0.0, 0.0, 0.0, 0.0]) -> ("MFC array"=w414:dbl[])  [unwired: 9 in, 1 out]
        n133 = Build Array (concatenate)(dbl[] [0.0, 0.0] ("element"), w414) -> (w411:dbl[])
      }
      frame 2 {
        (unwired) u16 0 ("UInt16")
        w473 = FALSE ("CUToff 1")
        (unwired) 0.0 ("dt (s)")
        w505 = u16 0
        # "0. CO\n1. HC\n2. Air\n3. NO\n4. CO2\n5. N2\n6. SO2\n7. H2O\n8. AirB"
        # "Buildup"
        # "O2% threshold limit"
        n134 = Equal To 0?(x=w448) -> (x = 0?=w460:bool)
        n135 = xnode "Read/Write Control"("FPGA VI Reference In"=w502, "Command"=0, "CUToff 1"=w473, "CUToff 2"=w473, "DO On?"=TRUE) -> ()  [unwired: 1 in, 2 out]
        n136 = case shown="4" w492 {
          tunnel: w496 -> [_ _ _ _ _]
          tunnel: w497 -> [_ _ _ _ _]
          tunnel: ["CO Furnace Inlet" "HC Furnace Inlet" "NO Furnace Inlet" "SW Furnace Inlet" "Age Furnace Inlet"] -> w452
          tunnel: w498 -> [_ _ _ _ _]
          tunnel: ["CO Rap Lim" "HC rap lim" "NO Rap Lim" "SW rap lim" "Age Rap Lim"] -> w477
          frame 0, Default {
          }
          frame 1 {
          }
          frame 2 {
          }
          frame 3 {
          }
          frame 4 {
          }
        }
        n137 = case shown="True" w460 {
          tunnel: [w527 "Furnace 1"] -> w472
          tunnel: [w525 "Furnace 2"] -> w471
          tunnel: w470 -> [_ w531]
          tunnel: w469 -> [_ w530]
          tunnel: [TRUE w529] -> w445
          tunnel: w446 -> [w526 _]
          tunnel: w434 -> [w524 _]
          tunnel: w459 -> [w523 _]
          tunnel: w452 -> [w522 _]
          tunnel: w452 -> [w515 _]
          tunnel: w446 -> [w516 _]
          tunnel: [w514 FALSE] -> w442
          tunnel: [w511 _] -> w438
          frame False {
            # "Furnace PID Based on Tin"
            n138 = Subtract(x=w516, y=sgl 10.0) -> (x-y=w518:sgl)
            n139 = Add(x=sgl 10.0, y=w516) -> (x+y=w517:sgl)
            n140 = call "Furnace PID SP 1.vi"("PID gains"=w523, "PV deg C"=w526, "User SP Deg C"=w522) -> ("output T SP"=w527:dbl, "Test Probe"=w512:dbl[])  [unwired: 7 in]
            n141 = call "Furnace PID SP 1.vi"("PID gains"=w523, "PV deg C"=w524, "User SP Deg C"=w515) -> ("output T SP"=w525:dbl, "Test Probe"=w513:dbl[])  [unwired: 7 in]
            n142 = In Range and Coerce(upper limit=w517, x=w515, lower limit=w518) -> (In Range?=w514:bool)  [unwired: 1 out]
            n143 = Build Array (concatenate)(w512, w513) -> (w511:dbl[])
          }
          frame True {
            # "Initial Temperature Ramp @ 1V"
            n144 = Subtract(x="Furnace 1", y=sgl 10.0) -> (x-y=w540:sgl)
            n145 = Add(x=sgl 10.0, y="Furnace 1") -> (x+y=w542:sgl)
            n146 = Subtract(x="Furnace 2", y=sgl 10.0) -> (x-y=w537:sgl)
            n147 = Add(x=sgl 10.0, y="Furnace 2") -> (x+y=w535:sgl)
            n148 = In Range and Coerce(upper limit=w542, x=w531, lower limit=w540) -> (In Range?=w543:bool)  [unwired: 1 out]
            n149 = In Range and Coerce(upper limit=w535, x=w530, lower limit=w537) -> (In Range?=w534:bool)  [unwired: 1 out]
            n150 = And(x=w543, y=w534) -> (x .and. y?=w529:bool)
          }
        }
        n151 = call "72pt Mov Avg.vi"("Value in"=w441) -> ("Value out"=w440:dbl)  [unwired: 10 in]
        n152 = call "Furnace SP calc.vi"("SP"=w472) -> ("SP&CRC"=w495:u8[])  [unwired: 10 in]
        n153 = call "Furnace SP calc.vi"("SP"=w471) -> ("SP&CRC"=w493:u8[])  [unwired: 10 in]
        n154 = Subtract(x=w440, y=sgl 3.0) -> (x-y=w457:dbl)
        n155 = Add(x=sgl 3.0, y=w440) -> (x+y=w458:dbl)
        n156 = Less?(x=w428, y=sgl 5.0) -> (x < y?=w443:bool)
        n157 = case shown="True" w445 {
          tunnel: w468 -> [_ w557]
          tunnel: w441 -> [_ w556]
          tunnel: w467 -> [_ w555]
          tunnel: [w547 w548] -> w466
          tunnel: [w547 w548] -> w465
          tunnel: w454 -> [_ w554]
          tunnel: w436 -> [_ w553]
          tunnel: w454 -> [_ w552]
          tunnel: w436 -> [_ w551]
          tunnel: [_ w550] -> w439
          frame False {
            w547 = sgl 1.0 ("y")
            # "Initial Fan SP"
          }
          frame True {
            # "Fan Control\nOnce Furnace Reaches SP"
            n158 = call "Invertor rate calc.vi"("PID gains"=w557, "V Max Flow"=w553, "process variable g/s"=w556, "User setpoint g/s"=w554) -> ("output V"=w549:dbl, "Test Probe"=w550:dbl[])  [unwired: 5 in, 1 out]
            n159 = call "Invertor rate calc.vi"("PID gains"=w557, "V Max Flow"=w551, "process variable g/s"=w555, "User setpoint g/s"=w552) -> ()  [unwired: 5 in, 3 out]
            n160 = call "10pt Mov Avg.vi"("Value in"=w549) -> ("Value out"=w548:dbl)  [unwired: 10 in]
          }
        }
        n161 = In Range and Coerce(upper limit=w458, x=w454, lower limit=w457) -> (In Range?=w444:bool)  [unwired: 1 out]
        n162 = Greater Or Equal?(x=w477, y=w476) -> ()  [unwired: 1 out]
        n163 = And(x=w445, y=w444) -> (x .and. y?=w451:bool)
        n164 = Equal To 0?(x=w448) -> (x = 0?=w449:bool)
        n165 = And(x=w451, y=w449) -> (x .and. y?=w450:bool)
        n166 = Compound Arithmetic op=AND(w442, w444, w443) -> (w429:bool)
        "Ready" <- w429
        n167 = case shown="True" w450 {
          tunnel: w448 -> [w509 _]
          tunnel: [w509 1 ("index")] -> w447
          frame False {
          }
          frame True {
            # "Turns on Furnace PID"
          }
        }
        n168 = case shown="True" w429 {
          tunnel: [FALSE "Start Test"] -> w430
          frame False {
          }
          frame True {
          }
        }
        n169 = case shown="True" w461 {
          tunnel: w466 -> [_ w546]
          tunnel: w465 -> [_ w545]
          tunnel: [w544 w546] -> w464
          tunnel: [w544 w545] -> w463
          tunnel: w462 -> [w544 _]
          frame False {
            # "Fan Manual"
          }
          frame True {
          }
        }
        n170 = Build Array (concatenate)(w438, w439) -> (w437:dbl[])
        n171 = case shown="True" w474 {
          tunnel: [w561 w565] -> w483
          tunnel: w495 -> [w561 w565]
          tunnel: [u8[] [64, 160, 0, 0, 133, 108] ("SP&CRC") w563] -> w482
          tunnel: [w560 w564] -> w435
          tunnel: w464 -> [w560 w564]
          tunnel: [0.0 ("element") w562] -> w494
          tunnel: w493 -> [_ w563]
          tunnel: w463 -> [_ w562]
          frame False {
            # "half system"
          }
          frame True {
            # "full system"
          }
        }
        n172 = Build Array(w435, w494) -> (w479:dbl[])
        n173 = Build Array("CO2", "N2", "SO2", "H2O") -> (w485:dbl[])
        n174 = Select(t=3, s=w430, f=2) -> (s? t:f=w506:i32)
        n175 = Build Array (concatenate)(w483, w482) -> (w481:u8[])
        n176 = call "MFR Flow to SP 2-3.vi"("MFC SPs"=w485) -> ("MFC array"=w478:dbl[], "SV Array"=w480:bool[])  [unwired: 9 in]
        n177 = Build Array (concatenate)(w479, w478) -> (w484:dbl[])
      }
      frame 3 {
        # "Test"
        n178 = case shown="1" w663 {
          tunnel: w669 -> [_ _ w765 w794 _ _]
          tunnel: [w693 w726 w771 w815 w1185 w1367] -> w608
          tunnel: w668 -> [_ _ _ _ _ _]
          tunnel: w667 -> [w676 w715 w742 w808 w1159 _]
          tunnel: w666 -> [_ _ _ _ _ _]
          tunnel: [w695 w729 w770 w825 w1227 w1369] -> w665
          tunnel: w664 -> [w691 w727 w769 _ _ _]
          tunnel: w662 -> [_ _ _ _ w1174 w1345]
          tunnel: w661 -> [_ _ _ w824 _ _]
          tunnel: [w692 w725 w773 w821 w1230 0 ("t")] -> w660
          tunnel: w659 -> [_ _ _ w785 _ _]
          tunnel: w658 -> [_ _ _ w822 _ w1352]
          tunnel: [w692 w725 w773 w820 w1230 w1340] -> w657
          tunnel: w656 -> [_ _ _ w819 _ _]
          tunnel: w655 -> [_ _ _ w818 _ _]
          tunnel: w654 -> [w675 w708 w745 w816 w1223 _]
          tunnel: w653 -> [_ _ _ _ w1196 _]
          tunnel: w652 -> [_ _ _ w800 _ _]
          tunnel: w651 -> [_ _ w761 _ _ _]
          tunnel: w650 -> [_ _ w759 _ _ _]
          tunnel: w649 -> [_ _ w760 w805 _ _]
          tunnel: w647 -> [_ _ _ _ _ w1366]
          tunnel: w646 -> [_ _ _ _ _ _]
          tunnel: [0 0 0 0 0 w1349] -> w642
          tunnel: w645 -> [_ _ w758 w807 _ _]
          tunnel: w630 -> [_ _ _ w806 _ _]
          tunnel: w644 -> [_ _ _ _ _ _]
          tunnel: w643 -> [_ _ _ _ _ _]
          tunnel: w641 -> [_ _ _ w801 _ _]
          tunnel: w640 -> [_ _ _ _ w1222 _]
          tunnel: w639 -> [_ _ _ _ w1220 _]
          tunnel: w638 -> [_ _ _ _ _ _]
          tunnel: w637 -> [_ _ _ _ _ _]
          tunnel: w636 -> [_ _ _ _ _ _]
          tunnel: [_ _ _ _ w1189 _] -> w635
          tunnel: w634 -> [_ _ _ _ w1221 _]
          tunnel: [_ _ _ _ w1189 _] -> w633
          tunnel: w632 -> [_ _ _ _ w1219 _]
          tunnel: w631 -> [w680 w704 w743 w795 w1189 _]
          tunnel: [_ _ _ _ w1152 w1361] -> w629
          tunnel: w628 -> [_ _ _ _ _ w1361]
          tunnel: w627 -> [_ _ _ _ w1198 _]
          tunnel: w626 -> [_ _ _ _ w1199 _]
          tunnel: [_ _ _ _ w1195 _] -> w625
          tunnel: [_ _ _ _ w1194 _] -> w624
          tunnel: [_ _ _ _ w1192 _] -> w623
          tunnel: [_ _ _ _ w1193 _] -> w622
          tunnel: w621 -> [_ _ _ _ w1203 _]
          tunnel: w620 -> [_ _ _ _ w1201 _]
          tunnel: w619 -> [_ _ _ _ w1202 _]
          tunnel: w618 -> [_ _ _ _ w1200 _]
          tunnel: w617 -> [_ _ _ w787 w1197 _]
          tunnel: w616 -> [_ _ _ _ w1214 _]
          tunnel: w615 -> [_ _ _ _ w1213 _]
          tunnel: [_ _ _ _ w1210 _] -> w614
          tunnel: [dbl[] [2.75, 27.5, 0.0, 0.0, 0.0] ("MFC SPs") dbl[] [2.75, 27.5, 0.0, 0.0, 0.0] ("MFC SPs") dbl[] [2.75, 27.5, 0.0, 0.0, 0.0] ("MFC SPs") w792 w1206 w1357] -> w612
          tunnel: w611 -> [_ _ _ _ w1205 _]
          tunnel: w610 -> [_ _ _ w788 w1204 _]
          tunnel: [w685 w717 w751 w789 w1186 w1359] -> w609
          tunnel: w605 -> [_ _ _ w784 w1183 _]
          tunnel: w604 -> [w678 w707 w744 _ w1182 _]
          tunnel: w603 -> [_ _ _ _ _ _]
          tunnel: w602 -> [_ _ _ _ w1181 _]
          tunnel: w601 -> [_ _ _ _ _ _]
          tunnel: w600 -> [w674 w706 w740 _ w1173 _]
          tunnel: w599 -> [_ _ _ _ _ w1356]
          tunnel: w598 -> [_ _ _ _ _ w1354]
          tunnel: w597 -> [_ _ w749 w782 w1180 _]
          tunnel: w596 -> [_ _ _ _ _ w1351]
          tunnel: [_ _ _ _ _ w1337] -> w595
          tunnel: w594 -> [_ _ _ _ _ w1335]
          tunnel: [_ _ _ _ _ w1336] -> w593
          tunnel: [_ _ _ _ w1170 _] -> w591
          tunnel: w590 -> [w673 w705 w741 _ w1169 _]
          tunnel: w589 -> [_ _ _ _ _ _]
          tunnel: w585 -> [w670 w713 _ _ w1160 _]
          tunnel: w584 -> [_ _ _ _ w1168 _]
          tunnel: w583 -> [_ _ _ _ w1167 _]
          tunnel: w582 -> [w682 w716 w750 w783 w1164 _]
          tunnel: w581 -> [_ _ _ _ w1163 _]
          tunnel: [_ _ _ _ w1162 _] -> w580
          tunnel: [_ _ _ _ w1161 _] -> w579
          tunnel: w578 -> [w672 w714 w747 _ w1157 _]
          tunnel: [w671 w712 w746 _ w1156 _] -> w577
          tunnel: w576 -> [_ _ _ _ w1151 _]
          frame 0, Default {
            (unwired) 0.0 ("Air MFR")
            (unwired) 0.0 ("HC MFR")
            w692 = u16 0
            # "1Hz MFC's\n\n0. CO2\n1. N2\n2. SO2\n3. H2O\n4. N2P"
            # "CO Light-Off"
            n179 = Greater Or Equal?(x=w682, y=w691) -> (x >= y?=w694:bool)
            n180 = call "Mov_Avg_JS.vi"("Array In"=w672, "Cycle Length"=w670, "Input"=w676) -> ("Array Out Main"=w671:dbl[], "Mean"=w677:dbl)  [unwired: 7 in]
            n181 = case shown="True" w678 {
              tunnel: w677 -> [_ w697]
              tunnel: w675 -> [_ w700]
              tunnel: w674 -> [_ w698]
              tunnel: [w696 w703] -> w679
              tunnel: [w696 w703] -> w681
              tunnel: [_ w702] -> _
              tunnel: w673 -> [_ w699]
              tunnel: w680 -> [w696 _]
              frame False {
                # "Manual Set-point"
              }
              frame True {
                n182 = call "Invertor rate calc.vi"("PID gains"=w700, "V Max Flow"=w699, "process variable g/s"=w697, "User setpoint g/s"=w698) -> ("output V"=w701:dbl, "Test Probe"=w702:dbl[])  [unwired: 5 in, 1 out]
                n183 = call "Invertor rate calc.vi"("PID gains"=w700, "V Max Flow"=w699, "process variable g/s"=w697, "User setpoint g/s"=w698) -> ()  [unwired: 5 in, 3 out]
                n184 = call "10pt Mov Avg.vi"("Value in"=w701) -> ("Value out"=w703:dbl)  [unwired: 10 in]
              }
            }
            n185 = Select(t=4, s=w694, f=3) -> (s? t:f=w695:i32)
            n186 = Build Array(w679, w681) -> (w693:dbl[])
            n187 = call "Furnace SP calc.vi"("SP"=sgl 1000.0) -> ("SP&CRC"=w683:u8[])  [unwired: 10 in]
            n188 = Build Array (concatenate)(w683, u8[] [65, 32, 0, 0, 133, 120] ("SP&CRC")) -> (w685:u8[])
          }
          frame 1 {
            w725 = u16 0
            # "1Hz MFC's\n\n0. CO2\n1. N2\n2. SO2\n3. H2O\n4. N2P"
            # "Need to Review for new injection"
            # "Need to Review for new injection"
            # "HC Light-Off"
            n189 = call "Mov_Avg_JS.vi"("Array In"=w714, "Cycle Length"=w713, "Input"=w715) -> ("Array Out Main"=w712:dbl[], "Mean"=w710:dbl)  [unwired: 7 in]
            n190 = Greater Or Equal?(x=w716, y=w727) -> (x >= y?=w728:bool)
            n191 = case shown="True" w707 {
              tunnel: w710 -> [_ w731]
              tunnel: w708 -> [_ w734]
              tunnel: w706 -> [_ w732]
              tunnel: [w730 w737] -> w711
              tunnel: [w730 w737] -> w709
              tunnel: [_ w736] -> _
              tunnel: w705 -> [_ w733]
              tunnel: w704 -> [w730 _]
              frame False {
                # "Manual Set-point"
              }
              frame True {
                n192 = call "Invertor rate calc.vi"("PID gains"=w734, "V Max Flow"=w733, "process variable g/s"=w731, "User setpoint g/s"=w732) -> ("output V"=w735:dbl, "Test Probe"=w736:dbl[])  [unwired: 5 in, 1 out]
                n193 = call "Invertor rate calc.vi"("PID gains"=w734, "V Max Flow"=w733, "process variable g/s"=w731, "User setpoint g/s"=w732) -> ()  [unwired: 5 in, 3 out]
                n194 = call "10pt Mov Avg.vi"("Value in"=w735) -> ("Value out"=w737:dbl)  [unwired: 10 in]
              }
            }
            n195 = Select(t=4, s=w728, f=3) -> (s? t:f=w729:i32)
            n196 = Build Array(w711, w709) -> (w726:dbl[])
            n197 = call "Furnace SP calc.vi"("SP"=sgl 1000.0) -> ("SP&CRC"=w718:u8[])  [unwired: 10 in]
            n198 = Build Array (concatenate)(w718, u8[] [65, 32, 0, 0, 133, 120] ("SP&CRC")) -> (w717:u8[])
          }
          frame 2 {
            (unwired) 0.0 ("Air MFR")
            w773 = 0 ("t")
            # "NO Light-Off"
            n199 = Multiply(x=w765, y=60.0) -> (x*y=w766:dbl)
            n200 = Divide(x=w766, y=1.2) -> (x/y=w764:dbl)
            n201 = Greater Or Equal?(x=w750, y=w769) -> (x >= y?=w772:bool)
            n202 = call "NOSO2 calc age.vi"("Flow Rate"=w764, "NO/SO2 m ppm"=w749, "NO/SO2 Conc"=w760, "NO/SO2 t ppm"=w761) -> ("NO/SO2 MFR"=w756:dbl)  [unwired: 7 in]
            n203 = call "Mov_Avg_JS.vi"("Array In"=w747, "Input"=w742) -> ("Array Out Main"=w746:dbl[], "Mean"=w748:dbl)  [unwired: 8 in]
            n204 = call "CO calc loff.vi"("CO conc"=w758, "NO conc"=w760, "NO:CO ratio"=w759, "NOx MFR"=w756) -> ()  [unwired: 7 in, 1 out]
            n205 = case shown="True" w744 {
              tunnel: w748 -> [_ w775]
              tunnel: w745 -> [_ w778]
              tunnel: w740 -> [_ w776]
              tunnel: [w774 w781] -> w739
              tunnel: [w774 w781] -> w738
              tunnel: [_ w780] -> _
              tunnel: w741 -> [_ w777]
              tunnel: w743 -> [w774 _]
              frame False {
                # "Manual Set-point"
              }
              frame True {
                n206 = call "Invertor rate calc.vi"("PID gains"=w778, "V Max Flow"=w777, "process variable g/s"=w775, "User setpoint g/s"=w776) -> ("output V"=w779:dbl, "Test Probe"=w780:dbl[])  [unwired: 5 in, 1 out]
                n207 = call "Invertor rate calc.vi"("PID gains"=w778, "V Max Flow"=w777, "process variable g/s"=w775, "User setpoint g/s"=w776) -> ()  [unwired: 5 in, 3 out]
                n208 = call "10pt Mov Avg.vi"("Value in"=w779) -> ("Value out"=w781:dbl)  [unwired: 10 in]
              }
            }
            n209 = Select(t=4, s=w772, f=3) -> (s? t:f=w770:i32)
            n210 = Build Array(w739, w738) -> (w771:dbl[])
            n211 = call "Furnace SP calc.vi"("SP"=sgl 1000.0) -> ("SP&CRC"=w753:u8[])  [unwired: 10 in]
            n212 = Build Array (concatenate)(w753, u8[] [65, 32, 0, 0, 133, 120] ("SP&CRC")) -> (w751:u8[])
          }
          frame 3 {
            (unwired) 0.0 ("Air MFR")
            (unwired) 0.0 ("HC MFR")
            # "Sweep test"
            n213 = case shown="False" w788 {
              tunnel: w787 -> [_ w830]
              tunnel: w783 -> [_ w828]
              tunnel: [w826 w829] -> w786
              tunnel: w785 -> [_ w827]
              tunnel: w784 -> [w826 _]
              frame False {
              }
              frame True {
                n214 = call "Furnace PID SP 1.vi"("PID gains"=w830, "PV deg C"=w828, "User SP Deg C"=w827) -> ("output T SP"=w829:dbl)  [unwired: 7 in, 1 out]
              }
            }
            n215 = call "Invertor rate calc.vi"("PID gains"=w816, "process variable g/s"=w808, "User setpoint g/s"=w794) -> ()  [unwired: 6 in, 3 out]
            n216 = Multiply(x=w794, y=60.0) -> (x*y=w810:dbl)
            n217 = Divide(x=w810, y=1.2) -> (x/y=w793:dbl)
            n218 = Multiply(x=w800, y=1.5 ("Numeric")) -> (x*y=w799:dbl)
            n219 = call "Furnace SP calc.vi"("SP"=w786) -> ("SP&CRC"=w823:u8[])  [unwired: 10 in]
            n220 = call "NOSO2 calc age.vi"("PID"=w801, "Flow Rate"=w793, "NO/SO2 m ppm"=w782, "NO/SO2 Conc"=w805, "NO/SO2 t ppm"=w799) -> ("NO/SO2 MFR"=w809:dbl)  [unwired: 6 in]
            n221 = case shown="4" w824 {
              tunnel: [w835 w860 w893 w936 w958 w993 w1029 w1057 w1092 w1128 dbl[] [0.0, 0.0, 0.0, 0.0, 0.0, 0.0, 0.0, 0.0, 0.0] ("MFC SPs")] -> w814
              tunnel: w823 -> [w837 w856 w894 w934 w957 w991 w1030 w1056 w1091 w1127 w1147]
              tunnel: w795 -> [w836 w861 w895 w935 w956 w992 w1031 w1055 w1090 w1126 w1146]
              tunnel: w822 -> [w850 w875 w909 w939 w973 w1008 w1038 w1070 w1105 w1140 _]
              tunnel: [w847 w870 w904 w945 w968 w1003 w1024 w1065 w1100 w1137 w1150] -> w821
              tunnel: [w843 w869 w903 w943 w967 w1002 w1042 w1064 w1099 w1133 w1150] -> w820
              tunnel: w782 -> [_ w874 w908 w932 w972 w1007 w1036 w1069 w1104 _ _]
              tunnel: w819 -> [_ w868 _ _ _ _ _ w1063 _ _ _]
              tunnel: w818 -> [_ _ _ _ w960 _ _ _ _ _ _]
              tunnel: [FALSE ("s") FALSE ("s") FALSE ("s") FALSE ("s") FALSE ("s") FALSE ("s") FALSE ("s") FALSE ("s") FALSE ("s") FALSE ("s") TRUE ("s")] -> w817
              tunnel: [w837 w856 w894 w934 w957 w991 w1030 w1056 w1091 w1127 w1147] -> w791
              tunnel: [w836 w861 w895 w935 w956 w992 w1031 w1055 w1090 w1126 w1146] -> w797
              tunnel: w793 -> [w833 w859 w892 w927 w955 w990 w1023 w1054 w1089 w1124 _]
              tunnel: w807 -> [w831 w858 w891 w926 w954 w988 w1028 w1053 w1088 w1123 _]
              tunnel: w806 -> [w832 w857 w890 w925 w953 w989 w1027 w1052 w1087 w1122 _]
              frame 0, Default {
                w841 = 1.0 ("C_CO")
                # "0. CO\n1. HC\n2. Air\n3. NO\n4. CO2\n5. N2\n6. SO2\n7. H2O\n8. AirB"
                n222 = Increment(x=w850) -> (x+1=w844:i32)
                n223 = call "CO MFR sw 1.vi"("Bottle conc"=w831, "C_CO"=w841, "Flow rate"=w833) -> ("CO MFR"=w842:dbl)  [unwired: 8 in]
                n224 = call "HC MFR sw 1.vi"("HC Conc %"=w832, "C_HC"=w841, "Flow rate"=w833) -> ("HC MFR"=w840:dbl)  [unwired: 8 in]
                n225 = call "Air MFR sw 1.vi"("C_air"=0.9 ("C_CO"), "Flow rate"=w833) -> ("Air MFR"=w839:dbl)  [unwired: 9 in]
                n226 = Equal?(x=w844, y=20.0) -> (x = y?=w845:bool)
                n227 = Select(t=1, s=w845, f=0) -> (s? t:f=w847:i32)
                n228 = Select(t=0, s=w845, f=w844) -> (s? t:f=w843:i32)
                n229 = Replace Array Subset(array=dbl[] [0.0, 0.0, 0.0, 0.0, 0.0, 0.0, 0.0, 0.0, 0.0] ("MFC SPs"), new element #1=w842, index #1=0 ("index"), new element #2=w840, index #2=1 ("index"), new element #3=w839, index #3=2 ("index")) -> (w835:dbl[])
              }
              frame 1 {
                w864 = 1.75  # C_air
                w863 = 1.0 ("C_CO")
                # "0. CO\n1. HC\n2. Air\n3. NO\n4. CO2\n5. N2\n6. SO2\n7. H2O\n8. AirB"
                # "Timeout"
                # "Lambda measured upstream"
                n230 = Increment(x=w875) -> (x+1=w872:i32)
                n231 = call "CO MFR sw 1.vi"("Bottle conc"=w858, "C_CO"=w863, "Flow rate"=w859) -> ("CO MFR"=w867:dbl)  [unwired: 8 in]
                n232 = call "HC MFR sw 1.vi"("HC Conc %"=w857, "C_HC"=w863, "Flow rate"=w859) -> ("HC MFR"=w866:dbl)  [unwired: 8 in]
                n233 = call "Air MFR sw 1.vi"("C_air"=w864, "Flow rate"=w859) -> ("Air MFR"=w865:dbl)  [unwired: 9 in]
                n234 = Greater Or Equal?(x=w874, y=w868) -> (x >= y?=w871:bool)
                n235 = Equal?(x=w872, y=2000.0) -> (x = y?=w873:bool)
                n236 = case shown="True" w873 {
                  tunnel: [w885 10] -> w870
                  tunnel: [w882 0] -> w869
                  tunnel: w872 -> [w883 _]
                  tunnel: w871 -> [w884 _]
                  frame False {
                    n237 = Select(t=0, s=w884, f=w883) -> (s? t:f=w882:i32)
                    n238 = Select(t=2, s=w884, f=1) -> (s? t:f=w885:i32)
                  }
                  frame True {
                    # "safe case at the end"
                  }
                }
                n239 = Replace Array Subset(array=dbl[] [0.0, 0.0, 0.0, 0.0, 0.0, 0.0, 0.0, 0.0, 0.0] ("MFC SPs"), new element #1=w867, index #1=0 ("index"), new element #2=w866, index #2=1 ("index"), new element #3=w865, index #3=2 ("index")) -> (w860:dbl[])
              }
              frame 2 {
                w897 = 0.0  # C_air
                w898 = 1.5 ("C_CO")
                # "0. CO\n1. HC\n2. Air\n3. NO\n4. CO2\n5. N2\n6. SO2\n7. H2O\n8. AirB"
                # "timeout."
                n240 = Increment(x=w909) -> (x+1=w906:i32)
                n241 = Less Or Equal?(x=w908, y=1.0) -> (x <= y?=w905:bool)
                n242 = Equal?(x=w906, y=2000.0) -> (x = y?=w907:bool)
                n243 = call "CO MFR sw 1.vi"("Bottle conc"=w891, "C_CO"=w898, "Flow rate"=w892) -> ("CO MFR"=w901:dbl)  [unwired: 8 in]
                n244 = call "HC MFR sw 1.vi"("HC Conc %"=w890, "C_HC"=w898, "Flow rate"=w892) -> ("HC MFR"=w900:dbl)  [unwired: 8 in]
                n245 = call "Air MFR sw 1.vi"("C_air"=w897, "Flow rate"=w892) -> ("Air MFR"=w899:dbl)  [unwired: 9 in]
                n246 = case shown="False" w907 {
                  tunnel: [w919 10] -> w904
                  tunnel: [w916 0] -> w903
                  tunnel: w906 -> [w917 _]
                  tunnel: w905 -> [w918 _]
                  frame False {
                    n247 = Select(t=0, s=w918, f=w917) -> (s? t:f=w916:i32)
                    n248 = Select(t=3, s=w918, f=2) -> (s? t:f=w919:i32)
                  }
                  frame True {
                    # "safe case at the end"
                  }
                }
                n249 = Replace Array Subset(array=dbl[] [0.0, 0.0, 0.0, 0.0, 0.0, 0.0, 0.0, 0.0, 0.0] ("MFC SPs"), new element #1=w901, index #1=0 ("index"), new element #2=w900, index #2=1 ("index"), new element #3=w899, index #3=2 ("index")) -> (w893:dbl[])
              }
              frame 3 {
                w924 = 1.5 ("C_CO")
                # "0. CO\n1. HC\n2. Air\n3. NO\n4. CO2\n5. N2\n6. SO2\n7. H2O\n8. AirB"
                n250 = Less Or Equal?(x=w932, y=0.98) -> (x <= y?=w931:bool)
                n251 = Increment(x=w939) -> (x+1=w938:i32)
                n252 = call "CO MFR sw 2.vi"("Increment"=w938, "Bottle conc"=w926, "C_CO"=w924, "Flow rate"=w927) -> ("CO MFR"=w942:dbl)  [unwired: 7 in]
                n253 = call "HC MFR sw 2.vi"("Increment"=w938, "HC Conc %"=w925, "C_HC"=w924, "Flow rate"=w927) -> ("HC MFR"=w941:dbl)  [unwired: 7 in]
                n254 = call "Air MFR sw 2.vi"("Increment"=w938, "C_air"=0.0 ("C_CO"), "Flow rate"=w927) -> ("Air MFR"=w940:dbl)  [unwired: 8 in]
                n255 = Equal?(x=w938, y=1200.0) -> (x = y?=w930:bool)
                n256 = Or(x=w931, y=w930) -> (x .or. y?=w929:bool)
                n257 = Select(t=4, s=w929, f=3) -> (s? t:f=w945:i32)
                n258 = Replace Array Subset(array=dbl[] [0.0, 0.0, 0.0, 0.0, 0.0, 0.0, 0.0, 0.0, 0.0] ("MFC SPs"), new element #1=w942, index #1=0 ("index"), new element #2=w941, index #2=1 ("index"), new element #3=w940, index #3=2 ("index")) -> (w936:dbl[])
                n259 = Select(t=0, s=w929, f=w938) -> (s? t:f=w943:i32)
              }
              frame 4 {
                w961 = 1.0  # C_HC
                w962 = 1.0  # C_CO
                w963 = 0.3  # C_air
                # "0. CO\n1. HC\n2. Air\n3. NO\n4. CO2\n5. N2\n6. SO2\n7. H2O\n8. AirB"
                n260 = Less Or Equal?(x=w972, y=w960) -> (x <= y?=w969:bool)
                n261 = Increment(x=w973) -> (x+1=w970:i32)
                n262 = Equal?(x=w970, y=2000.0) -> (x = y?=w971:bool)
                n263 = call "HC MFR sw 1.vi"("HC Conc %"=w953, "C_HC"=w961, "Flow rate"=w955) -> ("HC MFR"=w965:dbl)  [unwired: 8 in]
                n264 = call "CO MFR sw 1.vi"("Bottle conc"=w954, "C_CO"=w962, "Flow rate"=w955) -> ("CO MFR"=w966:dbl)  [unwired: 8 in]
                n265 = call "Air MFR sw 1.vi"("C_air"=w963, "Flow rate"=w955) -> ("Air MFR"=w964:dbl)  [unwired: 9 in]
                n266 = case shown="True" w971 {
                  tunnel: [w983 10] -> w968
                  tunnel: [w980 0] -> w967
                  tunnel: w970 -> [w981 _]
                  tunnel: w969 -> [w982 _]
                  frame False {
                    n267 = Select(t=0, s=w982, f=w981) -> (s? t:f=w980:i32)
                    n268 = Select(t=5, s=w982, f=4) -> (s? t:f=w983:i32)
                  }
                  frame True {
                    # "safe case at the end"
                  }
                }
                n269 = Replace Array Subset(array=dbl[] [0.0, 0.0, 0.0, 0.0, 0.0, 0.0, 0.0, 0.0, 0.0] ("MFC SPs"), new element #1=w966, index #1=0 ("index"), new element #2=w965, index #2=1 ("index"), new element #3=w964, index #3=2 ("index")) -> (w958:dbl[])
              }
              frame 5 {
                w996 = 0.3  # C_HC
                w997 = 0.5  # C_CO
                w998 = 0.5  # C_air
                # "0. CO\n1. HC\n2. Air\n3. NO\n4. CO2\n5. N2\n6. SO2\n7. H2O\n8. AirB"
                n270 = Greater Or Equal?(x=w1007, y=0.97) -> (x >= y?=w1004:bool)
                n271 = Increment(x=w1008) -> (x+1=w1005:i32)
                n272 = Equal?(x=w1005, y=2000.0) -> (x = y?=w1006:bool)
                n273 = call "Air MFR sw 1.vi"("C_air"=w998, "Flow rate"=w990) -> ("Air MFR"=w999:dbl)  [unwired: 9 in]
                n274 = call "CO MFR sw 1.vi"("Bottle conc"=w988, "C_CO"=w997, "Flow rate"=w990) -> ("CO MFR"=w1001:dbl)  [unwired: 8 in]
                n275 = call "HC MFR sw 1.vi"("HC Conc %"=w989, "C_HC"=w996, "Flow rate"=w990) -> ("HC MFR"=w1000:dbl)  [unwired: 8 in]
                n276 = case shown="False" w1006 {
                  tunnel: [w1018 10] -> w1003
                  tunnel: [w1015 0] -> w1002
                  tunnel: w1005 -> [w1016 _]
                  tunnel: w1004 -> [w1017 _]
                  frame False {
                    n277 = Select(t=0, s=w1017, f=w1016) -> (s? t:f=w1015:i32)
                    n278 = Select(t=6, s=w1017, f=5) -> (s? t:f=w1018:i32)
                  }
                  frame True {
                    # "safe case at the end"
                  }
                }
                n279 = Replace Array Subset(array=dbl[] [0.0, 0.0, 0.0, 0.0, 0.0, 0.0, 0.0, 0.0, 0.0] ("MFC SPs"), new element #1=w1001, index #1=0 ("index"), new element #2=w1000, index #2=1 ("index"), new element #3=w999, index #3=2 ("index")) -> (w993:dbl[])
              }
              frame 6 {
                # "0. CO\n1. HC\n2. Air\n3. NO\n4. CO2\n5. N2\n6. SO2\n7. H2O\n8. AirB"
                n280 = Increment(x=w1038) -> (x+1=w1033:i32)
                n281 = Greater Or Equal?(x=w1036, y=1.0) -> (x >= y?=w1034:bool)
                n282 = call "CO MFR sw 3.vi"("Increment"=w1033, "Bottle conc"=w1028, "C_CO"=0.75, "Flow rate"=w1023) -> ("CO MFR"=w1041:dbl)  [unwired: 7 in]
                n283 = call "HC MFR sw 3.vi"("Increment"=w1033, "HC Conc %"=w1027, "C_HC"=0.5, "Flow rate"=w1023) -> ("CO MFR"=w1040:dbl)  [unwired: 7 in]
                n284 = call "Air MFR sw 3.vi"("Increment"=w1033, "C_air"=0.65, "Flow rate"=w1023) -> ("Air MFR"=w1039:dbl)  [unwired: 8 in]
                n285 = Replace Array Subset(array=dbl[] [0.0, 0.0, 0.0, 0.0, 0.0, 0.0, 0.0, 0.0, 0.0] ("MFC SPs"), new element #1=w1041, index #1=0 ("index"), new element #2=w1040, index #2=1 ("index"), new element #3=w1039, index #3=2 ("index")) -> (w1029:dbl[])
                n286 = Select(t=0, s=w1034, f=w1033) -> (s? t:f=w1042:i32)
                n287 = Select(t=7, s=w1034, f=6) -> (s? t:f=w1024:i32)
              }
              frame 7 {
                w1059 = 1.75  # C_air
                # "0. CO\n1. HC\n2. Air\n3. NO\n4. CO2\n5. N2\n6. SO2\n7. H2O\n8. AirB"
                # "Lambda measured upstream"
                n288 = Increment(x=w1070) -> (x+1=w1067:i32)
                n289 = Greater Or Equal?(x=w1069, y=w1063) -> (x >= y?=w1066:bool)
                n290 = Equal?(x=w1067, y=2000.0) -> (x = y?=w1068:bool)
                n291 = call "Air MFR sw 1.vi"("C_air"=w1059, "Flow rate"=w1054) -> ("Air MFR"=w1060:dbl)  [unwired: 9 in]
                n292 = call "CO MFR sw 1.vi"("Bottle conc"=w1053, "C_CO"=1.0, "Flow rate"=w1054) -> ("CO MFR"=w1062:dbl)  [unwired: 8 in]
                n293 = call "HC MFR sw 1.vi"("HC Conc %"=w1052, "C_HC"=1.0, "Flow rate"=w1054) -> ("HC MFR"=w1061:dbl)  [unwired: 8 in]
                n294 = case shown="False" w1068 {
                  tunnel: [w1080 10] -> w1065
                  tunnel: [w1077 0] -> w1064
                  tunnel: w1067 -> [w1078 _]
                  tunnel: w1066 -> [w1079 _]
                  frame False {
                    n295 = Select(t=0, s=w1079, f=w1078) -> (s? t:f=w1077:i32)
                    n296 = Select(t=8, s=w1079, f=7) -> (s? t:f=w1080:i32)
                  }
                  frame True {
                    # "safe case at the end"
                  }
                }
                n297 = Replace Array Subset(array=dbl[] [0.0, 0.0, 0.0, 0.0, 0.0, 0.0, 0.0, 0.0, 0.0] ("MFC SPs"), new element #1=w1062, index #1=0 ("index"), new element #2=w1061, index #2=1 ("index"), new element #3=w1060, index #3=2 ("index")) -> (w1057:dbl[])
              }
              frame 8 {
                w1095 = 0.0  # C_air
                # "0. CO\n1. HC\n2. Air\n3. NO\n4. CO2\n5. N2\n6. SO2\n7. H2O\n8. AirB"
                # "Lambda measured upstream"
                n298 = Increment(x=w1105) -> (x+1=w1102:i32)
                n299 = Less Or Equal?(x=w1104, y=1.0) -> (x <= y?=w1101:bool)
                n300 = Equal?(x=w1102, y=1500.0) -> (x = y?=w1103:bool)
                n301 = call "CO MFR sw 1.vi"("Bottle conc"=w1088, "C_CO"=1.5, "Flow rate"=w1089) -> ("CO MFR"=w1098:dbl)  [unwired: 8 in]
                n302 = call "HC MFR sw 1.vi"("HC Conc %"=w1087, "C_HC"=1.5, "Flow rate"=w1089) -> ("HC MFR"=w1097:dbl)  [unwired: 8 in]
                n303 = call "Air MFR sw 1.vi"("C_air"=w1095, "Flow rate"=w1089) -> ("Air MFR"=w1096:dbl)  [unwired: 9 in]
                n304 = case shown="False" w1103 {
                  tunnel: [w1115 10] -> w1100
                  tunnel: [w1112 0] -> w1099
                  tunnel: w1102 -> [w1113 _]
                  tunnel: w1101 -> [w1114 _]
                  frame False {
                    n305 = Select(t=0, s=w1114, f=w1113) -> (s? t:f=w1112:i32)
                    n306 = Select(t=9, s=w1114, f=8) -> (s? t:f=w1115:i32)
                  }
                  frame True {
                    # "safe case at the end"
                  }
                }
                n307 = Replace Array Subset(array=dbl[] [0.0, 0.0, 0.0, 0.0, 0.0, 0.0, 0.0, 0.0, 0.0] ("MFC SPs"), new element #1=w1098, index #1=0 ("index"), new element #2=w1097, index #2=1 ("index"), new element #3=w1096, index #3=2 ("index")) -> (w1092:dbl[])
              }
              frame 9 {
                # "0. CO\n1. HC\n2. Air\n3. NO\n4. CO2\n5. N2\n6. SO2\n7. H2O\n8. AirB"
                n308 = Increment(x=w1140) -> (x+1=w1134:i32)
                n309 = Equal?(x=w1134, y=120.0) -> (x = y?=w1135:bool)
                n310 = call "Air MFR sw 1.vi"("C_air"=0.9 ("C_CO"), "Flow rate"=w1124) -> ("Air MFR"=w1130:dbl)  [unwired: 9 in]
                n311 = call "CO MFR sw 1.vi"("Bottle conc"=w1123, "C_CO"=1.0, "Flow rate"=w1124) -> ("CO MFR"=w1132:dbl)  [unwired: 8 in]
                n312 = call "HC MFR sw 1.vi"("HC Conc %"=w1122, "C_HC"=1.0, "Flow rate"=w1124) -> ("HC MFR"=w1131:dbl)  [unwired: 8 in]
                n313 = Select(t=10, s=w1135, f=9) -> (s? t:f=w1137:i32)
                n314 = Replace Array Subset(array=dbl[] [0.0, 0.0, 0.0, 0.0, 0.0, 0.0, 0.0, 0.0, 0.0] ("MFC SPs"), new element #1=w1132, index #1=0 ("index"), new element #2=w1131, index #2=1 ("index"), new element #3=w1130, index #3=2 ("index")) -> (w1128:dbl[])
                n315 = Select(t=0, s=w1135, f=w1134) -> (s? t:f=w1133:i32)
              }
              frame 10 {
                w1150 = 0
                # "0. CO\n1. HC\n2. Air\n3. NO\n4. CO2\n5. N2\n6. SO2\n7. H2O\n8. AirB"
              }
            }
            n316 = Replace Array Subset(array=w814, new element=w809, index=3) -> (w792:dbl[])
            n317 = Build Array(w797, 0.0 ("x")) -> (w815:dbl[])
            n318 = Select(t=4, s=w817, f=3) -> (s? t:f=w825:i32)
            n319 = Build Array (concatenate)(w791, u8[] [65, 32, 0, 0, 133, 120] ("SP&CRC")) -> (w789:u8[])
          }
          frame 4 {
            (unwired) 0.0 ("Air MFR")
            (unwired) 0.0 ("HC MFR")
            w1184 = 0.0 ("element")
            w1230 = 0
            # "Press Alarm"
            # "O2 Alarm"
            # "1Hz MFC's\n\n0. CO2\n1. N2\n2. SO2\n3. H2O\n4. N2P"
            # "last value of the fan"
            # "Original\n0. CO - x\n1. HC - x\n2. Air - x\n3. NO - x\n4. CO2 \n5. N2\n6. SO2\n7. H2O\n8. AirB - x"
            # "NO"
            # "Ageing Test"
            n320 = call "60pt Mov Avg.vi"("Value in"=w1180) -> ("Value out"=w1179:dbl)  [unwired: 10 in]
            "Uego Avg" <- w1179
            n321 = call "Mov_Avg_JS_Dual.vi"("Cycle Length"=w1160, "Array In 2"=w1167, "Input 2"=w1163, "Array In"=w1168, "Input"=w1164) -> ("Array Out Main 2"=w1161:dbl[], "Mean 2"=w1165:dbl, "Array Out Main"=w1162:dbl[], "Mean"=w1166:dbl)  [unwired: 3 in]
            n322 = call "Mov_Avg_JS.vi"("Array In"=w1157, "Cycle Length"=w1160, "Input"=w1159) -> ("Array Out Main"=w1156:dbl[], "Mean"=w1158:dbl)  [unwired: 7 in]
            n323 = Greater?(x=w1174, y="Press Up Limit") -> (0:w1175:bool)
            n324 = Less?(x=w1174, y="Press Low Limit") -> (x < y?=w1176:bool)
            n325 = Greater?(x=w1179, y="O2 Up Limit") -> (0:w1218:bool)
            n326 = Less?(x=w1179, y="O2 Low Limit") -> (x < y?=w1217:bool)
            n327 = Or(x=w1175, y=w1176) -> (x .or. y?=w1155:bool)
            n328 = Or(x=w1218, y=w1217) -> (x .or. y?=w1154:bool)
            n329 = case shown="False" w1204 {
              tunnel: [w1252 w1308] -> w1192
              tunnel: [w1253 w1307] -> w1193
              tunnel: [w1251 w1309] -> w1195
              tunnel: [w1250 w1310] -> w1194
              tunnel: w1203 -> [w1248 w1309]
              tunnel: w1202 -> [w1247 _]
              tunnel: w1201 -> [w1246 w1310]
              tunnel: w1200 -> [w1245 _]
              tunnel: w1166 -> [w1240 _]
              tunnel: w1198 -> [w1239 _]
              tunnel: w1199 -> [w1235 _]
              tunnel: w1165 -> [w1234 _]
              tunnel: w1197 -> [w1232 _]
              tunnel: w1196 -> [w1233 _]
              tunnel: w1183 -> [_ w1308]
              tunnel: w1181 -> [_ w1307]
              tunnel: [w1231 _] -> w1172
              frame False {
                n330 = case shown="False" "Furnace Open Loop" {
                  tunnel: "Furnace Control VI" -> [w1275 _]
                  tunnel: [w1274 w1305] -> w1251
                  tunnel: [w1273 w1306] -> w1250
                  tunnel: [w1272 w1304] -> w1252
                  tunnel: [w1271 w1303] -> w1253
                  tunnel: w1233 -> [w1270 _]
                  tunnel: w1246 -> [w1269 w1306]
                  tunnel: w1239 -> [w1268 _]
                  tunnel: w1235 -> [w1267 _]
                  tunnel: w1247 -> [w1266 w1304]
                  tunnel: w1245 -> [w1265 w1303]
                  tunnel: "Furnace 1 Baseline" -> [w1264 _]
                  tunnel: "Counter Interval 1" -> [w1263 _]
                  tunnel: "Counter Interval 2" -> [w1262 _]
                  tunnel: w1232 -> [w1261 _]
                  tunnel: w1248 -> [w1260 w1305]
                  tunnel: "BED TARGET" -> [w1259 _]
                  tunnel: "BED TARGET 2" -> [w1258 _]
                  tunnel: w1234 -> [w1257 _]
                  tunnel: w1240 -> [w1256 _]
                  tunnel: "Furnace 2 Baseline" -> [w1255 _]
                  tunnel: [w1254 _] -> w1231
                  frame False {
                    # "Closed Loop"
                    n331 = case shown="False" w1275 {
                      tunnel: w1270 -> [w1278 _]
                      tunnel: [w1285 w1302] -> w1272
                      tunnel: [w1276 w1301] -> w1271
                      tunnel: [_ w1300] -> w1274
                      tunnel: [_ w1299] -> w1273
                      tunnel: w1260 -> [_ w1298]
                      tunnel: w1266 -> [_ w1297]
                      tunnel: w1259 -> [w1284 w1296]
                      tunnel: w1258 -> [w1280 w1295]
                      tunnel: w1269 -> [_ w1294]
                      tunnel: w1265 -> [_ w1293]
                      tunnel: w1257 -> [w1279 w1292]
                      tunnel: w1256 -> [w1283 w1291]
                      tunnel: w1267 -> [_ w1290]
                      tunnel: w1268 -> [_ w1289]
                      tunnel: w1264 -> [_ _]
                      tunnel: w1263 -> [_ w1288]
                      tunnel: w1262 -> [_ w1287]
                      tunnel: w1261 -> [w1286 _]
                      tunnel: w1255 -> [_ _]
                      tunnel: [w1281 _] -> w1254
                      frame False {
                        # "Furnace PID"
                        n332 = call "Furnace PID SP 1.vi"("PID gains"=w1278, "PV deg C"=w1279, "User SP Deg C"=w1280) -> ("output T SP"=w1276:dbl, "Test Probe"=w1277:dbl[])  [unwired: 7 in]
                        n333 = call "Furnace PID SP 1.vi"("PID gains"=w1286, "PV deg C"=w1283, "User SP Deg C"=w1284) -> ("output T SP"=w1285:dbl, "Test Probe"=w1282:dbl[])  [unwired: 7 in]
                        n334 = Build Array (concatenate)(w1282, w1277) -> (w1281:dbl[])
                      }
                      frame True {
                        # "Furnace VI"
                        n335 = call "Furnace_Control_2.vi"("T Furnace"=w1289, "Counter Interval"=w1288, "T Cat"=w1291, "T Set-Point"=w1296, "Furnace Set-point"=w1297, "Counter In"=w1298) -> ("Furnace Set-point"=w1302:dbl, "Counter Out"=w1300:i32)  [unwired: 4 in]
                        n336 = call "Furnace_Control_2.vi"("T Furnace"=w1290, "Counter Interval"=w1287, "T Cat"=w1292, "T Set-Point"=w1295, "Furnace Set-point"=w1293, "Counter In"=w1294) -> ("Furnace Set-point"=w1301:dbl, "Counter Out"=w1299:i32)  [unwired: 4 in]
                      }
                    }
                  }
                  frame True {
                    # "Open Loop\n(Uses last value)"
                  }
                }
              }
              frame True {
                # "Furnace Manual Mode"
              }
            }
            n337 = Decrement(x=w1213) -> (x-1=w1212:dbl)
            n338 = case shown="True" w1182 {
              tunnel: w1158 -> [_ w1318]
              tunnel: w1223 -> [_ w1321]
              tunnel: w1173 -> [_ w1319]
              tunnel: [w1317 w1324] -> w1191
              tunnel: w1221 -> [_ _]
              tunnel: w1220 -> [_ _]
              tunnel: [w1317 w1324] -> w1190
              tunnel: w1219 -> [_ _]
              tunnel: w1189 -> [w1317 _]
              tunnel: [_ w1323] -> w1171
              tunnel: w1169 -> [_ w1320]
              frame False {
                # "Manual Set-point"
              }
              frame True {
                n339 = call "Invertor rate calc.vi"("PID gains"=w1321, "V Max Flow"=w1320, "process variable g/s"=w1318, "User setpoint g/s"=w1319) -> ("output V"=w1322:dbl, "Test Probe"=w1323:dbl[])  [unwired: 5 in, 1 out]
                n340 = call "Invertor rate calc.vi"("PID gains"=w1321, "V Max Flow"=w1320, "process variable g/s"=w1318, "User setpoint g/s"=w1319) -> ()  [unwired: 5 in, 3 out]
                n341 = call "10pt Mov Avg.vi"("Value in"=w1322) -> ("Value out"=w1324:dbl)  [unwired: 10 in]
              }
            }
            n342 = Build Array(w1155, w1154) -> (w1153:bool[])
            n343 = Boolean Array To Number(Boolean array=w1153) -> (number=w1152:u32)
            n344 = case shown="True" w1214 {
              tunnel: w1212 -> [w1312 w1316]
              tunnel: [w1311 w1313] -> w1211
              tunnel: [w1312 w1316] -> w1210
              tunnel: w1205 -> [_ w1314]
              tunnel: w1151 -> [_ w1315]
              frame False {
                n345 = Less Or Equal To 0?(x=w1312) -> (x <= 0?=w1311:bool)
              }
              frame True {
                n346 = Greater Or Equal?(x=w1315, y=w1314) -> (x >= y?=w1313:bool)
              }
            }
            n347 = Build Array (concatenate)(w1172, w1171) -> (w1170:dbl[])
            n348 = call "Furnace SP calc.vi"("SP"=w1192) -> ("SP&CRC"=w1225:u8[])  [unwired: 10 in]
            n349 = call "Furnace SP calc.vi"("SP"=w1193) -> ("SP&CRC"=w1224:u8[])  [unwired: 10 in]
            n350 = case shown="True" w1222 {
              tunnel: [w1328 w1332] -> w1188
              tunnel: w1225 -> [w1328 w1332]
              tunnel: [u8[] [65, 32, 0, 0, 133, 120] ("SP&CRC") w1330] -> w1187
              tunnel: [w1327 w1331] -> w1209
              tunnel: w1191 -> [w1327 w1331]
              tunnel: [0.0 ("element") w1329] -> w1208
              tunnel: w1224 -> [_ w1330]
              tunnel: w1190 -> [_ w1329]
              frame False {
                # "Half System"
              }
              frame True {
                # "Full System"
              }
            }
            n351 = Build Array(w1184, "N2 Age", w1184, w1184, w1184) -> (w1206:dbl[])
            n352 = Build Array(w1209, w1208) -> (w1185:dbl[])
            n353 = Select(t=4 ("s? t:f"), s=w1211, f=3 ("s? t:f")) -> (s? t:f=w1227:i32)
            n354 = Build Array (concatenate)(w1188, w1187) -> (w1186:u8[])
          }
          frame 5 {
            (unwired) 0.0 ("Air MFR")
            (unwired) 0.0 ("HC MFR")
            w1346 = FALSE ("ISO6_SV")
            w1362 = 0.0 ("User Flow rate")
            # "leak test"
            n355 = Increment(x=w1352) -> (x+1=w1340:i32)
            n356 = xnode "Read/Write Control"("FPGA VI Reference In"=w1366, "Leak test on?"=w1346, "DO On?"=TRUE ("ISO6_SV"), "CUToff 1"=w1346, "CUToff 2"=w1346) -> ()  [unwired: 1 in, 2 out]
            n357 = local write "TankHi"(10.0 ("TankHi")) -> ()
            n358 = local write "TankLo"(9.0 ("TankHi")) -> ()
            n359 = Equal To 0?(x=w1335) -> (x = 0?=w1341:bool)
            n360 = Greater Or Equal?(x=w1345, y=9.0) -> (x >= y?=w1342:bool)
            n361 = And(x=w1342, y=w1341) -> (x .and. y?=w1343:bool)
            n362 = case shown="True" w1343 {
              tunnel: w1340 -> [_ w1371]
              tunnel: [w1370 1.0 ("y")] -> w1337
              tunnel: w1335 -> [w1370 _]
              frame False {
              }
              frame True {
                "Press Time" <- w1371
              }
            }
            n363 = Greater Or Equal?(x=w1352, y=w1351) -> (x >= y?=w1353:bool)
            n364 = case shown="True" w1353 {
              tunnel: w1345 -> [_ w1377]
              tunnel: [0 ("length") w1379] -> w1349
              tunnel: 9.0 ("y") -> [_ w1376]
              tunnel: [FALSE TRUE] -> w1347
              frame False {
              }
              frame True {
                n365 = Greater Or Equal?(x=w1377, y=w1376) -> (x >= y?=w1378:bool)
                n366 = case shown="True" w1378 {
                  tunnel: [1 ("length") 2 ("length")] -> w1379
                  frame False {
                  }
                  frame True {
                  }
                }
              }
            }
            n367 = local read "Press Time"() -> (w1339:i32)
            n368 = Build Array(w1362, w1362) -> (w1367:dbl[])
            n369 = Not Equal To 0?(x=w1337) -> (x != 0?=w1338:bool)
            n370 = Select(t=w1339, s=w1338, f=w1340) -> (s? t:f=w1336:i32)
            n371 = case shown="True" TRUE {
              tunnel: [dbl[] [0.0, 0.0, 0.0, 0.0, 0.0] ("MFC SPs") dbl[] [0.0, 50.0, 0.0, 0.0, 0.0] ("MFC SPs")] -> w1357
              frame False {
              }
              frame True {
              }
            }
            n372 = Greater Or Equal?(x=w1340, y=w1356) -> (x >= y?=w1355:bool)
            n373 = Select(t=5 ("s? t:f"), s=w1347, f=3 ("s? t:f")) -> (s? t:f=w1369:i32)
            n374 = case shown="False" w1355 {
              tunnel: w1345 -> [_ w1385]
              tunnel: [0 ("length") w1384] -> _
              tunnel: w1354 -> [_ w1383]
              frame False {
              }
              frame True {
                n375 = Greater?(x=w1385, y=w1383) -> (0:w1386:bool)
                n376 = Select(t=2 ("length"), s=w1386, f=1 ("length")) -> (s? t:f=w1384:i32)
              }
            }
            n377 = call "Furnace SP calc.vi"("SP"=sgl 5.0) -> ("SP&CRC"=w1360:u8[])  [unwired: 10 in]
            n378 = Build Array (concatenate)(w1360, w1360) -> (w1359:u8[])
          }
        }
        n379 = call "MFR Flow to SP 2-3.vi"("MFC SPs"=w612) -> ("MFC array"=w607:dbl[], "SV Array"=w606:bool[])  [unwired: 9 in]
        n380 = Build Array (concatenate)(w608, w607) -> (w613:dbl[])
      }
      frame 4 {
        w1415 = 0
        # "1Hz MFC's\n\n0. CO2\n1. N2\n2. SO2\n3. H2O\n4. N2P"
        # "0. CO\n3. NO\n4. CO2\n5. N2\n6. SO2\n7. H2O"
        # "Shutdown/cooldown"
        # "follow condition \nthen go to standby"
        n381 = Decrement(x=w1392) -> (x-1=w1391:dbl)
        n382 = call "Invertor rate calc.vi"("PID gains"=w1414, "process variable g/s"=w1411, "User setpoint g/s"=10.0 ("User Flow rate")) -> ()  [unwired: 6 in, 3 out]
        n383 = Less Or Equal?(x=w1391, y=0.0) -> (x <= y?=w1407:bool)
        n384 = Select(t=5, s=w1407, f=4) -> (s? t:f=w1417:i32)
        n385 = local write "TankHi"(0.5 ("TankHi")) -> ()
        n386 = local write "TankLo"(0.0 ("TankHi")) -> ()
        n387 = call "Furnace SP calc.vi"("SP"=sgl 10.0) -> ("SP&CRC"=w1400:u8[])  [unwired: 10 in]
        n388 = Build Array (concatenate)(w1400, w1400) -> (w1399:u8[])
        n389 = call "MFR Flow to SP 2-3.vi"("MFC SPs"=dbl[] [0.0, 27.5, 0.0, 0.0, 0.0]) -> ("MFC array"=w1398:dbl[], "SV Array"=w1397:bool[])  [unwired: 9 in]
        n390 = Build Array (concatenate)(w1405, w1405, w1398) -> (w1416:dbl[])
      }
      frame 5 {
        w1418 = 0.0 ("Sw time")
        w1427 = FALSE ("DO On?")
        w1433 = u16 0 ("length")
        # "Off"
        n391 = xnode "Read/Write Control"("FPGA VI Reference In"=w1434, "Command"=2, "DO On?"=w1427, "Leak test on?"=w1427, "CUToff 1"=w1427) -> ()  [unwired: 1 in, 2 out]
        n392 = shared-variable "RT CompactRIO Target 2\\Library 1.lvlib\\Enum 1"(u16 0 ("Enum 1")) -> ()  [unwired: 1 in, 1 out]
        n393 = call "MFR Flow to SP 2-3.vi"("MFC SPs"=dbl[] [0.0, 0.0, 0.0, 0.0, 0.0]) -> ("MFC array"=w1423:dbl[])  [unwired: 9 in, 1 out]
        n394 = Build Array (concatenate)(dbl[] [0.0, 0.0] ("element"), w1423) -> (w1420:dbl[])
      }
    }
    "MFC SV Array" <- w239
    n395 = Index Array(array=w110) -> (element #1=→"Ageing Time":dbl, element #2=→"Remaining Time":dbl, element #3=→"Complete":dbl, element #4=→"% Complete":dbl)  [unwired: 4 in]
    n396 = Index Array(array=w105) -> (element #1=→"Ageing Time 2":dbl, element #2=→"Remaining Time 2":dbl, element #3=→"Complete 2":dbl, element #4=→"% Complete 2":dbl)  [unwired: 4 in]
    n397 = Index Array(array=w104) -> (element #1=→"Ageing Time 3":dbl, element #2=→"Remaining Time 3":dbl, element #3=→"Complete 3":dbl, element #4=→"% Complete 3":dbl)  [unwired: 4 in]
    n398 = Index Array(array=w99) -> (element #1=→"Ageing Time 4":dbl, element #2=→"Remaining Time 4":dbl, element #3=→"Complete 4":dbl, element #4=→"% Complete 4":dbl)  [unwired: 4 in]
    n399 = Build Array (concatenate)(w350, w328, w218, w202, w115) -> (w359:dbl[])
    n400 = xnode "Read/Write Control"("FPGA VI Reference In"=w182, "Furnace Array Out"=w243) -> ("FPGA VI Reference Out"=w242:refnum<k20>, "error out"=w241:errorcluster)  [unwired: 1 in]
    n401 = shared-variable "RT CompactRIO Target 2\\Library 1.lvlib\\DATA"(w359) -> ()  [unwired: 1 in, 1 out]
    n402 = xnode "Read/Write Control"("FPGA VI Reference In"=w231, "Output Array"=w240) -> ()  [unwired: 1 in, 2 out]
    n403 = node-c288() -> ()  [unwired: 1 in, 1 out]
    "Test Start" <- w364
  }
  n404 = timed-loop {
    timing: w39 -> [_]
    timing-out: [_] -> w38
    shift-right: [w1594] -> _
    shift-left: w26 -> [w1595]
    shift-right: [w1592] -> _
    shift-left: 0 -> [w1593]
    shift-right: [w1590] -> _
    shift-left: 3 -> [w1591]
    shift-right: [w1588] -> _
    shift-left: 1 -> [w1589]
    shift-right: [w1586] -> _
    shift-left: 1 -> [w1587]
    shift-right: [w1584] -> _
    shift-left: 1 -> [w1585]
    shift-right: [w1581] -> _
    shift-left: 1 -> [w1583]
    shift-right: [w1580] -> _
    shift-left: 0 -> [w1582]
    shift-right: [w1578] -> _
    shift-left: w26 -> [w1579]
    shift-right: [w1576] -> _
    shift-left: 0 ("t") -> [w1577]
    tunnel: w30 -> [w1504]
    tunnel: w23 -> [w1519]
    shift-right: [w1554] -> _
    shift-left: i32[] [0, 0, 3, 1, 1, 1, 1, 0] -> [w1555]
    tunnel: w23 -> [w1462]
    tunnel: w2 -> [w1514]
    tunnel: w2 -> [w1492]
    tunnel: w19 -> [w1491]
    shift-right: [w1460] -> _
    shift-left: _ -> [w1461]
    shift-right: [w1458] -> _
    shift-left: _ -> [w1459]
    shift-right: [w1457] -> _
    shift-left: _ -> [w1456]
    stop <- w1611 stop-if-true
    # "Cat 4"
    # "Cat 3"
    # "Cat 2"
    # "Cat 1"
    # "MFC Error Display"
    # "10 Hz MFC's\n0. CO\n1. HC_1\n2. Air_1\n3. NO\n4. Air_B\n5. HC_B\n6. Air_2\n7. HC_2"
    # "MFC's\n00. CO\n01. HC _1\n02. Air_1\n03. NO\n04. CO2\n05. N2\n06. SO2\n07. H2O\n08. Air_B\n09.HC_B\n10. Air_2\n11. N2P\n12. HC_2"
    n405 = node-c288() -> (→"Iteration \nDuration 3":i64)  [unwired: 1 in, 2 out]
    n406 = local read "UEGO Sensor Results 2"() -> (w1452:T2)
    n407 = local read "UEGO Sensor Results"() -> (w1571:T2)
    n408 = xnode "Read/Write Control"("FPGA VI Reference In"=w1492, "error in"=w1491) -> ("Expansion Input Array"=w1493:fxp<+/-,34,9>[])  [unwired: 2 out]
    n409 = shared-variable "RT CompactRIO Target 2\\Library 1.lvlib\\Control Variables"(error in=w1504) -> (w1559:dbl[])  [unwired: 1 out]
    "Control Variables" <- w1559
    n410 = shared-variable "RT CompactRIO Target 2\\Library 1.lvlib\\Inject_Arrays"(error in=w1504) -> (w1520:dbl[])  [unwired: 1 out]
    n411 = xnode "Read/Write Control"("FPGA VI Reference In"=w1519, "error in"=w1504) -> ("Array 2 In"=w1486:fxp<+/-,30,9>[])  [unwired: 2 out]
    n412 = xnode "Read/Write Control"("FPGA VI Reference In"=w1462, "error in"=w1504) -> ("MFC Error No."=w1495:u8)  [unwired: 2 out]
    n413 = Delete From Array(array=w1486, length=2, index=0) -> (array with subset deleted=w1483:fxp<+/-,30,9>[])  [unwired: 1 out]
    n414 = Unbundle By Name(w1571) -> ("UEGO1Lambda"=w1488:sgl, "UEGO2Lambda"=w1451:sgl)
    n415 = Unbundle By Name(w1452) -> ("UEGO1Lambda"=w1450:sgl, "UEGO2Lambda"=w1449:sgl)
    n416 = shared-variable "RT CompactRIO Target 2\\Library 1.lvlib\\Inject_Arrays_Lambda"(error in=w1504) -> (w1522:dbl[])  [unwired: 1 out]
    n417 = shared-variable "RT CompactRIO Target 2\\Library 1.lvlib\\Inject_Arrays"(error in=w1504) -> (w1508:dbl[])  [unwired: 1 out]
    n418 = Number To Boolean Array(number=w1495) -> (Boolean array=w1494:bool[])
    n419 = local read "UEGO Meas 2"() -> (w1489:T2)
    n420 = xnode "Read/Write Control"("FPGA VI Reference In"=w1462, "error in"=w1504) -> ("Array 1 In"=w1532:fxp<+/-,35,9>[])  [unwired: 2 out]
    n421 = Index Array(array=w1494) -> (element #1=→"CO":bool, element #2=→"HC-1":bool, element #3=→"AIR-1":bool, element #4=→"NO":bool, element #5=→"AIR-B":bool, element #6=→"HC-B":bool, element #7=→"AIR-2":bool, element #8=→"HC-2":bool)  [unwired: 8 in]
    n422 = xnode "Read/Write Control"("FPGA VI Reference In"=w1514, "error in"=w1504) -> ("NOxSensorData 1"=w1598:T19, "NOxSensorData 2"=w1597:T19)  [unwired: 2 out]
    n423 = Index Array(array=w1493, index #1=0 ("index"), index #2=1 ("index")) -> (element #1=w1553:fxp<+/-,34,9>, element #2=w1556:fxp<+/-,34,9>)
    n424 = Delete From Array(array=w1483, length=14, index=136) -> (deleted portion=w1474:fxp<+/-,30,9>[])  [unwired: 1 out]
    n425 = local read "STOP"() -> (w1611:bool)
    n426 = call "MFC Parse.vi"("MFC Raw"=w1483) -> ("Array"=w1560:dbl[])
    n427 = call "5pt Mov Avg.vi"("Value in"=w1488) -> ("Value out"=w1448:dbl)  [unwired: 10 in]
    "UEGO 1 Cat" <- w1448
    n428 = call "5pt Mov Avg.vi"("Value in"=w1451) -> ("Value out"=w1447:dbl)  [unwired: 10 in]
    n429 = call "5pt Mov Avg.vi"("Value in"=w1450) -> ("Value out"=w1446:dbl)  [unwired: 10 in]
    n430 = call "5pt Mov Avg.vi"("Value in"=w1449) -> ("Value out"=w1445:dbl)  [unwired: 10 in]
    n431 = Unbundle By Name(w1489) -> ("UEGO1Lambda"=w1487:sgl)  [unwired: 1 out]
    "UEGO 1 Fur" <- w1487
    n432 = Delete From Array(array=w1532, length=2, index=0) -> (deleted portion=w1529:fxp<+/-,35,9>[])  [unwired: 1 out]
    n433 = call "Valve_Read.vi"("In Array"=w1474) -> ("x/y 2"=→"Valve 2 Position":dbl, "x/y"=→"Valve 1 Position":dbl)  [unwired: 9 in]
    n434 = Index Array(array=w1529, index #1=0 ("index"), index #2=1 ("index")) -> (element #1=w1528:fxp<+/-,35,9>, element #2=w1525:fxp<+/-,35,9>)
    n435 = call "5pt Mov Avg.vi"("Value in"=w1553) -> ("Value out"=w1552:dbl)  [unwired: 10 in]
    n436 = call "5pt Mov Avg.vi"("Value in"=w1556) -> ("Value out"=w1551:dbl)  [unwired: 10 in]
    n437 = call "NOx MAX.vi"("NOx Input 2"=w1597, "NOx Input 1"=w1598) -> ("Lambda 2"=w1541:dbl, "Lambda 1"=w1542:dbl)  [unwired: 3 in, 5 out]
    n438 = Build Array(w1448, w1447, w1446, w1445) -> (→"UEGO Array":dbl[])
    n439 = call "5pt Mov Avg.vi"("Value in"=w1552) -> ("Value out"=w1454:dbl)  [unwired: 10 in]
    "Flow 1" <- w1454
    n440 = call "5pt Mov Avg.vi"("Value in"=w1551) -> ("Value out"=w1453:dbl)  [unwired: 10 in]
    "Flow 2" <- w1453
    n441 = Index Array(array=w1559, index #1=28 ("index"), index #2=24 ("index"), index #3=25 ("index"), index #4=26 ("index"), index #5=18 ("index"), index #6=19 ("index"), index #7=20 ("index"), index #8=29 ("index"), index #9=30 ("index"), index #10=2 ("index"), index #11=6 ("index"), index #12=7 ("index")) -> (element #1=w1603:dbl, element #2=w1604:dbl, element #3=w1605:dbl, element #4=w1606:dbl, element #5=w1570:dbl, element #6=w1568:dbl, element #7=w1565:dbl, element #8=w1563:dbl, element #9=w1561:dbl, element #10=w1441:dbl, element #11=w1438:dbl, element #12=w1436:dbl)
    n442 = call "ECM_Lambda_Propane.vi"("V In"=w1528) -> ("Lambda Corr"=w1444:dbl)  [unwired: 6 in, 2 out]
    "ECM 1" <- w1444
    n443 = call "ECM_Lambda_Propane.vi"("V In"=w1525) -> ("Lambda Corr"=w1443:dbl)  [unwired: 6 in, 2 out]
    "ECM 2" <- w1443
    n444 = Bundle By Name(cluster=cluster{"output high":dbl, "output low":dbl} {"output high"=100.0, "output low"=-100.0} ("output range"), "output high"="Output High 2", "output low"="Output Low 2") -> (w1533:cluster{"output high":dbl, "output low":dbl})
    n445 = Bundle By Name(cluster=cluster{"output high":dbl, "output low":dbl} {"output high"=100.0, "output low"=-100.0} ("output range"), "output high"="Output High 1", "output low"="Output Low 1") -> (w1572:cluster{"output high":dbl, "output low":dbl})
    n446 = Bundle By Name(cluster=cluster{"output high":dbl, "output low":dbl} {"output high"=100.0, "output low"=-100.0} ("output range"), "output high"="Output High 3", "output low"="Output Low 3") -> (w1509:cluster{"output high":dbl, "output low":dbl})
    n447 = Build Array(w1454, w1453) -> (w1455:dbl[])
    n448 = local read "Test Start"() -> (w1490:i32)
    n449 = call "System_Inj_Array_Split.vi"("Inject_Arrays"=w1508) -> ("Lambda"=w1475:dbl[], "Closed Loop"=w1476:dbl[], "Cut Off -2"=w1477:dbl[], "Cut Off -1"=w1478:dbl[])  [unwired: 4 in, 3 out]
    n450 = call "Inj_Array_Split.vi"("Inject_Arrays"=w1520) -> ("Air Cyc 1"=w1544:dbl[], "HC Bal"=w1545:dbl[], "HC Cyc 2"=w1546:dbl[], "HC Cyc 1"=w1547:dbl[], "Air Cyc 2"=w1543:dbl[], "NO"=w1548:dbl[], "Air Bal"=w1550:dbl[], "CO"=w1549:dbl[], "Cycle Length"=w1521:i32)  [unwired: 2 in]
    "Cycle Length" <- w1521
    n451 = Decrement(x=w1521) -> (x-1=w1537:i32)
    n452 = case shown="3" w1490 {
      tunnel: [w1615 w1628 "Air Cyc 1" w1747] -> w1610
      tunnel: [w1615 w1628 "NO" w1746] -> w1609
      tunnel: [w1615 w1628 "Air Bal" w1745] -> w1540
      tunnel: [w1615 w1628 "HC Cyc 1" w1744] -> w1539
      tunnel: [w1615 w1628 "HC Bal" w1743] -> w1608
      tunnel: 0.0 ("y") -> [_ _ _ w1742]
      tunnel: w1606 -> [_ _ _ w1741]
      tunnel: w1605 -> [_ _ _ w1740]
      tunnel: w1604 -> [_ _ _ w1739]
      tunnel: w1603 -> [_ _ _ w1738]
      tunnel: w1448 -> [_ _ _ w1737]
      tunnel: w1542 -> [_ _ _ w1736]
      tunnel: w1541 -> [_ _ _ w1735]
      tunnel: 4 -> [_ _ _ w1734]
      tunnel: w1595 -> [w1623 _ _ w1733]
      tunnel: [w1623 w1629 w1658 w1732] -> w1594
      tunnel: w1593 -> [w1622 w1638 _ w1731]
      tunnel: [w1622 w1638 0 w1730] -> w1592
      tunnel: w1591 -> [w1621 w1637 _ w1729]
      tunnel: [w1621 w1637 3 w1728] -> w1590
      tunnel: w1589 -> [w1620 w1636 _ w1727]
      tunnel: [w1620 w1636 1 w1726] -> w1588
      tunnel: w1587 -> [w1619 w1635 _ w1725]
      tunnel: [w1619 w1635 1 w1724] -> w1586
      tunnel: w1585 -> [w1618 w1634 _ w1723]
      tunnel: [w1618 w1634 1 w1722] -> w1584
      tunnel: w1583 -> [w1617 w1633 _ w1721]
      tunnel: w1582 -> [w1616 w1632 _ w1720]
      tunnel: [w1617 w1633 1 w1719] -> w1581
      tunnel: [w1616 w1632 0 w1718] -> w1580
      tunnel: w1579 -> [w1624 _ _ w1717]
      tunnel: [w1624 w1629 w1658 w1716] -> w1578
      tunnel: w1577 -> [w1625 w1630 _ w1715]
      tunnel: [w1625 w1630 0 ("t") w1714] -> w1576
      tunnel: w1549 -> [_ _ _ w1713]
      tunnel: w1548 -> [_ _ _ w1712]
      tunnel: w1547 -> [_ _ _ w1711]
      tunnel: w1546 -> [_ _ _ w1710]
      tunnel: w1572 -> [_ _ _ w1709]
      tunnel: w1519 -> [_ _ _ w1708]
      tunnel: w1570 -> [_ _ _ w1707]
      tunnel: w1568 -> [_ _ _ w1706]
      tunnel: w1565 -> [_ _ _ w1705]
      tunnel: w1563 -> [_ _ _ w1704]
      tunnel: w1561 -> [_ _ _ w1703]
      tunnel: w1560 -> [_ _ _ w1702]
      tunnel: w1550 -> [_ _ _ w1701]
      tunnel: w1555 -> [_ w1631 _ w1700]
      tunnel: [_ w1631 i32[] [0, 0, 3, 1, 1, 1, 1, 0] _] -> w1554
      tunnel: w1537 -> [_ _ _ w1699]
      tunnel: w1447 -> [_ _ _ w1698]
      tunnel: w1545 -> [_ _ _ w1697]
      tunnel: [w1615 w1628 "Air Cyc 2" w1696] -> w1538
      tunnel: w1544 -> [_ _ _ w1695]
      tunnel: w1543 -> [_ _ _ w1694]
      tunnel: "PID Catalyst 1" -> [_ _ _ w1693]
      tunnel: [_ _ _ w1692] -> w1524
      tunnel: w1533 -> [_ _ _ w1691]
      tunnel: "PID Catalyst 2" -> [_ _ _ w1690]
      tunnel: w1444 -> [_ _ _ w1689]
      tunnel: w1443 -> [_ _ _ w1688]
      tunnel: [_ _ _ w1680] -> w1523
      tunnel: w1522 -> [_ _ _ w1687]
      tunnel: w1521 -> [_ _ _ w1686]
      tunnel: [w1615 w1628 "HC Cyc 2" w1685] -> w1518
      tunnel: [w1615 w1628 "CO" w1684] -> w1517
      tunnel: "PID Mop-up Catalyst" -> [_ _ _ w1683]
      tunnel: w1509 -> [_ _ _ w1682]
      tunnel: w1462 -> [_ _ _ w1681]
      tunnel: w1487 -> [_ _ _ w1679]
      tunnel: w1478 -> [_ _ _ w1678]
      tunnel: w1477 -> [_ _ _ w1677]
      tunnel: w1476 -> [_ _ _ w1676]
      tunnel: w1475 -> [_ _ _ w1675]
      tunnel: "Valve 1 SP" -> [w1614 w1627 w1640 w1674]
      tunnel: "Valve 2 SP" -> [w1613 w1626 w1639 w1672]
      tunnel: [w1614 w1627 w1640 w1673] -> w1464
      tunnel: [w1613 w1626 w1639 w1671] -> w1463
      tunnel: w1461 -> [_ _ _ w1670]
      tunnel: [_ _ _ w1669] -> w1460
      tunnel: w1459 -> [_ _ _ w1668]
      tunnel: [_ _ _ w1667] -> w1458
      tunnel: [_ _ _ w1666] -> w1457
      tunnel: w1456 -> [_ _ _ w1665]
      tunnel: w1446 -> [_ _ _ w1664]
      tunnel: w1445 -> [_ _ _ w1663]
      tunnel: w1441 -> [_ _ _ w1662]
      tunnel: w1438 -> [_ _ _ w1661]
      tunnel: w1436 -> [_ _ _ w1660]
      tunnel: "NO PID Light-Off" -> [_ _ _ w1659]
      frame 0, Default {
        w1615 = 0.0 ("Numeric")
      }
      frame 1 {
        w1629 = string[] [] ("Ageing Variables")
        w1628 = 0.0 ("Numeric")
      }
      frame 2 {
        # "Index2"
        # "Index1"
        # "Clock"
        # "Count.steps"
        # "Count.repeats"
        # "Count.subcycles"
        # "Count.cycles"
        n453 = shared-variable "RT CompactRIO Target 2\\Library 1.lvlib\\Ageing Variables"() -> (w1658:string[])  [unwired: 1 in, 1 out]
      }
      frame 3 {
        n454 = case shown="2" w1734 {
          tunnel: [w1753 w1772 w1794 w1797 w1878 w1941 w1955 w2346] -> w1747
          tunnel: [w1763 w1779 w1781 w1797 w1850 w1941 w1954 w2346] -> w1746
          tunnel: [w1763 w1779 w1794 w1797 w1824 w1941 w2027 w2346] -> w1745
          tunnel: [w1763 w1764 w1794 w1797 0.0 ("Numeric") w1941 w1956 w2346] -> w1744
          tunnel: w1738 -> [_ _ _ _ _ _ w2022 w2419]
          tunnel: w1741 -> [_ _ _ _ _ _ w2024 w2414]
          tunnel: w1740 -> [_ _ _ _ _ _ w2025 w2415]
          tunnel: w1739 -> [_ _ _ _ _ _ w2026 w2416]
          tunnel: w1737 -> [_ _ _ _ w1815 _ w1947 w2420]
          tunnel: [w1763 w1779 w1794 w1797 w1802 w1941 w1942 w2346] -> w1743
          tunnel: w1742 -> [_ _ _ _ _ _ _ _]
          tunnel: w1736 -> [_ _ _ _ w1870 _ _ _]
          tunnel: w1735 -> [_ _ _ _ w1875 _ _ _]
          tunnel: w1733 -> [_ _ _ _ _ _ w2007 w2372]
          tunnel: [_ _ _ _ _ _ w2007 w2372] -> w1732
          tunnel: w1731 -> [_ _ _ _ _ _ w1963 w2379]
          tunnel: [_ _ _ _ _ _ w2020 w2371] -> w1730
          tunnel: w1729 -> [_ _ _ _ _ _ w1975 w2378]
          tunnel: [_ _ _ _ _ _ w2019 w2370] -> w1728
          tunnel: w1727 -> [_ _ _ _ _ _ w2018 w2377]
          tunnel: [_ _ _ _ _ _ w2017 w2369] -> w1726
          tunnel: w1725 -> [_ _ _ _ _ _ w2016 w2376]
          tunnel: [_ _ _ _ _ _ w2015 w2368] -> w1724
          tunnel: w1723 -> [_ _ _ _ _ _ w2014 w2375]
          tunnel: [_ _ _ _ _ _ w2013 w2367] -> w1722
          tunnel: w1721 -> [_ _ _ _ _ _ w2012 w2374]
          tunnel: w1720 -> [_ _ _ _ _ _ w1969 w2373]
          tunnel: [_ _ _ _ _ _ w2011 w2366] -> w1719
          tunnel: [_ _ _ _ _ _ w2010 w2365] -> w1718
          tunnel: w1717 -> [_ _ _ _ _ _ w1996 w2380]
          tunnel: [_ _ _ _ _ _ w1978 w2349] -> w1716
          tunnel: w1715 -> [_ _ _ _ w1827 _ _ _]
          tunnel: [_ _ _ _ w1891 _ _ _] -> w1714
          tunnel: w1713 -> [_ _ _ _ w1844 _ _ _]
          tunnel: w1712 -> [_ _ _ _ w1843 _ _ _]
          tunnel: w1711 -> [_ _ _ _ w1842 _ _ _]
          tunnel: w1710 -> [_ _ _ _ w1841 _ _ _]
          tunnel: w1709 -> [_ _ _ _ w1890 _ w1953 w2347]
          tunnel: w1708 -> [_ _ _ _ _ _ w1948 _]
          tunnel: w1702 -> [_ _ _ _ _ _ _ _]
          tunnel: w1707 -> [_ _ _ _ _ _ _ _]
          tunnel: w1706 -> [_ _ _ _ _ _ w1946 _]
          tunnel: w1705 -> [_ _ _ _ _ _ w1945 _]
          tunnel: w1704 -> [_ _ _ _ _ _ w1944 _]
          tunnel: w1703 -> [_ _ _ _ _ _ _ _]
          tunnel: w1701 -> [_ _ _ _ w1837 _ _ _]
          tunnel: w1700 -> [_ _ _ _ _ _ _ _]
          tunnel: w1699 -> [_ _ _ _ w1864 _ _ _]
          tunnel: w1698 -> [_ _ _ _ w1814 _ _ _]
          tunnel: w1697 -> [_ _ _ _ w1840 _ _ _]
          tunnel: [w1763 w1779 w1794 w1797 w1825 w1941 _ w2346] -> w1696
          tunnel: w1695 -> [_ _ _ _ w1839 _ _ _]
          tunnel: w1694 -> [_ _ _ _ w1838 _ _ _]
          tunnel: w1693 -> [_ _ _ _ w1877 _ _ _]
          tunnel: [_ _ _ _ w1876 _ _ _] -> w1692
          tunnel: w1691 -> [_ _ _ _ w1848 _ _ _]
          tunnel: w1690 -> [_ _ _ _ w1847 _ _ _]
          tunnel: w1689 -> [_ _ _ _ w1869 _ _ _]
          tunnel: w1688 -> [_ _ _ _ w1874 _ _ _]
          tunnel: w1687 -> [_ _ _ _ _ _ _ _]
          tunnel: w1686 -> [_ _ _ _ w1809 _ _ _]
          tunnel: [w1763 w1779 w1794 w1797 w1823 w1941 w1942 w2346] -> w1685
          tunnel: [w1759 w1779 w1780 w1797 w1857 w1941 0.0 ("Numeric") w2346] -> w1684
          tunnel: w1683 -> [_ _ _ _ w1860 _ _ _]
          tunnel: w1682 -> [_ _ _ _ w1861 _ _ _]
          tunnel: w1681 -> [_ _ _ _ w1846 _ _ _]
          tunnel: [_ _ _ _ w1834 _ _ _] -> w1680
          tunnel: w1679 -> [_ _ _ _ w1819 _ _ _]
          tunnel: w1678 -> [_ _ _ _ w1831 _ _ _]
          tunnel: w1677 -> [_ _ _ _ w1830 _ _ _]
          tunnel: w1676 -> [_ _ _ _ w1826 _ _ _]
          tunnel: w1675 -> [_ _ _ _ w1829 _ _ _]
          tunnel: w1674 -> [_ _ _ w1796 w1822 _ _ _]
          tunnel: [_ _ _ w1796 w1822 _ _ _] -> w1673
          tunnel: [_ _ _ w1795 w1821 _ _ _] -> w1671
          tunnel: w1672 -> [_ _ _ w1795 w1821 _ _ _]
          tunnel: w1670 -> [_ _ _ _ w1817 _ _ _]
          tunnel: [_ _ _ _ w1816 _ _ _] -> w1669
          tunnel: w1668 -> [_ _ _ _ w1808 _ _ _]
          tunnel: [_ _ _ _ w1807 _ _ _] -> w1667
          tunnel: [_ _ _ _ w1806 _ _ _] -> w1666
          tunnel: w1665 -> [_ _ _ _ w1805 _ _ _]
          tunnel: w1664 -> [_ _ _ _ w1800 _ _ _]
          tunnel: w1663 -> [_ _ _ _ w1799 _ _ _]
          tunnel: w1662 -> [w1752 w1777 w1786 _ _ _ _ _]
          tunnel: w1661 -> [w1750 w1770 _ _ _ _ _ _]
          tunnel: w1660 -> [w1748 w1769 _ _ _ _ _ _]
          tunnel: w1659 -> [_ _ w1784 _ _ _ _ _]
          frame 0, Default {
            w1763 = 0.0 ("Numeric")
            # "Rapidox  Input from Rapidox \nLook at replacing from MEXA 7170 or MEXA 1"
            # "Flow Rate input from Shared\nVariables Index 2"
            # "O2 eq up input from NOx can Array"
            # "Lambda targetinput from Shared\nVariables Index 6"
            # "O2 (O2 t) conc input from Shared\nVariables Index 7"
            # "O2 conc input from Shared\nVariables Index 7"
            # "Flow Rate input from Shared\nVariables Index 2"
            # "5Hz CO Loop"
            n455 = Multiply(x=w1752, y=50.0) -> (x*y=w1749:dbl)
            n456 = call "Air MFR loff.vi"("O2t %"=w1748, "Flow rate"=w1749) -> ("Air MFR"=w1754:dbl)  [unwired: 9 in]
            n457 = call "CO MFR loff.vi"("Flow rate"=w1749, "O2t %"=w1748, "Lambda_t"=w1750) -> ("CO MFR"=w1758:dbl)  [unwired: 8 in]
            n458 = Multiply(x=w1754, y="O2 Fact COLO") -> (x*y=w1756:dbl)
            n459 = Multiply(x=w1758, y="CO Fact COLO") -> (x*y=w1761:dbl)
            n460 = Add(x="O2 Base COLO", y=w1756) -> (x+y=w1753:dbl)
            n461 = Add(x="CO Base COLO", y=w1761) -> (x+y=w1759:dbl)
          }
          frame 1 {
            w1779 = 0.0 ("Numeric")
            # "5Hz HC Loop"
            n462 = Multiply(x=w1777, y=50.0) -> (x*y=w1771:dbl)
            n463 = call "Air MFR loff.vi"("O2t %"=w1770, "Flow rate"=w1771) -> ("Air MFR"=w1773:dbl)  [unwired: 9 in]
            n464 = call "HC MFR loff.vi"("Flow rate"=w1771, "O2t %"=w1769, "Lambda_t"=w1770) -> ("HC MFR"=w1765:dbl)  [unwired: 8 in]
            n465 = Multiply(x=w1773, y="O2 Fact HCLO") -> (x*y=w1775:dbl)
            n466 = Add(x="O2 Base HCLO", y=w1775) -> (x+y=w1772:dbl)
            n467 = Multiply(x=w1765, y="HC Fact HCLO") -> (x*y=w1767:dbl)
            n468 = Add(x="HC Base HCLO", y=w1767) -> (x+y=w1764:dbl)
          }
          frame 2 {
            w1794 = 0.0 ("Numeric")
            # "5Hz NO Loop"
            n469 = Multiply(x=w1786, y=50.0) -> (x*y=w1785:dbl)
            n470 = call "NOSO2 calc age.vi"("PID"=w1784, "Flow Rate"=w1785) -> ("NO/SO2 MFR"=w1783:dbl)  [unwired: 9 in]
            n471 = Multiply(x=w1783, y="NO Factor NOLO") -> (x*y=w1789:dbl)
            n472 = call "CO calc loff.vi"("NOx MFR"=w1783) -> ("CO MFR"=w1782:dbl)  [unwired: 10 in]
            n473 = Add(x=w1789, y="NO Base NOLO") -> (x+y=w1781:dbl)
            n474 = Multiply(x=w1782, y="CO Factor NOLO") -> (x*y=w1792:dbl)
            n475 = Add(x="CO Base NOLO", y=w1792) -> (x+y=w1780:dbl)
          }
          frame 3 {
            w1797 = 0.0 ("Numeric")
            # "5Hz Sweep Loop"
          }
          frame 4 {
            w1820 = FALSE ("CUToff 1")
            # "Control Selection"
            # "Flow Shut-off Valve"
            # "5Hz Ageing Loop"
            # "NO"
            # "Open/Closed Loop"
            # "CO"
            # "Air Bal"
            # "Air 2"
            # "Air 1"
            # "HC Bal"
            # "HC 2"
            # "MFC's\n\nHC\nAir_1\nAir_B\nHC_B\nAir_2"
            # "Ageing Array\n0.Time\n1.Bed temp\n2.Inlet lambda\n3.O2\n4.HC\n5.CO\n6.Bleed\n7.Inlet temp\n8.Flow rate\n9.NOx\n10.CUToff"
            # "HC 1 Cyc"
            n476 = case shown="False" "NOxLambda Control" {
              tunnel: w1870 -> [_ w1924]
              tunnel: [w1910 w1924] -> w1872
              tunnel: w1875 -> [_ w1923]
              tunnel: [w1908 w1923] -> w1873
              tunnel: w1815 -> [w1913 _]
              tunnel: w1814 -> [w1914 _]
              tunnel: w1800 -> [w1909 _]
              tunnel: w1799 -> [w1911 _]
              tunnel: 0 ("length") -> [w1912 _]
              frame False {
                n477 = case shown="0, Default" w1912 {
                  tunnel: w1913 -> [w1916 w1918 _ _]
                  tunnel: w1914 -> [_ _ w1920 w1922]
                  tunnel: w1911 -> [_ w1917 _ w1921]
                  tunnel: [w1916 w1918 w1920 w1922] -> w1910
                  tunnel: w1909 -> [w1915 _ w1919 _]
                  tunnel: [w1915 w1917 w1919 w1921] -> w1908
                  frame 0, Default {
                  }
                  frame 1 {
                  }
                  frame 2 {
                  }
                  frame 3 {
                  }
                }
              }
              frame True {
              }
            }
            n478 = case shown="False" "ECM Lambda Control" {
              tunnel: w1869 -> [_ w1907]
              tunnel: [w1903 w1906] -> w1813
              tunnel: w1874 -> [_ w1905]
              tunnel: [w1902 w1904] -> w1812
              tunnel: w1872 -> [w1903 _]
              tunnel: w1873 -> [w1902 _]
              frame False {
              }
              frame True {
                n479 = call "3pt Mov Avg.vi"("Value in"=w1907) -> ("Value out"=w1906:dbl)  [unwired: 10 in]
                n480 = call "3pt Mov Avg.vi"("Value in"=w1905) -> ("Value out"=w1904:dbl)  [unwired: 10 in]
              }
            }
            n481 = Equal?(x=w1864, y=w1827) -> (x = y?=w1889:bool)
            n482 = Index Array(array=w1844, index=w1827) -> (element=w1845:dbl)
            n483 = Index Array(array=w1843, index=w1827) -> (element=w1849:dbl)
            n484 = Index Array(array=w1842, index=w1827) -> (element=w1856:dbl)
            n485 = Index Array(array=w1841, index=w1827) -> (element=w1855:dbl)
            n486 = Index Array(array=w1840, index=w1827) -> (element=w1851:dbl)
            n487 = Index Array(array=w1839, index=w1827) -> (element=w1852:dbl)
            n488 = Index Array(array=w1838, index=w1827) -> (element=w1833:dbl)
            n489 = Index Array(array=w1837, index=w1827) -> (element=w1853:dbl)
            n490 = Increment(x=w1827) -> (x+1=w1893:i32)
            n491 = Index Array(array=w1829, index=w1827) -> (element=w1835:dbl)
            n492 = Index Array(array=dbl[] [], index=w1827) -> (element=w1836:dbl)
            n493 = Select(t=0, s=w1889, f=w1893) -> (s? t:f=w1891:i32)
            n494 = call "Mov_Avg_JS_Dual.vi"("Cycle Length"=w1809, "Array In 2"=w1805, "Input 2"=w1812, "Array In"=w1808, "Input"=w1813) -> ("Array Out Main 2"=w1806:dbl[], "Mean 2"=w1810:dbl, "Array Out Main"=w1807:dbl[], "Mean"=w1811:dbl)  [unwired: 3 in]
            n495 = call "Mov_Avg_JS.vi"("Array In"=w1817, "Cycle Length"=w1809, "Input"=w1819) -> ("Array Out Main"=w1816:dbl[], "Mean"=w1818:dbl)  [unwired: 7 in]
            n496 = Multiply(x=w1845, y="CO Factor") -> (x*y=w1857:dbl)
            n497 = Multiply(x=w1849, y="NO Factor") -> (x*y=w1850:dbl)
            n498 = Multiply(x=w1856, y="HC Cyc1 Factor") -> (x*y=w1804:dbl)
            n499 = Multiply(x=w1855, y="HC Cyc 2 Factor") -> (x*y=w1823:dbl)
            n500 = Multiply(x=w1851, y="HC Bal Factor") -> (x*y=w1803:dbl)
            n501 = Index Array(array=w1831, index=w1827) -> (element=w1834:dbl)
            n502 = Index Array(array=w1830, index=w1827) -> (element=w1832:dbl)
            n503 = Index Array(array=w1826, index=w1827) -> ()  [unwired: 1 out]
            n504 = Add(x="Lambda SP", y=w1835) -> (x+y=w1867:dbl)
            n505 = Add(x=w1835, y="Lambda SP 2") -> (x+y=w1868:dbl)
            n506 = Equal To 0?(x=w1836) -> (x = 0?=w1888:bool)
            n507 = case shown="True" w1888 {
              tunnel: w1877 -> [_ w1929]
              tunnel: w1890 -> [_ w1930]
              tunnel: w1867 -> [_ w1940]
              tunnel: w1811 -> [_ w1939]
              tunnel: w1833 -> [w1926 w1934]
              tunnel: [w1926 w1933] -> w1880
              tunnel: w1852 -> [w1925 w1937]
              tunnel: [w1925 w1936] -> w1882
              tunnel: w1810 -> [_ w1932]
              tunnel: w1868 -> [_ w1931]
              tunnel: w1847 -> [_ w1928]
              tunnel: w1848 -> [_ w1927]
              frame False {
                # "open loop - not B"
              }
              frame True {
                # "Baseline B"
                n508 = call-poly <vilib>:"PID.vi"("output range"=w1930, "PID gains"=w1929, "process variable"=w1939, "setpoint"=w1940) -> ("output"=w1938:dbl)  [unwired: 6 in, 1 out]
                n509 = call-poly <vilib>:"PID.vi"("output range"=w1927, "PID gains"=w1928, "process variable"=w1932, "setpoint"=w1931) -> ("output"=w1935:dbl)  [unwired: 6 in, 1 out]
                n510 = Add(x=w1937, y=w1938) -> (x+y=w1936:dbl)
                n511 = Add(x=w1934, y=w1935) -> (x+y=w1933:dbl)
              }
            }
            n512 = case shown="True" "Mop-up Lambda Control" {
              tunnel: w1860 -> [_ w1899]
              tunnel: w1861 -> [_ w1901]
              tunnel: "Lambda SP 3" -> [_ w1900]
              tunnel: w1818 -> [_ w1898]
              tunnel: w1853 -> [w1894 w1896]
              tunnel: [w1894 w1895] -> w1859
              frame False {
              }
              frame True {
                # "Baseline B"
                n513 = call-poly <vilib>:"PID.vi"("output range"=w1901, "PID gains"=w1899, "process variable"=w1898, "setpoint"=w1900) -> ("output"=w1897:dbl)  [unwired: 6 in, 1 out]
                n514 = Add(x=w1896, y=w1897) -> (x+y=w1895:dbl)
              }
            }
            n515 = Not Equal To 0?(x=w1834) -> ()  [unwired: 1 out]
            n516 = Not Equal To 0?(x=w1832) -> ()  [unwired: 1 out]
            n517 = xnode "Read/Write Control"("FPGA VI Reference In"=w1846, "CUToff 1"=w1820, "CUToff 2"=w1820) -> ()  [unwired: 1 in, 2 out]
            n518 = Add(x=w1804, y=w1803) -> (x+y=w1802:dbl)
            n519 = Boolean To (0,1)(Boolean=w1820) -> (0, 1=w1876:i16)
            n520 = Multiply(x=w1882, y="Air Cyc 1 Factor") -> (x*y=w1878:dbl)
            n521 = Multiply(x=w1880, y="Air Cyc 2 Factor") -> (x*y=w1825:dbl)
            n522 = Multiply(x=w1859, y="Air Bal Factor") -> (x*y=w1824:dbl)
          }
          frame 5 {
            (unwired) 50.0 ("Numeric")
            w1941 = 0.0 ("Numeric")
            # "Leak Test"
          }
          frame 6 {
            w1942 = 0.0 ("Numeric")
            # "Ageing Original"
            # "Ageing Array\n0.Time\n1.Bed temp\n2.Inlet lambda\n3.O2\n4.HC\n5.CO\n6.Bleed\n7.Inlet temp\n8.Flow rate\n9.NOx\n10.CUToff"
            # "repeats"
            # "no. steps"
            # "ageing gas"
            # "no. subcycles"
            # "no. cycles"
            # "28 Furnace Lambda SP\n24 Lambda P\n25 Lambda I\n26 Lambda D\n19 CO Bottle Conc\n20 HC Bottle Conc\n29 HC React Const\n30 Full System\n\n\nPossible additions\nSwitch Between Routines"
            # "Lambda input Furnace (measured)"
            # "Target Furnace Lambda (should we replace? incase of varying lambda profiles)"
            # "AIR\n Cyc\nl\ne"
            # "HC\n Cyc\nl\ne"
            # "Air Balance"
            # "HC Balance"
            # "Lambda UEGO"
            # "Target O2%"
            # "HC conc %"
            # "HC reaction ct"
            # "Flow rate l/min"
            n523 = Add(x=w1963, y=w1975) -> (x+y=w1974:i32)
            n524 = Bundle By Name(cluster=T10 {"proportional gain (Kc)"=1.0, "integral time (Ti, min)"=0.1, "derivative time (Td, min)"=0.0} ("Air PID Gains CO 2"), "proportional gain (Kc)"=w2026, "integral time (Ti, min)"=w2025, "derivative time (Td, min)"=w2024) -> (w2023:T10)
            n525 = Increment(x=w1963) -> (x+1=w1962:i32)
            n526 = Delete From Array(array=w2007, length=3, index=0) -> (deleted portion=w2003:string[], array with subset deleted=w1979:string[])
            n527 = Increment(x=w1962) -> (x+1=w1961:i32)
            n528 = Index Array(array=w1979, index #1=w1963, index #2=w1962, index #3=w1961) -> (element #1=w1993:string, element #2=w1994:string, element #3=w1995:string)
            n529 = Index Array(array=w2003, index #1=0 ("index"), index #2=1 ("index"), index #3=2 ("index")) -> (element #1=w2001:string, element #2=w2002:string, element #3=w2000:string)
            n530 = Decimal String To Number(string=w1993) -> (number=w1964:i32)  [unwired: 2 in, 1 out]
            n531 = Decimal String To Number(string=w1994) -> (number=w1965:i32)  [unwired: 2 in, 1 out]
            n532 = Decimal String To Number(string=w1995) -> (number=w1966:i32)  [unwired: 2 in, 1 out]
            n533 = Decimal String To Number(string=w2001) -> (number=w1977:i32)  [unwired: 2 in, 1 out]
            n534 = Decimal String To Number(string=w2002) -> (number=w1992:i32)  [unwired: 2 in, 1 out]
            n535 = Decimal String To Number(string=w2000) -> (number=w1967:i32)  [unwired: 2 in, 1 out]
            n536 = Array Subset(array=w1979, index=w1974, length=12) -> (w1972:string[])
            n537 = Index Array(array=w1972, index=0) -> (element=w1973:string)
            n538 = Decimal String To Number(string=w1973) -> (number=w1968:i32)  [unwired: 2 in, 1 out]
            n539 = Equal?(x=w1968, y=w1969) -> (x = y?=w1970:bool)
            n540 = case shown="False" w1970 {
              tunnel: w1975 -> [w2047 w2148]
              tunnel: [w2054 w2147] -> w2019
              tunnel: w1969 -> [w2038 w2128]
              tunnel: [w2049 w2133] -> w2010
              tunnel: w2016 -> [w2043 w2142]
              tunnel: w2012 -> [w2041 w2129]
              tunnel: [w2040 w2132] -> w2011
              tunnel: w1965 -> [w2039 w2145]
              tunnel: w1963 -> [w2042 w2134]
              tunnel: w2014 -> [w2050 w2130]
              tunnel: [w2051 w2136] -> w2013
              tunnel: w1964 -> [w2044 w2143]
              tunnel: [w2052 w2137] -> w2015
              tunnel: w1967 -> [w2045 w2141]
              tunnel: w2018 -> [w2046 w2140]
              tunnel: w1992 -> [w2048 w2139]
              tunnel: [w2053 w2138] -> w2017
              tunnel: [w2055 w2135] -> w2020
              tunnel: [w2057 w2146] -> _
              tunnel: w1966 -> [w2035 w2131]
              tunnel: [w2037 w2126] -> w1978
              tunnel: w1996 -> [w2037 _]
              tunnel: w1972 -> [_ w2126]
              frame False {
                n541 = Decrement(x=w2035) -> (x-1=w2036:i32)
                n542 = Equal?(x=w2036, y=w2038) -> (x = y?=w2056:bool)
                n543 = case shown="True" w2056 {
                  tunnel: w2050 -> [w2059 w2070]
                  tunnel: w2044 -> [_ w2083]
                  tunnel: w2043 -> [w2058 w2081]
                  tunnel: w2045 -> [_ w2080]
                  tunnel: w2046 -> [w2063 w2079]
                  tunnel: w2048 -> [_ w2078]
                  tunnel: [FALSE w2077] -> w2057
                  tunnel: [w2063 w2073] -> w2053
                  tunnel: [w2058 w2071] -> w2052
                  tunnel: [w2059 w2069] -> w2051
                  tunnel: [w2065 w2076] -> w2055
                  tunnel: w2047 -> [w2064 w2075]
                  tunnel: [w2064 w2074] -> w2054
                  tunnel: w2042 -> [w2065 w2072]
                  tunnel: [w2061 0] -> w2049
                  tunnel: w2038 -> [w2062 _]
                  tunnel: w2041 -> [w2060 _]
                  tunnel: [w2060 1] -> w2040
                  tunnel: w2039 -> [_ _]
                  frame False {
                    n544 = Increment(x=w2062) -> (x+1=w2061:i32)
                  }
                  frame True {
                    n545 = Equal?(x=w2083, y=w2070) -> (x = y?=w2082:bool)
                    n546 = case shown="True" w2082 {
                      tunnel: w2081 -> [w2085 w2093]
                      tunnel: w2080 -> [_ w2103]
                      tunnel: w2079 -> [w2086 w2101]
                      tunnel: w2078 -> [_ w2100]
                      tunnel: [FALSE w2099] -> w2077
                      tunnel: [w2089 w2098] -> w2076
                      tunnel: w2075 -> [_ w2097]
                      tunnel: [3 w2096] -> w2074
                      tunnel: [w2086 w2095] -> w2073
                      tunnel: w2072 -> [w2089 w2094]
                      tunnel: [w2085 w2092] -> w2071
                      tunnel: w2070 -> [w2088 _]
                      tunnel: [w2087 1] -> w2069
                      frame False {
                        n547 = Increment(x=w2088) -> (x+1=w2087:i32)
                      }
                      frame True {
                        n548 = Equal?(x=w2103, y=w2093) -> (x = y?=w2102:bool)
                        n549 = case shown="True" w2102 {
                          tunnel: w2101 -> [w2108 w2116]
                          tunnel: w2100 -> [_ w2120]
                          tunnel: [FALSE w2118] -> w2099
                          tunnel: [w2107 0] -> w2098
                          tunnel: w2097 -> [w2105 _]
                          tunnel: [3 ("y") 3] -> w2096
                          tunnel: [w2108 w2117] -> w2095
                          tunnel: w2094 -> [w2104 _]
                          tunnel: w2093 -> [w2111 _]
                          tunnel: [w2110 1] -> w2092
                          frame False {
                            n550 = Increment(x=w2111) -> (x+1=w2110:i32)
                            n551 = Compound Arithmetic op=ADD(w2104, w2105, 12 ("y")) -> (w2107:i32)
                          }
                          frame True {
                            n552 = Equal?(x=w2120, y=w2116) -> (x = y?=w2119:bool)
                            n553 = case shown="True" w2119 {
                              tunnel: [FALSE TRUE] -> w2118
                              tunnel: [w2121 1] -> w2117
                              tunnel: w2116 -> [w2122 _]
                              frame False {
                                n554 = Increment(x=w2122) -> (x+1=w2121:i32)
                              }
                              frame True {
                              }
                            }
                          }
                        }
                      }
                    }
                  }
                }
              }
              frame True {
                n555 = Increment(x=w2128) -> (x+1=w2127:i32)
                n556 = Equal?(x=w2145, y=w2129) -> (x = y?=w2144:bool)
                n557 = case shown="False" w2144 {
                  tunnel: w2148 -> [w2150 w2166]
                  tunnel: [w2149 w2165] -> w2147
                  tunnel: [FALSE w2171] -> w2146
                  tunnel: w2131 -> [_ w2179]
                  tunnel: w2130 -> [w2152 w2177]
                  tunnel: w2143 -> [_ w2176]
                  tunnel: w2142 -> [w2155 w2175]
                  tunnel: w2141 -> [_ w2174]
                  tunnel: w2140 -> [w2156 w2173]
                  tunnel: w2139 -> [_ w2172]
                  tunnel: w2127 -> [w2158 w2160]
                  tunnel: [w2156 w2170] -> w2138
                  tunnel: [w2155 w2169] -> w2137
                  tunnel: [w2152 w2168] -> w2136
                  tunnel: [w2157 w2167] -> w2135
                  tunnel: w2134 -> [w2157 w2164]
                  tunnel: [w2158 w2163] -> w2133
                  tunnel: w2129 -> [w2154 w2161]
                  tunnel: [w2153 w2162] -> w2132
                  frame False {
                    n558 = Increment(x=w2154) -> (x+1=w2153:i32)
                    n559 = Add(x=w2150, y=12) -> (x+y=w2149:i32)
                  }
                  frame True {
                    n560 = Equal?(x=w2179, y=w2160) -> (x = y?=w2178:bool)
                    n561 = case shown="False" w2178 {
                      tunnel: w2177 -> [w2185 w2191]
                      tunnel: w2176 -> [_ w2204]
                      tunnel: w2175 -> [w2186 w2202]
                      tunnel: w2174 -> [_ w2201]
                      tunnel: w2173 -> [w2187 w2200]
                      tunnel: w2172 -> [_ w2199]
                      tunnel: [FALSE w2198] -> w2171
                      tunnel: [w2187 w2194] -> w2170
                      tunnel: [w2186 w2192] -> w2169
                      tunnel: [w2185 w2190] -> w2168
                      tunnel: [w2182 w2197] -> w2167
                      tunnel: w2166 -> [w2181 w2196]
                      tunnel: [w2181 w2195] -> w2165
                      tunnel: w2164 -> [w2182 w2193]
                      tunnel: [w2183 0] -> w2163
                      tunnel: w2160 -> [w2183 _]
                      tunnel: [w2180 w2188] -> w2162
                      tunnel: w2161 -> [w2180 w2188]
                      frame False {
                      }
                      frame True {
                        n562 = Equal?(x=w2204, y=w2191) -> (x = y?=w2203:bool)
                        n563 = case shown="False" w2203 {
                          tunnel: w2202 -> [w2206 w2214]
                          tunnel: w2201 -> [_ w2224]
                          tunnel: w2200 -> [w2207 w2222]
                          tunnel: w2199 -> [_ w2221]
                          tunnel: [FALSE w2220] -> w2198
                          tunnel: [w2210 w2219] -> w2197
                          tunnel: w2196 -> [_ w2218]
                          tunnel: [3 ("y") w2217] -> w2195
                          tunnel: [w2207 w2216] -> w2194
                          tunnel: w2193 -> [w2210 w2215]
                          tunnel: [w2206 w2213] -> w2192
                          tunnel: w2191 -> [w2209 _]
                          tunnel: [w2208 1] -> w2190
                          frame False {
                            n564 = Increment(x=w2209) -> (x+1=w2208:i32)
                          }
                          frame True {
                            n565 = Equal?(x=w2224, y=w2214) -> (x = y?=w2223:bool)
                            n566 = case shown="False" w2223 {
                              tunnel: w2222 -> [w2225 w2236]
                              tunnel: w2221 -> [_ w2240]
                              tunnel: [FALSE w2238] -> w2220
                              tunnel: [w2232 0] -> w2219
                              tunnel: w2218 -> [w2231 _]
                              tunnel: [3 ("y") 3] -> w2217
                              tunnel: [w2225 w2237] -> w2216
                              tunnel: w2215 -> [_ _]
                              tunnel: w2214 -> [w2228 _]
                              tunnel: [w2227 1] -> w2213
                              frame False {
                                n567 = Increment(x=w2228) -> (x+1=w2227:i32)
                                n568 = Add(x=w2231, y=12) -> (x+y=w2232:i32)
                              }
                              frame True {
                                n569 = Equal?(x=w2240, y=w2236) -> (x = y?=w2239:bool)
                                n570 = case shown="True" w2239 {
                                tunnel: [FALSE TRUE] -> w2238
                                tunnel: [w2241 1] -> w2237
                                tunnel: w2236 -> [w2242 _]
                                frame False {
                                n571 = Increment(x=w2242) -> (x+1=w2241:i32)
                                }
                                frame True {
                                }
                                }
                              }
                            }
                          }
                        }
                      }
                    }
                  }
                }
              }
            }
            n572 = Delete From Array(array=w1978, length=1, index=6) -> (deleted portion=w1997:string[], array with subset deleted=w1987:string[])
            n573 = for {
              tunnel: [w2034] -> w1991 mode=indexing
              tunnel: w1987 -> [w2033] mode=indexing
              n574 = Fract/Exp String To Number(string=w2033) -> (number=w2034:dbl)  [unwired: 3 in, 1 out]
            }
            n575 = Index Array(array=w1997) -> (element=w1981:string)  [unwired: 1 in]
            n576 = Index Array(array=w1991, index #1=10 ("index"), index #2=4 ("index"), index #3=5 ("index"), index #4=3 ("index"), index #5=8 ("index")) -> (element #1=w1950:dbl, element #2=w1990:dbl, element #3=w1989:dbl, element #4=w1986:dbl, element #5=w1988:dbl)
            n577 = Equal?(x="B", y=w1981) -> (x = y?=w1984:bool)
            n578 = Equal?(x=w1981, y="b") -> (x = y?=w1985:bool)
            n579 = Not Equal To 0?(x=w1950) -> (x != 0?=w1951:bool)
            n580 = Or(x=w1984, y=w1985) -> (x .or. y?=w1982:bool)
            n581 = xnode "Read/Write Control"("FPGA VI Reference In"=w1948, "CUToff 1"=w1951, "CUToff 2"=w1951) -> ()  [unwired: 1 in, 2 out]
            n582 = call "Lambda to O2.vi"() -> ("O2 %"=w2029:sgl)  [unwired: 1 in]
            n583 = call "Lambda to O2.vi"("Lambda"=w1947) -> ("O2 %"=w2028:sgl)
            n584 = case shown="True" w1982 {
              tunnel: [w2292 w2331] -> _
              tunnel: [w2287 w2325] -> w1955
              tunnel: [w2293 w2330] -> w2030
              tunnel: w1977 -> [w2300 w2333]
              tunnel: w1989 -> [w2299 w2332]
              tunnel: w1990 -> [w2298 w2329]
              tunnel: w1988 -> [w2288 w2313]
              tunnel: [0.0 ("dt (s)") 1.0 ("dt (s)")] -> w2032
              tunnel: w2023 -> [_ w2320]
              tunnel: w1953 -> [_ w2322]
              tunnel: w2022 -> [_ w2321]
              tunnel: w1947 -> [_ w2319]
              tunnel: w1946 -> [w2290 w2317]
              tunnel: w1945 -> [w2289 w2316]
              tunnel: w1986 -> [w2286 w2314]
              frame False {
                # "open loop - not B"
                n585 = case shown="1" w2300 {
                  tunnel: [w2304 0.0 ("dt (s)")] -> w2293
                  tunnel: [0.0 ("dt (s)") w2309] -> w2292
                  tunnel: w2299 -> [_ w2311]
                  tunnel: w2288 -> [w2303 w2310]
                  tunnel: w2298 -> [w2302 _]
                  tunnel: w2290 -> [_ w2307]
                  tunnel: w2289 -> [w2301 _]
                  frame 0, Default {
                    # "HC"
                    n586 = Multiply(x=w2303, y=w2302) -> (x*y=w2306:dbl)
                    n587 = Divide(x=w2306, y=w2301) -> (x/y=w2304:dbl)
                  }
                  frame 1 {
                    # "CO"
                    n588 = Multiply(x=w2310, y=w2311) -> (x*y=w2312:dbl)
                    n589 = Divide(x=w2312, y=w2307) -> (x/y=w2309:dbl)
                  }
                }
                n590 = Multiply(x=w2288, y=w2286) -> (x*y=w2294:dbl)
                n591 = Multiply(x=w2294, y=4.76) -> (x*y=w2296:dbl)
                n592 = Divide(x=w2296, y=100.0) -> (x/y=w2287:dbl)
              }
              frame True {
                # "Baseline B"
                n593 = Multiply(x=w2313, y=w2314) -> (x*y=w2326:dbl)
                n594 = case shown="1" w2333 {
                  tunnel: [w2335 0.0 ("dt (s)")] -> w2330
                  tunnel: [0.0 ("dt (s)") w2342] -> w2331
                  tunnel: w2332 -> [_ w2344]
                  tunnel: w2313 -> [w2337 w2343]
                  tunnel: w2329 -> [w2336 _]
                  tunnel: w2317 -> [_ w2340]
                  tunnel: w2316 -> [w2334 _]
                  frame 0, Default {
                    # "HC loop"
                    n595 = Multiply(x=w2337, y=w2336) -> (x*y=w2338:dbl)
                    n596 = Divide(x=w2338, y=w2334) -> (x/y=w2335:dbl)
                  }
                  frame 1 {
                    # "CO loop"
                    n597 = Multiply(x=w2343, y=w2344) -> (x*y=w2345:dbl)
                    n598 = Divide(x=w2345, y=w2340) -> (x/y=w2342:dbl)
                  }
                }
                n599 = Multiply(x=w2326, y=4.76) -> (x*y=w2328:dbl)
                n600 = Divide(x=w2328, y=100.0) -> (x/y=w2315:dbl)
                n601 = call-poly <vilib>:"PID.vi"("output range"=w2322, "PID gains"=w2320, "process variable"=w2319, "setpoint"=w2321) -> ("output"=w2323:dbl)  [unwired: 6 in, 1 out]
                n602 = Add(x=w2323, y=w2315) -> (x+y=w2325:dbl)
              }
            }
            n603 = case shown="1" "HC INJ CONTROL" {
              tunnel: [w2247 w2268] -> w2031
              tunnel: [w2255 w2267] -> w1954
              tunnel: w2028 -> [w2258 w2275]
              tunnel: w1988 -> [w2257 w2276]
              tunnel: w1944 -> [w2259 w2266]
              tunnel: w2029 -> [w2246 w2274]
              tunnel: w1945 -> [w2256 w2277]
              tunnel: w2030 -> [w2248 w2269]
              tunnel: [sgl 0.0 ("f") w2269] -> w1956
              frame 0, Default {
                # "HC CYCLE CALC - came from here"
                # "Delta O2 %"
                # "HC Injected Upstream Furnace"
                n604 = Subtract(x=w2246, y=w2258) -> (x-y=w2263:sgl)
                n605 = Multiply(x=w2263, y=w2257) -> (x*y=w2264:dbl)
                n606 = Divide(x=w2264, y=sgl 21.0) -> (x/y=w2250:dbl)
                n607 = Absolute Value(x=w2264) -> (abs(x)=w2265:dbl)
                n608 = Divide(x=w2265, y=w2256) -> (x/y=w2262:dbl)
                n609 = Greater Than 0?(x=w2250) -> (x > 0?=w2260:bool)
                n610 = Divide(x=w2262, y=w2259) -> (x/y=w2253:dbl)
                n611 = Select(t=w2250, s=w2260, f=sgl 0.0) -> (s? t:f=w2255:dbl)
                n612 = Select(t=sgl 0.0 ("f"), s=w2260, f=w2253) -> (s? t:f=w2249:dbl)
                n613 = Add(x=w2248, y=w2249) -> (x+y=w2247:dbl)
              }
              frame 1 {
                # "Do we remove AVG 31??"
                # "Delta O2 %"
                # "HC Injection Split"
                n614 = Subtract(x=w2274, y=w2275) -> (x-y=w2282:sgl)
                n615 = Multiply(x=w2282, y=w2276) -> (x*y=w2284:dbl)
                n616 = Divide(x=w2284, y=sgl 21.0) -> (x/y=w2283:dbl)
                n617 = Absolute Value(x=w2284) -> (abs(x)=w2285:dbl)
                n618 = Divide(x=w2285, y=w2277) -> (x/y=w2281:dbl)
                n619 = Greater Than 0?(x=w2283) -> (x > 0?=w2279:bool)
                n620 = Divide(x=w2281, y=w2266) -> (x/y=w2272:dbl)
                n621 = Select(t=w2283, s=w2279, f=sgl 0.0) -> (s? t:f=w2270:dbl)
                n622 = Select(t=sgl 0.0 ("f"), s=w2279, f=w2272) -> (s? t:f=w2271:dbl)
                n623 = call "31pt Mov Avg.vi"("Value in"=w2270) -> ("Value out"=w2267:dbl)  [unwired: 10 in]
                n624 = call "31pt Mov Avg.vi"("Value in"=w2271) -> ("Value out"=w2268:dbl)  [unwired: 10 in]
              }
            }
            n625 = Multiply(x=w2032, y=w2031) -> (x*y=w2027:dbl)
          }
          frame 7 {
            w2346 = 0.0 ("Numeric")
            # "Ageing using model - parametrised"
            # "Ageing Gas From Ageing Array"
            # "HC conc %"
            # "repeats"
            # "no. steps"
            # "ageing gas"
            # "no. subcycles"
            # "no. cycles"
            n626 = Add(x=w2379, y=w2378) -> (x+y=w2396:i32)
            n627 = Increment(x=w2379) -> (x+1=w2406:i32)
            n628 = Delete From Array(array=w2372, length=3, index=0) -> (deleted portion=w2386:string[], array with subset deleted=w2394:string[])
            n629 = Increment(x=w2406) -> (x+1=w2407:i32)
            n630 = Bundle By Name(cluster=T10 {"proportional gain (Kc)"=1.0, "integral time (Ti, min)"=0.1, "derivative time (Td, min)"=0.0} ("Air PID Gains CO 2"), "proportional gain (Kc)"=w2416, "integral time (Ti, min)"=w2415, "derivative time (Td, min)"=w2414) -> (w2417:T10)
            n631 = Index Array(array=w2394, index #1=w2379, index #2=w2406, index #3=w2407) -> (element #1=w2392:string, element #2=w2391:string, element #3=w2390:string)
            n632 = Index Array(array=w2386, index #1=0 ("index"), index #2=1 ("index"), index #3=2 ("index")) -> (element #1=w2388:string, element #2=w2387:string, element #3=w2389:string)
            n633 = Decimal String To Number(string=w2392) -> (number=w2405:i32)  [unwired: 2 in, 1 out]
            n634 = Decimal String To Number(string=w2391) -> (number=w2404:i32)  [unwired: 2 in, 1 out]
            n635 = Decimal String To Number(string=w2390) -> (number=w2403:i32)  [unwired: 2 in, 1 out]
            n636 = Decimal String To Number(string=w2388) -> (number=w2364:i32)  [unwired: 2 in, 1 out]
            n637 = Decimal String To Number(string=w2387) -> (number=w2393:i32)  [unwired: 2 in, 1 out]
            n638 = Decimal String To Number(string=w2389) -> (number=w2402:i32)  [unwired: 2 in, 1 out]
            n639 = Array Subset(array=w2394, index=w2396, length=12) -> (w2398:string[])
            n640 = Index Array(array=w2398, index=0) -> (element=w2397:string)
            n641 = Decimal String To Number(string=w2397) -> (number=w2401:i32)  [unwired: 2 in, 1 out]
            n642 = Equal?(x=w2401, y=w2373) -> (x = y?=w2400:bool)
            n643 = case shown="False" w2400 {
              tunnel: w2378 -> [w2435 w2536]
              tunnel: [w2442 w2535] -> w2370
              tunnel: w2373 -> [w2426 w2516]
              tunnel: [w2437 w2521] -> w2365
              tunnel: w2376 -> [w2431 w2530]
              tunnel: w2374 -> [w2429 w2517]
              tunnel: [w2428 w2520] -> w2366
              tunnel: w2404 -> [w2427 w2533]
              tunnel: w2379 -> [w2430 w2522]
              tunnel: w2375 -> [w2438 w2518]
              tunnel: [w2439 w2524] -> w2367
              tunnel: w2405 -> [w2432 w2531]
              tunnel: [w2440 w2525] -> w2368
              tunnel: w2402 -> [w2433 w2529]
              tunnel: w2377 -> [w2434 w2528]
              tunnel: w2393 -> [w2436 w2527]
              tunnel: [w2441 w2526] -> w2369
              tunnel: [w2443 w2523] -> w2371
              tunnel: [w2445 w2534] -> _
              tunnel: w2403 -> [w2423 w2519]
              tunnel: [w2425 w2514] -> w2349
              tunnel: w2380 -> [w2425 _]
              tunnel: w2398 -> [_ w2514]
              frame False {
                n644 = Decrement(x=w2423) -> (x-1=w2424:i32)
                n645 = Equal?(x=w2424, y=w2426) -> (x = y?=w2444:bool)
                n646 = case shown="True" w2444 {
                  tunnel: w2438 -> [w2447 w2458]
                  tunnel: w2432 -> [_ w2471]
                  tunnel: w2431 -> [w2446 w2469]
                  tunnel: w2433 -> [_ w2468]
                  tunnel: w2434 -> [w2451 w2467]
                  tunnel: w2436 -> [_ w2466]
                  tunnel: [FALSE w2465] -> w2445
                  tunnel: [w2451 w2461] -> w2441
                  tunnel: [w2446 w2459] -> w2440
                  tunnel: [w2447 w2457] -> w2439
                  tunnel: [w2453 w2464] -> w2443
                  tunnel: w2435 -> [w2452 w2463]
                  tunnel: [w2452 w2462] -> w2442
                  tunnel: w2430 -> [w2453 w2460]
                  tunnel: [w2449 0] -> w2437
                  tunnel: w2426 -> [w2450 _]
                  tunnel: w2429 -> [w2448 _]
                  tunnel: [w2448 1] -> w2428
                  tunnel: w2427 -> [_ _]
                  frame False {
                    n647 = Increment(x=w2450) -> (x+1=w2449:i32)
                  }
                  frame True {
                    n648 = Equal?(x=w2471, y=w2458) -> (x = y?=w2470:bool)
                    n649 = case shown="True" w2470 {
                      tunnel: w2469 -> [w2473 w2481]
                      tunnel: w2468 -> [_ w2491]
                      tunnel: w2467 -> [w2474 w2489]
                      tunnel: w2466 -> [_ w2488]
                      tunnel: [FALSE w2487] -> w2465
                      tunnel: [w2477 w2486] -> w2464
                      tunnel: w2463 -> [_ w2485]
                      tunnel: [3 w2484] -> w2462
                      tunnel: [w2474 w2483] -> w2461
                      tunnel: w2460 -> [w2477 w2482]
                      tunnel: [w2473 w2480] -> w2459
                      tunnel: w2458 -> [w2476 _]
                      tunnel: [w2475 1] -> w2457
                      frame False {
                        n650 = Increment(x=w2476) -> (x+1=w2475:i32)
                      }
                      frame True {
                        n651 = Equal?(x=w2491, y=w2481) -> (x = y?=w2490:bool)
                        n652 = case shown="True" w2490 {
                          tunnel: w2489 -> [w2496 w2504]
                          tunnel: w2488 -> [_ w2508]
                          tunnel: [FALSE w2506] -> w2487
                          tunnel: [w2495 0] -> w2486
                          tunnel: w2485 -> [w2493 _]
                          tunnel: [3 ("y") 3] -> w2484
                          tunnel: [w2496 w2505] -> w2483
                          tunnel: w2482 -> [w2492 _]
                          tunnel: w2481 -> [w2499 _]
                          tunnel: [w2498 1] -> w2480
                          frame False {
                            n653 = Increment(x=w2499) -> (x+1=w2498:i32)
                            n654 = Compound Arithmetic op=ADD(w2492, w2493, 12 ("y")) -> (w2495:i32)
                          }
                          frame True {
                            n655 = Equal?(x=w2508, y=w2504) -> (x = y?=w2507:bool)
                            n656 = case shown="True" w2507 {
                              tunnel: [FALSE TRUE] -> w2506
                              tunnel: [w2509 1] -> w2505
                              tunnel: w2504 -> [w2510 _]
                              frame False {
                                n657 = Increment(x=w2510) -> (x+1=w2509:i32)
                              }
                              frame True {
                              }
                            }
                          }
                        }
                      }
                    }
                  }
                }
              }
              frame True {
                n658 = Increment(x=w2516) -> (x+1=w2515:i32)
                n659 = Equal?(x=w2533, y=w2517) -> (x = y?=w2532:bool)
                n660 = case shown="False" w2532 {
                  tunnel: w2536 -> [w2538 w2554]
                  tunnel: [w2537 w2553] -> w2535
                  tunnel: [FALSE w2559] -> w2534
                  tunnel: w2519 -> [_ w2567]
                  tunnel: w2518 -> [w2540 w2565]
                  tunnel: w2531 -> [_ w2564]
                  tunnel: w2530 -> [w2543 w2563]
                  tunnel: w2529 -> [_ w2562]
                  tunnel: w2528 -> [w2544 w2561]
                  tunnel: w2527 -> [_ w2560]
                  tunnel: w2515 -> [w2546 w2548]
                  tunnel: [w2544 w2558] -> w2526
                  tunnel: [w2543 w2557] -> w2525
                  tunnel: [w2540 w2556] -> w2524
                  tunnel: [w2545 w2555] -> w2523
                  tunnel: w2522 -> [w2545 w2552]
                  tunnel: [w2546 w2551] -> w2521
                  tunnel: w2517 -> [w2542 w2549]
                  tunnel: [w2541 w2550] -> w2520
                  frame False {
                    n661 = Increment(x=w2542) -> (x+1=w2541:i32)
                    n662 = Add(x=w2538, y=12) -> (x+y=w2537:i32)
                  }
                  frame True {
                    n663 = Equal?(x=w2567, y=w2548) -> (x = y?=w2566:bool)
                    n664 = case shown="False" w2566 {
                      tunnel: w2565 -> [w2573 w2579]
                      tunnel: w2564 -> [_ w2592]
                      tunnel: w2563 -> [w2574 w2590]
                      tunnel: w2562 -> [_ w2589]
                      tunnel: w2561 -> [w2575 w2588]
                      tunnel: w2560 -> [_ w2587]
                      tunnel: [FALSE w2586] -> w2559
                      tunnel: [w2575 w2582] -> w2558
                      tunnel: [w2574 w2580] -> w2557
                      tunnel: [w2573 w2578] -> w2556
                      tunnel: [w2570 w2585] -> w2555
                      tunnel: w2554 -> [w2569 w2584]
                      tunnel: [w2569 w2583] -> w2553
                      tunnel: w2552 -> [w2570 w2581]
                      tunnel: [w2571 0] -> w2551
                      tunnel: w2548 -> [w2571 _]
                      tunnel: [w2568 w2576] -> w2550
                      tunnel: w2549 -> [w2568 w2576]
                      frame False {
                      }
                      frame True {
                        n665 = Equal?(x=w2592, y=w2579) -> (x = y?=w2591:bool)
                        n666 = case shown="False" w2591 {
                          tunnel: w2590 -> [w2594 w2602]
                          tunnel: w2589 -> [_ w2612]
                          tunnel: w2588 -> [w2595 w2610]
                          tunnel: w2587 -> [_ w2609]
                          tunnel: [FALSE w2608] -> w2586
                          tunnel: [w2598 w2607] -> w2585
                          tunnel: w2584 -> [_ w2606]
                          tunnel: [3 ("y") w2605] -> w2583
                          tunnel: [w2595 w2604] -> w2582
                          tunnel: w2581 -> [w2598 w2603]
                          tunnel: [w2594 w2601] -> w2580
                          tunnel: w2579 -> [w2597 _]
                          tunnel: [w2596 1] -> w2578
                          frame False {
                            n667 = Increment(x=w2597) -> (x+1=w2596:i32)
                          }
                          frame True {
                            n668 = Equal?(x=w2612, y=w2602) -> (x = y?=w2611:bool)
                            n669 = case shown="False" w2611 {
                              tunnel: w2610 -> [w2613 w2624]
                              tunnel: w2609 -> [_ w2628]
                              tunnel: [FALSE w2626] -> w2608
                              tunnel: [w2620 0] -> w2607
                              tunnel: w2606 -> [w2619 _]
                              tunnel: [3 ("y") 3] -> w2605
                              tunnel: [w2613 w2625] -> w2604
                              tunnel: w2603 -> [_ _]
                              tunnel: w2602 -> [w2616 _]
                              tunnel: [w2615 1] -> w2601
                              frame False {
                                n670 = Increment(x=w2616) -> (x+1=w2615:i32)
                                n671 = Add(x=w2619, y=12) -> (x+y=w2620:i32)
                              }
                              frame True {
                                n672 = Equal?(x=w2628, y=w2624) -> (x = y?=w2627:bool)
                                n673 = case shown="False" w2627 {
                                tunnel: [FALSE TRUE] -> w2626
                                tunnel: [w2629 1] -> w2625
                                tunnel: w2624 -> [w2630 _]
                                frame False {
                                n674 = Increment(x=w2630) -> (x+1=w2629:i32)
                                }
                                frame True {
                                }
                                }
                              }
                            }
                          }
                        }
                      }
                    }
                  }
                }
              }
            }
            n675 = Delete From Array(array=w2349, length=1, index=6) -> (deleted portion=w2352:string[], array with subset deleted=w2354:string[])
            n676 = for {
              tunnel: [w2422] -> w2353 mode=indexing
              tunnel: w2354 -> [w2421] mode=indexing
              n677 = Fract/Exp String To Number(string=w2421) -> (number=w2422:dbl)  [unwired: 3 in, 1 out]
            }
            n678 = Index Array(array=w2352) -> (element=w2358:string)  [unwired: 1 in]
            n679 = Index Array(array=w2353, index #1=4 ("index"), index #2=5 ("index"), index #3=3 ("index"), index #4=8 ("index")) -> ()  [unwired: 4 out]
            n680 = Equal?(x="B", y=w2358) -> (x = y?=w2356:bool)
            n681 = Equal?(x=w2358, y="b") -> (x = y?=w2355:bool)
            n682 = Or(x=w2356, y=w2355) -> (x .or. y?=w2348:bool)
            n683 = case shown="True" w2348 {
              tunnel: [w2640 w2672] -> _
              tunnel: [w2641 w2671] -> _
              tunnel: 0.0 ("y") -> [w2644 w2673]
              tunnel: 0.0 ("y") -> [w2643 w2670]
              tunnel: 0.0 ("y") -> [w2642 w2669]
              tunnel: 0.0 -> [w2636 w2668]
              tunnel: [0.0 ("dt (s)") 1.0 ("dt (s)")] -> _
              tunnel: w2417 -> [_ w2663]
              tunnel: w2347 -> [_ w2665]
              tunnel: w2419 -> [_ w2664]
              tunnel: w2420 -> [_ w2662]
              tunnel: 0.0 ("Numeric") -> [w2638 w2661]
              tunnel: 0.0 ("Numeric") -> [w2637 w2660]
              tunnel: [0.0 w2659] -> _
              tunnel: w2364 -> [w2635 w2658]
              frame False {
                n684 = case shown="1" w2635 {
                  tunnel: [w2648 0.0 ("dt (s)")] -> w2641
                  tunnel: [0.0 ("dt (s)") w2653] -> w2640
                  tunnel: w2644 -> [_ w2655]
                  tunnel: w2636 -> [w2647 w2654]
                  tunnel: w2643 -> [w2646 _]
                  tunnel: w2642 -> [_ _]
                  tunnel: w2638 -> [_ w2651]
                  tunnel: w2637 -> [w2645 _]
                  frame 0, Default {
                    # "HC"
                    n685 = Multiply(x=w2647, y=w2646) -> (x*y=w2650:dbl)
                    n686 = Divide(x=w2650, y=w2645) -> (x/y=w2648:dbl)
                  }
                  frame 1 {
                    # "CO"
                    n687 = Multiply(x=w2654, y=w2655) -> (x*y=w2656:dbl)
                    n688 = Divide(x=w2656, y=w2651) -> (x/y=w2653:dbl)
                  }
                }
              }
              frame True {
                # "Baseline B"
                n689 = case shown="1" w2658 {
                  tunnel: [w2675 0.0 ("dt (s)")] -> w2671
                  tunnel: [0.0 ("dt (s)") w2682] -> w2672
                  tunnel: w2673 -> [_ w2684]
                  tunnel: w2668 -> [w2677 w2683]
                  tunnel: w2670 -> [w2676 _]
                  tunnel: w2669 -> [_ _]
                  tunnel: w2661 -> [_ w2680]
                  tunnel: w2660 -> [w2674 _]
                  frame 0, Default {
                    # "HC loop"
                    n690 = Multiply(x=w2677, y=w2676) -> (x*y=w2678:dbl)
                    n691 = Divide(x=w2678, y=w2674) -> (x/y=w2675:dbl)
                  }
                  frame 1 {
                    # "CO loop"
                    n692 = Multiply(x=w2683, y=w2684) -> (x*y=w2685:dbl)
                    n693 = Divide(x=w2685, y=w2680) -> (x/y=w2682:dbl)
                  }
                }
                n694 = call-poly <vilib>:"PID.vi"("output range"=w2665, "PID gains"=w2663, "process variable"=w2662, "setpoint"=w2664) -> ("output"=w2666:dbl)  [unwired: 6 in, 1 out]
                n695 = Add(x=w2666, y=0.0) -> (x+y=w2659:dbl)
              }
            }
          }
        }
      }
    }
    n696 = call "Valve_SP.vi"("Valve 1 SP"=w1463) -> ("Output"=w1467:u8[])  [unwired: 10 in]
    n697 = call "Valve_SP.vi"("Valve 1 SP"=w1464) -> ("Output"=w1466:u8[])  [unwired: 10 in]
    n698 = local read "MFC SV Array"() -> (w1506:bool[])
    n699 = Build Array(w1517, w1539, w1610, w1609, w1540, w1608, w1538, w1518) -> (w1557:dbl[])
    n700 = Build Array (concatenate)(w1466, w1467) -> (w1465:u8[])
    n701 = call "MFR Flow to SP 2-2_RS232.vi"("MFC SPs"=w1557) -> ("MFC array"=w1480:u8[], "SV Array"=w1507:bool[])  [unwired: 9 in]
    n702 = Build Array (concatenate)(w1560, w1557, w1523, w1524, w1455) -> (w1558:dbl[])
    n703 = Build Array (concatenate)(w1480, w1465) -> (w1479:u8[])
    n704 = shared-variable "RT CompactRIO Target 2\\Library 1.lvlib\\DATA_2"(w1558) -> ()  [unwired: 1 in, 1 out]
    n705 = call "MFC_SV_Combined.vi"("SV Array 1Hz"=w1506, "SV Array 5Hz"=w1507) -> ("SV Full MFC"=w1505:bool[])  [unwired: 9 in]
    n706 = xnode "Read/Write Control"("FPGA VI Reference In"=w1462, "MFC Array Out"=w1479, "DO SV Array Out"=w1505) -> ()  [unwired: 1 in, 2 out]
    n707 = node-c288() -> ()  [unwired: 1 in, 1 out]
  }
  n708 = node-c288(w11) -> ()  [unwired: 1 out]
  n709 = node-c288(w3) -> ()  [unwired: 1 out]
  n710 = node-c288(w17) -> ()  [unwired: 1 out]
  n711 = node-c288(w38) -> ()  [unwired: 1 out]
  n712 = node-c288(w46) -> ()  [unwired: 1 out]
  n713 = xnode "Close FPGA VI Reference"("FPGA VI Reference In"=w22, "error in"=w21) -> ("error out"=→"error out":errorcluster)
